vi "01 Dryer_Performance_SM.vi"() -> ()   [LabVIEW 2016]
uses:
  Utility/Save File/File Setup (Public)/DPT Global Test Variables.vi
  Utility/Save File/File Setup.lvlib
  Type Definitions/RMC Calc Inputs.ctl
  Nufi/Nufi Global_ReceivedDataCluster.vi
  Type Definitions/Q Dryer Data.ctl
  Drivers/Yokogawa WT500/Type Definitions/WT500 Sequences.ctl
  Drivers/Chroma 617xx/Type Definition/Chroma Driver Select.ctl
  Type Definitions/Equipment DPT.ctl
  <vilib>/Analysis/NI_AALBase.lvlib
  <vilib>/Analysis/baseanly.llb/Mean (DBL).vi
  Utility/Type Definitions/UTILITY Power Inputs Control.ctl
  Utility/Custom Pallet Controls/Custom Pallet DBL.ctl
  <vilib>/Platform/fileVersionInfo.llb/FileVersionInformation.ctl
  Utility/Save File/File Setup (Public)/Type Definition/DPT Global Type.ctl
  Utility/Type Definitions/UTILITY Power Analyzer.ctl
  Utility/Custom Pallet Controls/Custom Pallet Quit.ctl
  Utility/Custom Pallet Controls/Custom Pallet Timer.ctl
  Utility/Save File/File Setup (Public)/Type Definition/DPT Output Dryer Information.ctl
  Utility/Custom Pallet Controls/Custom Pallet Configuration.ctl
  Utility/Custom Pallet Controls/Custom Pallet Reverse.ctl
  Utility/Custom Pallet Controls/Custom Pallet String.ctl
  Utility/Custom Pallet Controls/Custom Pallet Chart.ctl
  Drivers/cDAQ/Type Definitions/cDAQ Setup.ctl
panel:
  out "cDAQ Data Out":string[](array[string])
  out "Indexes used":i32[](array[numeric])
  in  "Setup":T1={"Test Setup"={"RH Resistor"=100.0, "Temp Resistor"=100.0, "Gas P. Resistor"=250.0, "Temp4mA Val"=32.0, "Temp20mA Val"=212.0, "RH4mA Val"=0.0, "RH20mA Val"=100.0, "GPres4mA Val"=0.0, "Gpres20mA Val"=50.0}, "cDAQ Array Locations"={"Scale Channel"=90, "TC Channels"=0, "VDC Discrete Channel"=72, "RH Chan"=91, "Temp Chan"=93, "Tscale Channel"=2, "RDB Channel"=0, "Gas Temperature"=88, "Gas Pressure"=89, "Barometric Pressure"=94, "Gas Feedback Chan"=92}}
  in  "Weight Offset 2":dbl
  in  "W.Samps 2":i32=10
  out "Status Message":T2
  in  "Back Button":T3
  in  "Settings":T4
  in  "End Test":T5
  out "2015 array":string[][](array[string])
  out "FileInit Cluster":T6={"Dryer Type"="NR", "TR Number"="", "Lab ID"="", "Output Stream Header"=[], "Stream Data Output"=[], "2015 Array"=[], "Dryer Test Data"=[], "Off Mode Array"=[], "Calibration Array"=[], "File Initialization Array"=[], "Load Run Number"="", "Model:"="DGnn", "Serial Number:"="DGnn", "Build:"="", "Test_Title Per TR:"="HeatUP", "Ambient Temp SetPoint:"="70", "Washer Water \nTemperature ( 60 ± 5°F ):"="60", "Frequency:"="60 HZ", "Dryness Setting:"="", "Heat Setting:"="", "Ambient RH:"="50", "Drying Cycle:"="", "Exhaust:"="NR", "Comments:"="", "Technician:"="", "Engineer:"="CraigT.", "Water Hardness (PPM)"="60", "Empty Dryer Cold Weight"="HeatUP", "Date:"="DGnn", "Version:"="DGnn", "Computer:"="1A", "Load Type"="", "Nominal Load  Weight"="", "Weights Out"={"Measured IMC"=7.0, "Actual RMC"=7.0, "RMC (Desired)"=100.0, "Bone Dry Wt(lbs)"=7.0, "Tolerance(%)"=5.0}, "Test Station:"="1A", "Heat Setting:"="", "Dryness Setting:"="", "Frequency:"="60 HZ", "Water Hardness (PPM)"="60", "Washer Water \nTemperature ( 60 ± 5°F )"="60", "Flow Computer Info Baro,BTUF,u,Z"=[], "Filename"="", "Analog Voltage Data"=[]} {"Weights Out"."Tolerance(%)" format="%0#_6g"; "Weights Out"."Bone Dry Wt(lbs)" format="%03_6g"; "Weights Out"."RMC (Desired)" format="%0#_6g"; "Weights Out"."Actual RMC" format="%03_6g"; "Weights Out"."Measured IMC" format="%0#_6g"}
  out "Plot Power":cluster{dbl[], dbl[]}[](graph)
  in  "Quit":T5
  out "Power Out":T7={"Yokogawa"={"WT210"={"Sample Rate (1: 0.25s)"=1, "A Range (12: 20A)"=11, "V Range (6: 600V)"=4, "Power VISA Yokogawa WT210"=""}, "WT500"={"Power VISA Yokogawa WT500"="", "V Range (8: 1000V)"=6, "I Range (7: 40A)"=7, "Update Rate (3: 500ms)"=2}}, "Aplus"={"Aplus IP Address"="192.168.1.101", "Remote Port"=502, "Instrument"="APLUS", "Instr Driver Revision"="1.03.0053"}, "Power Limits"={"Crest Factor"={"Upper Limit"=1.49, "Lower Limit"=1.34}, "Harmonic Content"={"Uthd"=2.0}, "Voltage"={"% Error"=2.0}, "Stability"={"<1 Watt "={"Wattage"=1.0, "Slope (mW/H)"=10.0}, ">1 Watt"={"1%Power/Hour"=1.0}}}, "Nominal Voltage"=120, "Time Limit (s)"=10800.0, "Power Variation Limit (%)"=50.0, "Power Supply"={"Chroma 61605"="CHROMA", "Use Chroma?"=FALSE}} {"Yokogawa"."WT500"."Update Rate (3: 500ms)" items=["-", "100ms", "200ms", "500ms", "1s", "2s", "5s"]; "Yokogawa"."WT500"."I Range (7: 40A)" items=["AUTO", "500 mA", "1 A", "2 A", "5 A", "10 A", "20 A", "40 A", "S-AUTO", "50 mV", "100 mV", "200 mV", "500 mV", "1 V", "2 V", "5 V", "10 V", "250 mA", "500 mA", "1 A", "2.5 A", "5 A", "10 A", "20 A", "25 mV", "50 mV", "100 mV", "250 mV", "500 mV", "1 V", "2.5 V", "5 V"]; "Yokogawa"."WT500"."V Range (8: 1000V)" items=["AUTO", "15", "30", "60", "100", "150", "300", "600", "1000", "7.5", "15", "30", "50", "75", "150", "300", "500"]; "Yokogawa"."WT210"."V Range (6: 600V)" items=["Auto", "15V", "30V", "60V", "150V", "300V", "600V"]; "Yokogawa"."WT210"."A Range (12: 20A)" items=["Auto", "5mA", "10mA", "20mA", "50mA", "100mA", "200mA", "0.5A", "1A", "2A", "5A", "10A", "20A", "50mV", "100mV", "200mV", "2.5V", "5V", "10V"]; "Yokogawa"."WT210"."Sample Rate (1: 0.25s)" items=["0.1s", "0.25s", "0.5s", "1s", "2s", "5s"]}
  in  "Voltage Stream Header Output":string[][](array[string])
  in  "Stream Data":string[][](array[string])
  in  "Tab Control 3":enum32{"Page 1", "Page 2", "Page 3", "Page 4"}(tab)
  out "Equipment":T8={"Scale Com Port"="", "Com Flow Computer"="", "Com Power Meter"="", "Com Power Supply"="", "Power "={"Yokogawa"={"WT210"={"Sample Rate (1: 0.25s)"=1, "A Range (12: 20A)"=11, "V Range (6: 600V)"=4, "Power VISA Yokogawa WT210"=""}, "WT500"={"Power VISA Yokogawa WT500"="", "V Range (8: 1000V)"=6, "I Range (7: 40A)"=7, "Update Rate (3: 500ms)"=2}}, "Aplus"={"Aplus IP Address"="192.168.1.101", "Remote Port"=502, "Instrument"="APLUS", "Instr Driver Revision"="1.03.0053"}, "Power Limits"={"Crest Factor"={"Upper Limit"=1.49, "Lower Limit"=1.34}, "Harmonic Content"={"Uthd"=2.0}, "Voltage"={"% Error"=2.0}, "Stability"={"<1 Watt "={"Wattage"=1.0, "Slope (mW/H)"=10.0}, ">1 Watt"={"1%Power/Hour"=1.0}}}, "Nominal Voltage"=120, "Time Limit (s)"=10800.0, "Power Variation Limit (%)"=50.0, "Power Supply"={"Chroma 61605"="CHROMA", "Use Chroma?"=FALSE}}} {"Power"."Yokogawa"."WT500"."Update Rate (3: 500ms)" items=["-", "100ms", "200ms", "500ms", "1s", "2s", "5s"]; "Power"."Yokogawa"."WT500"."I Range (7: 40A)" items=["AUTO", "500 mA", "1 A", "2 A", "5 A", "10 A", "20 A", "40 A", "S-AUTO", "50 mV", "100 mV", "200 mV", "500 mV", "1 V", "2 V", "5 V", "10 V", "250 mA", "500 mA", "1 A", "2.5 A", "5 A", "10 A", "20 A", "25 mV", "50 mV", "100 mV", "250 mV", "500 mV", "1 V", "2.5 V", "5 V"]; "Power"."Yokogawa"."WT500"."V Range (8: 1000V)" items=["AUTO", "15", "30", "60", "100", "150", "300", "600", "1000", "7.5", "15", "30", "50", "75", "150", "300", "500"]; "Power"."Yokogawa"."WT210"."V Range (6: 600V)" items=["Auto", "15V", "30V", "60V", "150V", "300V", "600V"]; "Power"."Yokogawa"."WT210"."A Range (12: 20A)" items=["Auto", "5mA", "10mA", "20mA", "50mA", "100mA", "200mA", "0.5A", "1A", "2A", "5A", "10A", "20A", "50mV", "100mV", "200mV", "2.5V", "5V", "10V"]; "Power"."Yokogawa"."WT210"."Sample Rate (1: 0.25s)" items=["0.1s", "0.25s", "0.5s", "1s", "2s", "5s"]}
  in  "Power Analyzer":T9=enum."WT500"
  in  "Data Save Array":string[][](array[string])
  out "Off Mode Power Output":string[][](array[string])
  out "Error after create directory":errorcluster
  out "Error after save to excel":errorcluster
  out "Error before create directory":errorcluster
  out "Error":errorcluster[](array[cluster])
  out "Tsamp(s)":dbl
  in  "Tab Control":T10(tab)
  out "Wbouy":dbl
  out "Plot RMC":cluster{dbl[], dbl[]}[](graph)
  out "Experimental Completion Time Estimate":dbl format="%<%H:%M:%S>t"
  out "RMC Chart":T11
  out "Watt Chart":dbl(graph)
  out "Relative Moisture Content (%)":T12 format="%.2f"
  out "Scale Weight (lbs)":T12 format="%.2f"
  out "RDB Temperature (Degrees F)":T12 format="%.2f"
  out "Room Ambient (Degrees F)":T12 format="%.2f"
  out "Cloth Weight Estimate (lbs)":T12 format="%.2f"
  out "Wet Clothing Weight (lbs)":T12 format="%.2f"
  out "Empty Dryer Cold Weight (lbs)":T12 format="%.2f"
  out "Bone Dry Weight (lbs)":T12 format="%.2f"
  out "Watt Hours (Wh)":T12 format="%.2f"
  out "Power (Watts)":T12 format="%.2f"
  out "Current L2 (A)":T12 format="%.2f"
  out "Current L1 (A)":T12 format="%.2f"
  out "Power ON":bool
  out "Description":string="Dryer Performance Test"
  out "Test Time":T13 format="%<%H:%M:%S>t"
  in  "Tab Control 2":enum32{"Debug Only", "Running"}(tab)
  in  "Debug Info":T14(tab)=enum."Settings"
  out "FileName DataLog":path caption="FileName"
  out "FileVersionInfo Out":T15
  out "Ver.":string="Development"
  out "Work File Directory":path=path "c:/Work"
  in  "Close when complete":bool
  in  "Standby Power Settings":path=path "C:/work/Standby Power Settings.csv"
  in  "Excel Template Path":path=path "C:/work/DOE Calculation Template for 2015 DOE ETP Rev4.xlsx"
  out "Created File Path":path
  in  "Error Log 2":errorcluster[](array[cluster])
  out "Power Off Check":bool[](array[boolean])
  out "error out":errorcluster
  out "Error Count":dbl
  out "# elements in queue":i32
  out "Error Log":errorcluster[](array[cluster])
  out "Data Filename":string
  out "Power Off Time(samples)":i32=15
  in  "UI Timer":i32=1000
  in  "DAQ Timer":i32=1000
  in  "Clear Graph":bool
  out "Use SL9200 Gas Readings?":bool
  in  "Simulate":bool
  in  "Supply Voltage:":string(combo)
  out "Time Limit(s)":dbl=5400.0 format="%<%H:%M:%S>t"
  out "RMC Limit":dbl=2.0
  out "Enable Time Limit":bool
  out "Enable RMC Limit":bool
  in  "MA Filter Size":i32=10
  in  "Power On Threshold":dbl=50.0
  in  "Scale Temp Coeff":dbl
  out "Init Scale Temp":dbl=72.0
  out "Use Dry Gas Meter?":bool=TRUE
  out "Load Offset":dbl
  in  "Drum Volume":dbl=6.0
  out "Enable Stop On Power Off":bool=TRUE
  out "exe?":bool
  out "RMC Calc Inputs":T16
  out "Tend?":dbl format="%<%H:%M:%S>t"
  out "Scale Com Port":refnum<visa-resource-name>="COM1"
  out "ITHX RH Sensor":bool
  out "Offset":dbl
  out "Init Offset Coeff":dbl
  in  "Power off Check RMC sec":dbl=5.0
  out "DAQ Delay Time":i32
  out "Data Process RMC Counter":dbl
  out "L1 Adjusted":string
  out "L2 Adjusted":string
  out "Debug Mode":bool=TRUE
  out "Debug List Test States":string[](array[string])
  out "daq debug array":string[](array[string])
  out "UI States":string[](array[string])
  out "End1_Main":bool=TRUE
  out "Write to File":bool=TRUE
  out "Test Complete?":bool
  out "Loggin Data":bool
  out "End2_DAQ":bool=TRUE
  out "Eng3_Log":bool=TRUE
  out "BTUF3":string[][](array[string])
  out "Power On One Shot":bool
  out "End Msg":string
  out "Final User Message":string="Premature Completion."
  out "cDAQ":bool=TRUE
  in  "cDAQ Setting":bool=TRUE
  out "End_End":bool=TRUE
  in  "CDAQ Tasks":refnum<k21>[](array[refnum])
  out "[Temp (F), RH]":dbl[](array[numeric])
  out "Power Off One Shot":bool
  out "Elapsed Time":T13 format="%<%H:%M:%S>t"
  out "Start Time (sec)":T13 format="%<%H:%M:%S>t"
  out "Power >Threshold":bool
  out "TC Channel List":string
  out "DAQ Channel List":string
  out "DAQ Label List":string[](array[string])
  in  "Get Data Interrupt":bool
  out "Use Chroma":bool
  out "Number of TCs":i32
  out "Stream DC to File?":bool
  out "Globals for Dryer Performance Test":T17={"Test Setup"={"RH Resistor"=267.4, "Temp Cal"=72.0, "Temp Coeff"=-0.0234, "Power On Threshold"=50.0, "MA Filter Size"=60, "Weight Offset"=0.0, "Temp Resistor"=267.4, "Gas Enabled"=FALSE, "Gas P. Resistor"=250.0, "Scale Com"=1.0, "W. Samps"=5, "Temp4mA Val"=267.4, "Temp20mA Val"=267.4, "RH4mA Val"=0.0, "RH20mA Val"=100.0, "GPres4mA Val"=0.0, "Gpres20mA Val"=50.0, "Smoothing"=FALSE, "CDAQ"=FALSE, "34970"=FALSE, "34980"=FALSE, "RH-IP"="192.168.1.161", "RH-IP2"="192.168.1.161", "RH-IP3"="192.168.1.161", "CompVolume"=0.0, "T45_Coeff."=0.0}, "Agilent Setup"={"Scale Channel"="3009", "TC Channels"="1001:1040,2001:2040", "VDC Discrete Channels"="3001:3008", "RH Chan"="3010,3011", "Temp Chan"="3010,3011", "Tscale Channel"="", "RDB Channel"="1001", "Gas Temperature"="1019", "Gas Pressure"="1020", "Barometric Pressure"="1040", "Gas Feedback Chan"="3012"}, "Directories"={"Work File Directory"=path "c:/Work", "Save File Directory"=path "c:/Data", "Library Directory"=path "c:/Data", "Data Backup Directory"=path "c:/Data", "Data Backup Dir Fail"=path "c:/Data", "Lab Directory"=path "c:/Data"}, "Test Information"={"Model:"="DGnn", "Temperature:"="Mode: EHEAT", "Engineer:"="CraigT.", "Technician:"="RonR.", "Comments:"="R134A Charge Level: 50g", "Lab ID:"="DGnn", "TR Number:"="T000000", "Test Number:"="T000000", "Test Station:"="Unitialized", "Empty Dryer Cold Weight:"=0.0, "Serial Number:"="DGnn", "Build:"="DGnn", "Dryer Type"="RonR.", "Humidity"="70,50", "Test Title per TR:"="70,50"}, "cDAQ Array Locations"={"Scale Channel"="90", "TC Channels"="1-15, 65,66,67\n16-31, 68,69\n32-47, 70,71\n48-64, 72, 73", "VDC Discrete Channel"="1020,1040,3001:3008", "RH Chan"="91", "Temp Chan"="93", "Tscale Channel"="3", "RDB Channel"="1", "Gas Temperature"="0", "Gas Pressure"="89", "Barometric Pressure"="94", "Gas Feedback Chan"="92"}}
  out "Plot All":cluster{dbl[], dbl[]}[](graph)
  in  "Apply Load Offset":bool
  out "Use Smoothing":bool=TRUE
  out "2015?":bool
  out "Data":string[][](array[string])
  in  "Plot Legend":T18(array[cluster])
  in  "None":bool
  in  "All":bool
  out "Power Label":string[](array[string])=["VL1", "VL2", "IL1", "IL2", "P", "WH", "Ipeak", "Phi(1,2)"]
  out "Q Element":T19
  in  "Start Test":bool
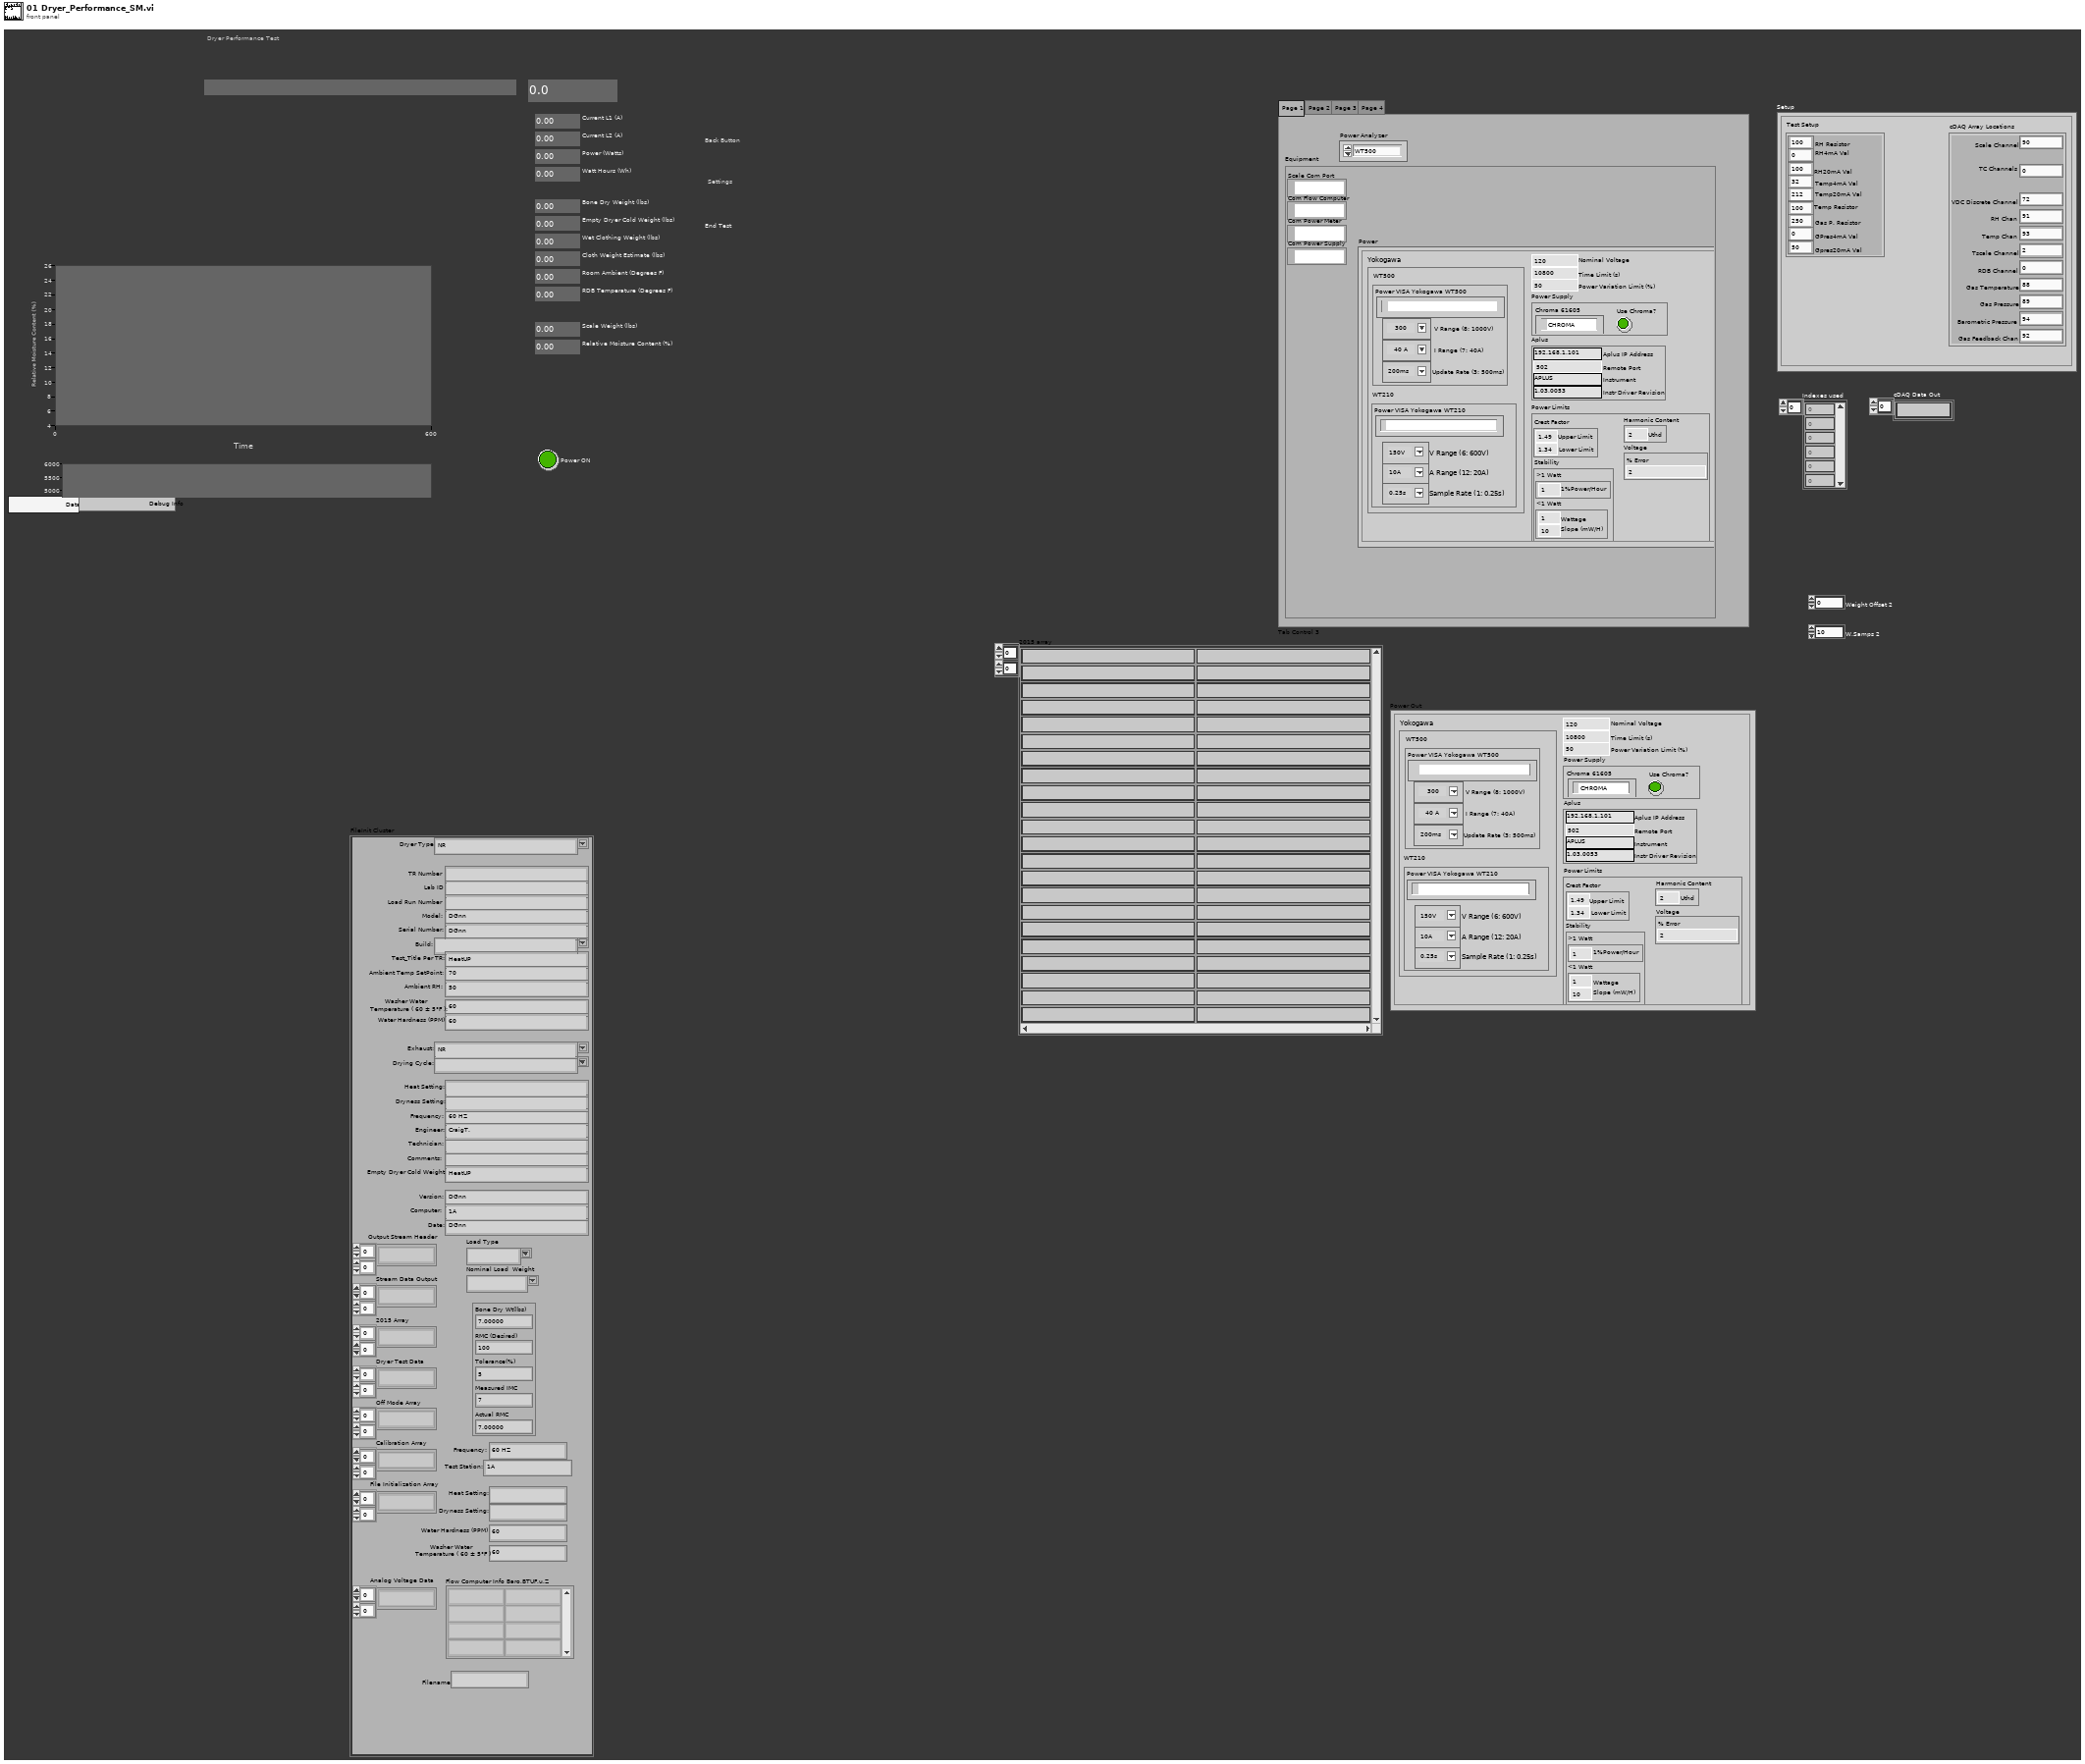
[diagram p1: front panel]
types:
  T1 = typedef "cDAQ Setup.ctl" = cluster{"Test Setup":cluster{"RH Resistor":dbl, "Temp Resistor":dbl, "Gas P. Resistor":dbl, "Temp4mA Val":dbl, "Temp20mA Val":dbl, "RH4mA Val":dbl, "RH20mA Val":dbl, "GPres4mA Val":dbl, "Gpres20mA Val":dbl}, "cDAQ Array Locations":cluster{"Scale Channel":i32, "TC Channels":i32, "VDC Discrete Channel":i32, "RH Chan":i32, "Temp Chan":i32, "Tscale Channel":i32, "RDB Channel":i32, "Gas Temperature":i32, "Gas Pressure":i32, "Barometric Pressure":i32, "Gas Feedback Chan":i32}}
  T2 = typedef "Custom Pallet String.ctl" = string
  T3 = typedef "Custom Pallet Reverse.ctl" = bool
  T4 = typedef "Custom Pallet Configuration.ctl" = bool
  T5 = typedef "Custom Pallet Quit.ctl" = bool
  T6 = typedef "File Setup.lvlib/DPT Output Dryer Information.ctl" = cluster{"Dryer Type":string, "TR Number":string, "Lab ID":string, "Output Stream Header":string[][], "Stream Data Output":string[][], "2015 Array":string[][], "Dryer Test Data":string[][], "Off Mode Array":string[][], "Calibration Array":string[][], "File Initialization Array":string[][], "Load Run Number":string, "Model:":string, "Serial Number:":string, "Build:":string, "Test_Title Per TR:":string, "Ambient Temp SetPoint:":string, "Washer Water \nTemperature ( 60 ± 5°F ):":string, "Frequency:":string, "Dryness Setting:":string, "Heat Setting:":string, "Ambient RH:":string, "Drying Cycle:":string, "Exhaust:":string, "Comments:":string, "Technician:":string, "Engineer:":string, "Water Hardness (PPM)":string, "Empty Dryer Cold Weight":string, "Date:":string, "Version:":string, "Computer:":string, "Load Type":string, "Nominal Load  Weight":string, "Weights Out":cluster{"Measured IMC":dbl, "Actual RMC":dbl, "RMC (Desired)":dbl, "Bone Dry Wt(lbs)":dbl, "Tolerance(%)":dbl}, "Test Station:":string, "Heat Setting:":string, "Dryness Setting:":string, "Frequency:":string, "Water Hardness (PPM)":string, "Washer Water \nTemperature ( 60 ± 5°F )":string, "Flow Computer Info Baro,BTUF,u,Z":string[][], "Filename":string, "Analog Voltage Data":string[][]}
  T7 = typedef "UTILITY Power Inputs Control.ctl" = cluster{"Yokogawa":cluster{"WT210":cluster{"Sample Rate (1: 0.25s)":i32, "A Range (12: 20A)":i32, "V Range (6: 600V)":i32, "Power VISA Yokogawa WT210":refnum<visa-resource-name>}, "WT500":cluster{"Power VISA Yokogawa WT500":refnum<visa-resource-name>, "V Range (8: 1000V)":i32, "I Range (7: 40A)":i32, "Update Rate (3: 500ms)":i32}}, "Aplus":cluster{"Aplus IP Address":string, "Remote Port":i32, "Instrument":string, "Instr Driver Revision":string}, "Power Limits":cluster{"Crest Factor":cluster{"Upper Limit":dbl, "Lower Limit":dbl}, "Harmonic Content":cluster{"Uthd":dbl}, "Voltage":cluster{"% Error":dbl}, "Stability":cluster{"<1 Watt ":cluster{"Wattage":dbl, "Slope (mW/H)":dbl}, ">1 Watt":cluster{"1%Power/Hour":dbl}}}, "Nominal Voltage":i32, "Time Limit (s)":dbl, "Power Variation Limit (%)":dbl, "Power Supply":cluster{"Chroma 61605":refnum<visa-resource-name>, "Use Chroma?":bool}}
  T8 = typedef "Equipment DPT.ctl" = cluster{"Scale Com Port":refnum<visa-resource-name>, "Com Flow Computer":refnum<visa-resource-name>, "Com Power Meter":refnum<visa-resource-name>, "Com Power Supply":refnum<visa-resource-name>, "Power ":T7}
  T9 = typedef "UTILITY Power Analyzer.ctl" = enum16{"", "APLUS", "WT210", "WT500", "WT300", "OSI", "Debug", "WT230"}
  T10 = enum32{"                           Data  ", "                                  Debug Info"}
  T11 = typedef "Custom Pallet Chart.ctl" = dbl
  T12 = typedef "Custom Pallet DBL.ctl" = dbl
  T13 = typedef "Custom Pallet Timer.ctl" = dbl
  T14 = enum32{"File Info", "Error Data", "Settings", "Test States", "NI CDAQ Data", "Globals"}
  T15 = typedef "FileVersionInformation.ctl" = cluster{"FileVersion":string, "ProductName":string, "InternalName":string, "CompanyName":string, "LegalCopyright":string, "FileDescription":string}
  T16 = typedef "RMC Calc Inputs.ctl" = cluster{"Measeured Weight":dbl, "BDW - Bone Dry Wt(lbs)":dbl, "Empty Dryer Cold Weight":dbl, "Measured IMC":dbl, "Tamb":dbl, "T-RDB":dbl, "Drum Volume":dbl, "Load Offset":dbl, "Temp Coeff":dbl, "Temp Cal":dbl, "Tscale":dbl}
  T17 = typedef "File Setup.lvlib/DPT Global Type.ctl" = cluster{"Test Setup":cluster{"RH Resistor":dbl, "Temp Cal":dbl, "Temp Coeff":dbl, "Power On Threshold":dbl, "MA Filter Size":i32, "Weight Offset":dbl, "Temp Resistor":dbl, "Gas Enabled":bool, "Gas P. Resistor":dbl, "Scale Com":dbl, "W. Samps":i32, "Temp4mA Val":dbl, "Temp20mA Val":dbl, "RH4mA Val":dbl, "RH20mA Val":dbl, "GPres4mA Val":dbl, "Gpres20mA Val":dbl, "Smoothing":bool, "CDAQ":bool, "34970":bool, "34980":bool, "RH-IP":string, "RH-IP2":string, "RH-IP3":string, "CompVolume":dbl, "T45_Coeff.":dbl}, "Agilent Setup":cluster{"Scale Channel":string, "TC Channels":string, "VDC Discrete Channels":string, "RH Chan":string, "Temp Chan":string, "Tscale Channel":string, "RDB Channel":string, "Gas Temperature":string, "Gas Pressure":string, "Barometric Pressure":string, "Gas Feedback Chan":string}, "Directories":cluster{"Work File Directory":path, "Save File Directory":path, "Library Directory":path, "Data Backup Directory":path, "Data Backup Dir Fail":path, "Lab Directory":path}, "Test Information":cluster{"Model:":string, "Temperature:":string, "Engineer:":string, "Technician:":string, "Comments:":string, "Lab ID:":string, "TR Number:":string, "Test Number:":string, "Test Station:":string, "Empty Dryer Cold Weight:":dbl, "Serial Number:":string, "Build:":string, "Dryer Type":string, "Humidity":string, "Test Title per TR:":string}, "cDAQ Array Locations":cluster{"Scale Channel":string, "TC Channels":string, "VDC Discrete Channel":string, "RH Chan":string, "Temp Chan":string, "Tscale Channel":string, "RDB Channel":string, "Gas Temperature":string, "Gas Pressure":string, "Barometric Pressure":string, "Gas Feedback Chan":string}}
  T18 = cluster{"Title":string, "OnOff":bool, "Color Box":u32, "Value":dbl}[]
  T19 = typedef "Q Dryer Data.ctl" = cluster{"Data Array":dbl[], "Data":string[][], "Date":string}
  T20 = enum32{"invalid app kind", "Development System", "Run Time System", "Student Edition", "Embedded LabVIEW", "Evaluation", "Custom"}
  T21 = enum16{"Exe", "Init CDAQ", "Gather DATA", "Close"}
  T22 = typedef "Chroma Driver Select.ctl" = enum16{"Initialize", "Output On 120", "Output On 240", "Output On 208", "Output Off", "Status", "Send Command", "Track Current"}
  T23 = enum32{"Invalid", "Standard", "Closed", "Hidden", "Minimized", "Maximized"}
  T24 = cluster{"Core":cluster{"Current VI Reference":refnum<vi>, "Close Panel on Exit?":bool}, "Error Log":errorcluster[], "FileName":path, "Config File Path":path, "Standby Power Settings":path, "Equipment":T8, "DAQ Chan List":string, "DAQ Label List":string[], "Supply Voltage:":string, "Empty Dryer Cold Weight":dbl, "Start Header Data":string[][], "Dryer Type":string, "Dryer Load Nominal Weight":string, "Power Analyzer":T9, "CDAQ Tasks":refnum<k21>[]}
  T25 = typedef "File Setup.lvlib/DPT Audit Data.ctl" = cluster{"Technician":string, "Date":string, "Model":string, "Serial":string, "Total Dry Time(m)":dbl, "Bone Dry Wt":dbl, "Initial Wt":dbl, "Final Wt":dbl, "Initial Ret":dbl, "Final Ret":dbl, "Elect Energy Used":dbl, "Gas Meter Temp":dbl, "Gas Meter Pres":dbl, "Gas Volume":dbl, "Barometer Temp":dbl, "Barometer Pres":dbl, "Gas Corr Fact":dbl, "Cor Gas Vol":dbl, "Gas Heat Val":dbl, "Gas Energy BTU":dbl, "Gas Energy kwh 4%":dbl, "Elect Energy kwh 4%":dbl, "Total  Energy 4%":dbl, "Gas Vol Init":dbl, "Gas Vol Fin":dbl, "Start Time(s)":dbl, "End Time(s)":dbl, "Elect Energy Start":dbl, "Elect Energy End":dbl, "Per Cycle Efficency":dbl, "Annual Consumption":dbl, "Load Cycles":string, "Ambinet Temp":string, "Ambinet RH":string, "Per Cycle Off Mode/Standby Power":dbl, "Total Energy (Gas + Elect)":dbl, "Combined Energy Factor":dbl, "Off Mode Power":dbl, "Exhaust":string, "Washer Water Temperature ( 60 ± 5°F )":string, "Supply Voltage":string, "Reference Temperature (F)":string, "Reference Pressure (psi)":string, "Standby Power":dbl}
  T26 = typedef "UTILITY Power Data.ctl" = cluster{"Irms:Element 1":dbl, "Irms:Element 2":dbl, "P:Sigma":dbl, "Wp:Sigma":dbl, "Urms:Element 2":dbl, "Urms:Element 1":dbl, "Cf I:Element 1":dbl, "Cf I:Element 2":dbl, "Uthd:Element 1":dbl, "Uthd:Element 2":dbl, "Cf U:Element 1":dbl, "Cf U:Element 2":dbl, "Time:Element 1":dbl, "Freq U:Element 1":dbl, "S:Element 1":dbl, "S:Element 2":dbl, "Lambda:Element 1":dbl, "Lambda:Element 2":dbl, "Max Watt Hours":dbl, "Urms:Element 2 Avg":dbl, "Urms:Element 1 Avg":dbl}
  T27 = cluster{"Temp/Humidity[0]":dbl, "Temp/Humidity[1]":dbl}
  T28 = cluster{"Measured IMC":dbl, "Actual RMC":dbl, "RMC (Desired)":dbl, "Bone Dry Wt(lbs)":dbl, "Tolerance(%)":dbl}
  T29 = cluster{"Current VI Reference":refnum<vi>, "Close Panel on Exit?":bool}
  T30 = typedef "WT500 Sequences.ctl" = enum16{"Initialize", "GetReadings", "GetErrors", "Close", "NoOp", "MiscCmd"}
  T31 = cluster{"queue out":refnum<queue>, "Q Element":T19, "Equipment":T8, "DAQ Channel List":string, "Error Log 2":errorcluster[], "Stream Data":string[][], "Voltage Stream Header Output":string[][]}
  T32 = typedef "WT500 Dryer Power Data.ctl" = cluster{"Current L1":dbl, "Current L2":dbl, "Power":dbl, "WattHours":dbl}
  T33 = cluster{"queue out":refnum<queue>, "Q Element":T19, "Graph Reset":bool, "Init Save File":bool, "Time Array":dbl[], "Data Array":dbl[][], "Enable RMC":bool, "Power Previous":bool, "Data Save Array":string[][], "Excel Template Path":path}
  T34 = cluster{"Title":string, "OnOff":bool, "Color Box":u32, "Value":dbl}
  T35 = cluster{"[0]":dbl, "[1]":dbl, "[2]":dbl, "[3]":dbl, "[4]":dbl, "[5]":dbl}
  T36 = cluster{"[0]":dbl, "[1]":dbl, "[2]":dbl, "[3]":dbl}
  T37 = enum16{"Left Button", "Center Button", "Right Button", "Window Close"}
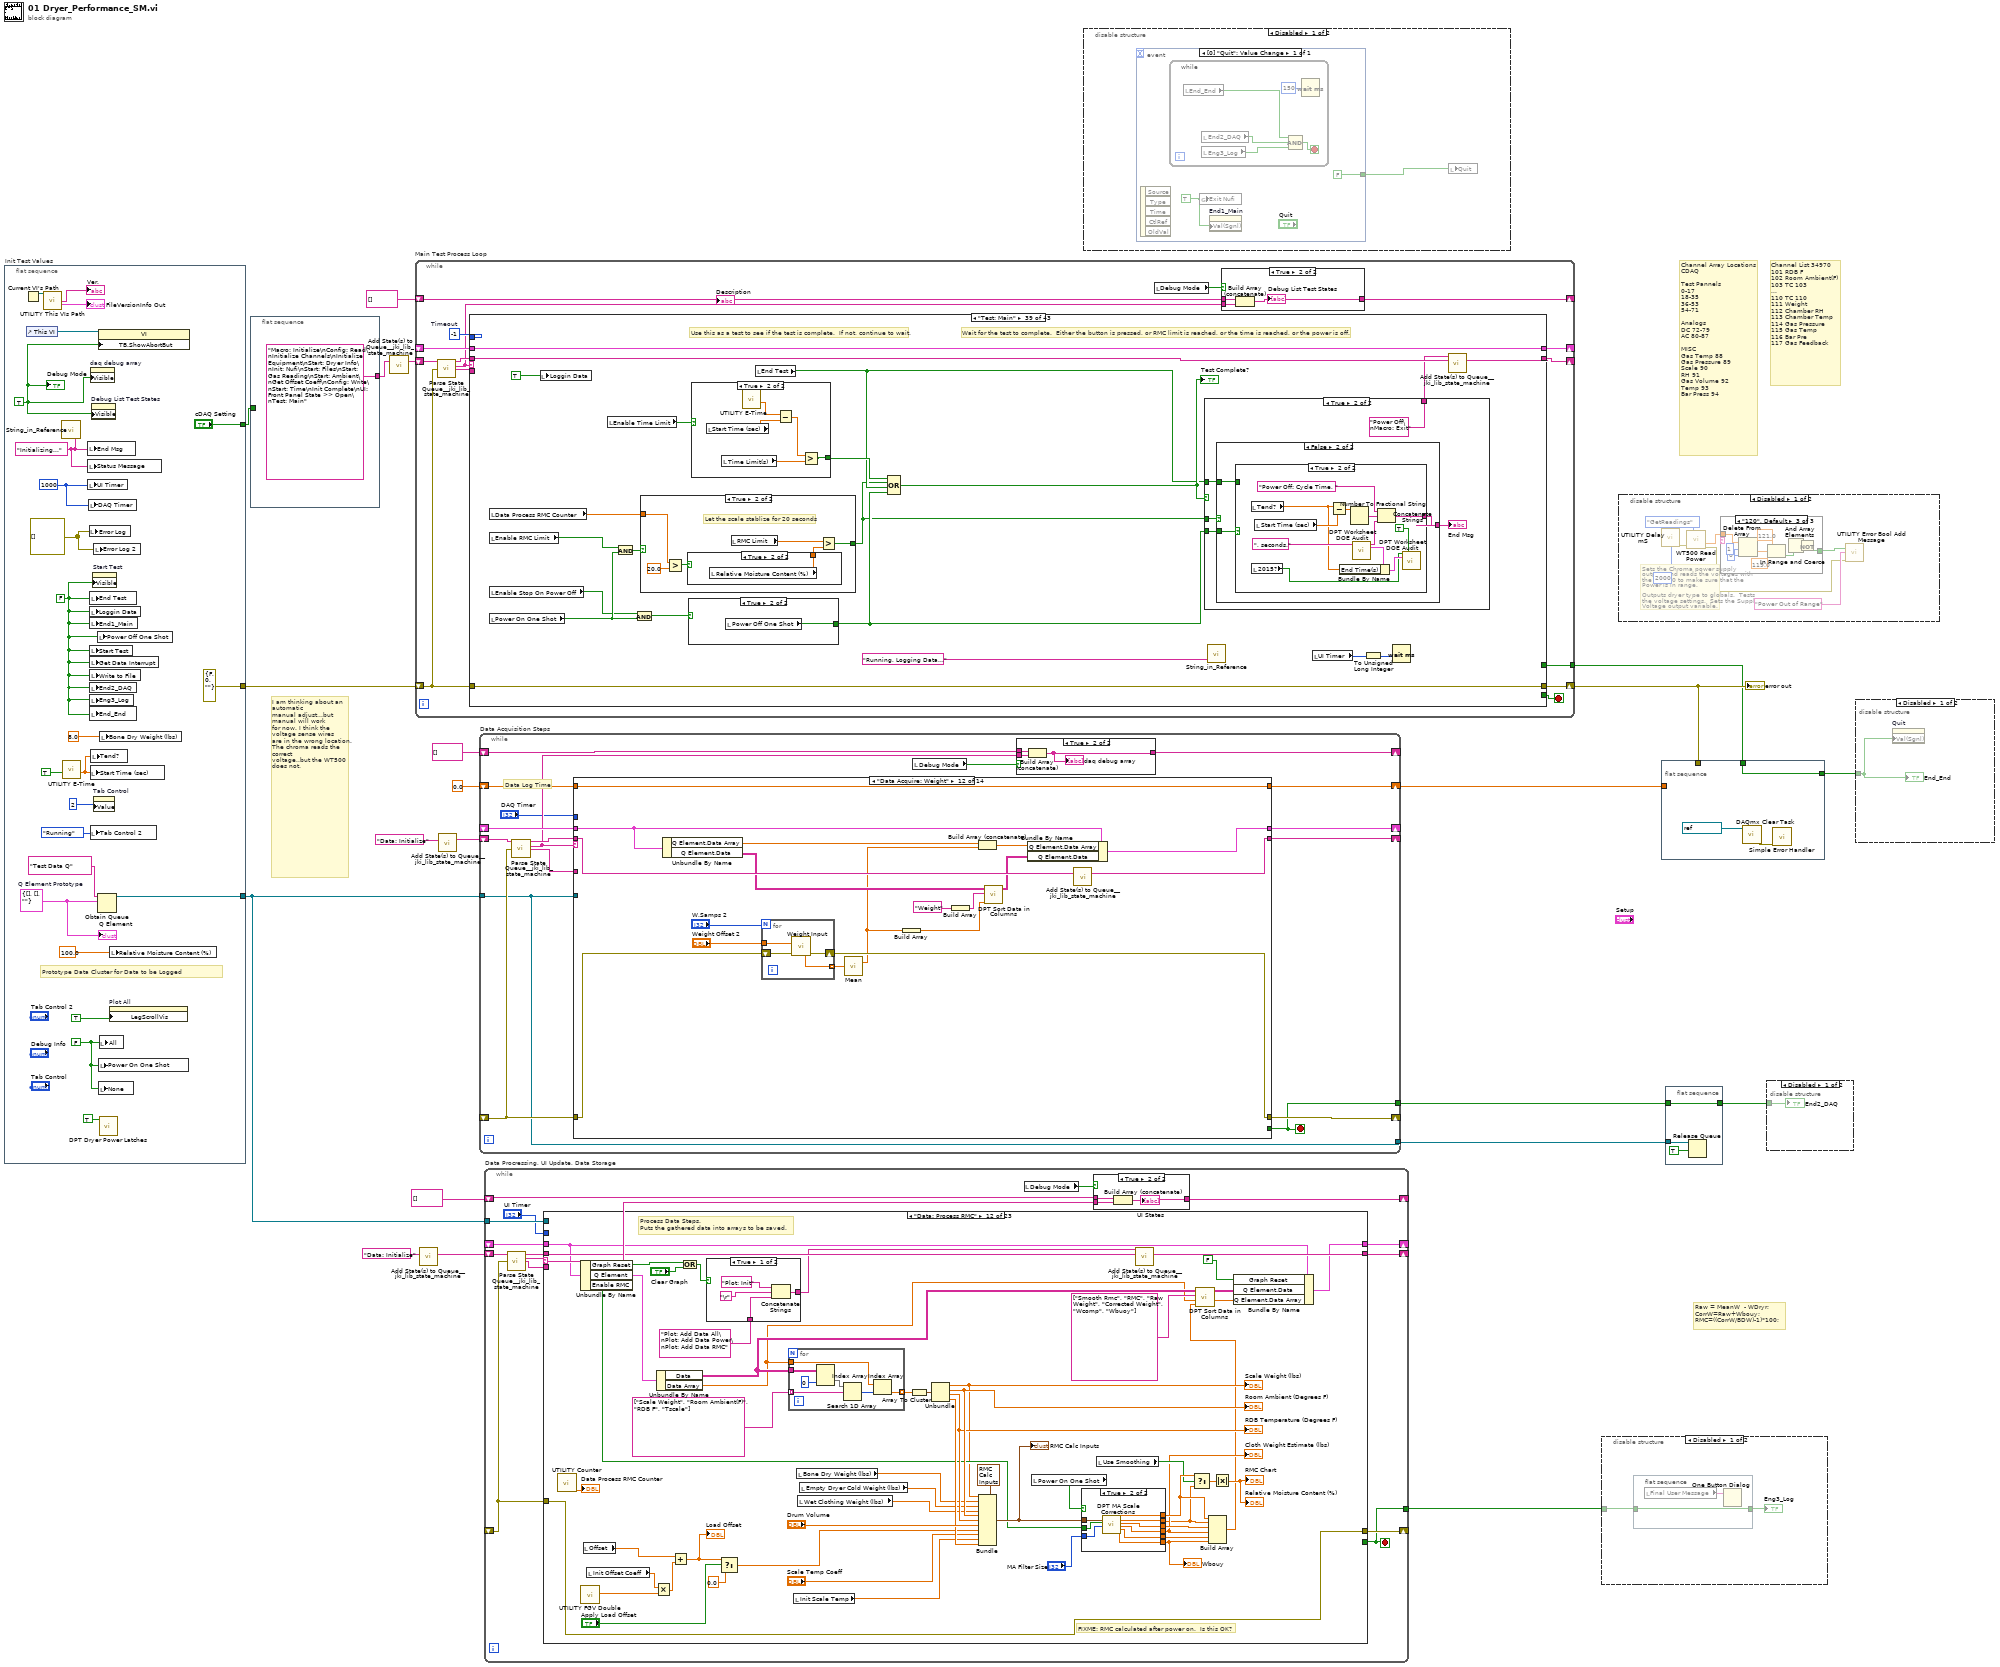
[diagram p0: block diagram]
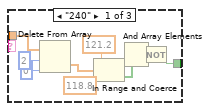
[diagram p6: hidden frame]
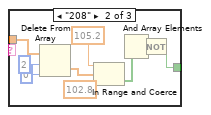
[diagram p7: hidden frame]
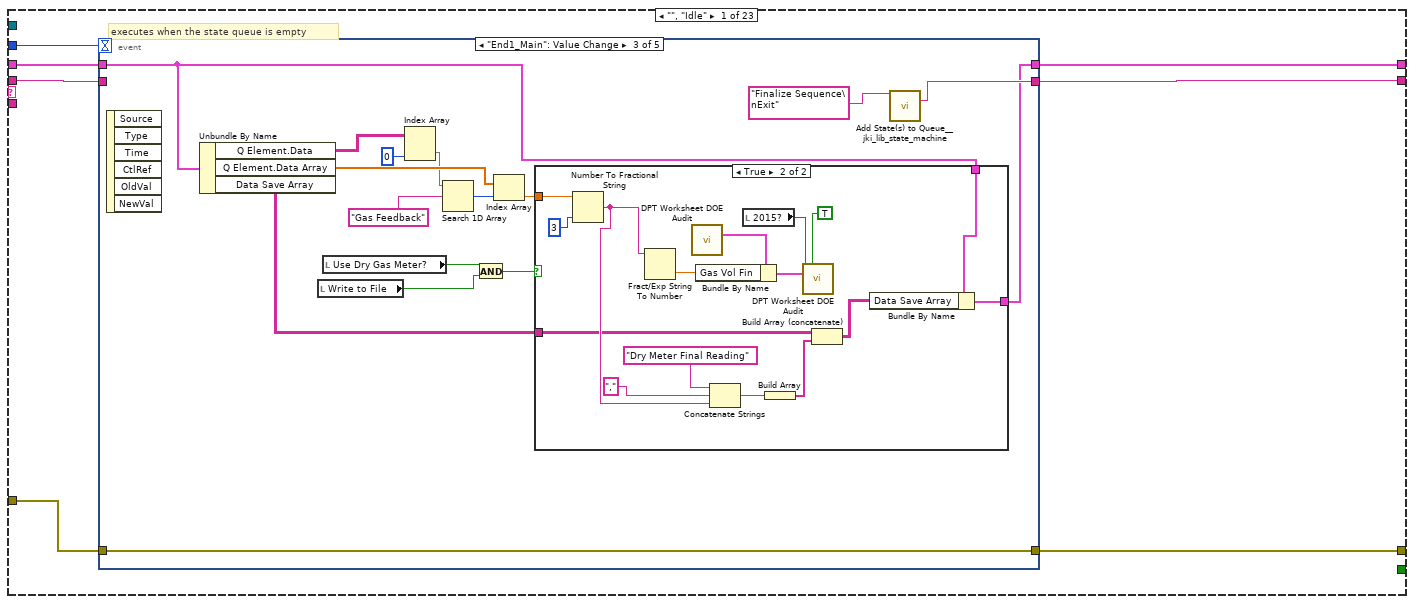
[diagram p10: hidden frame]
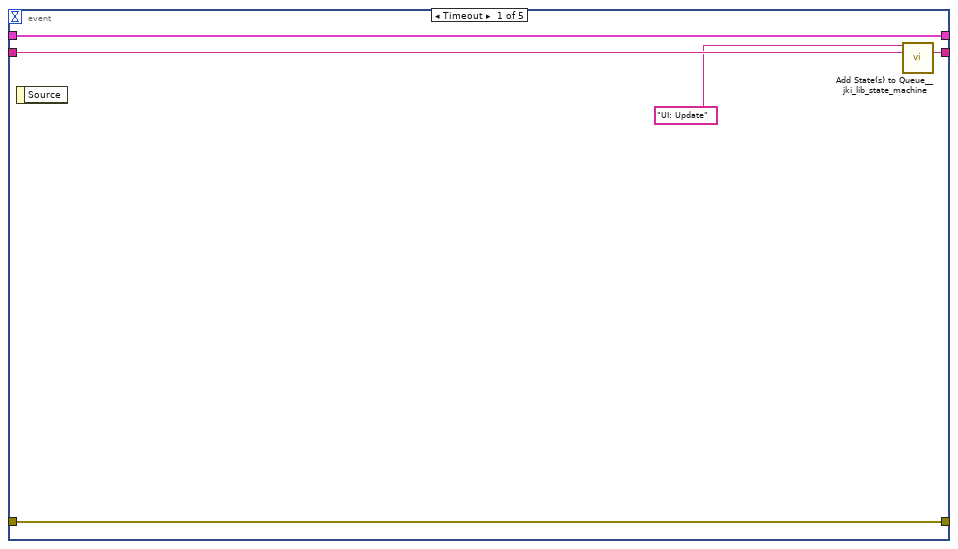
[diagram p11: hidden frame]
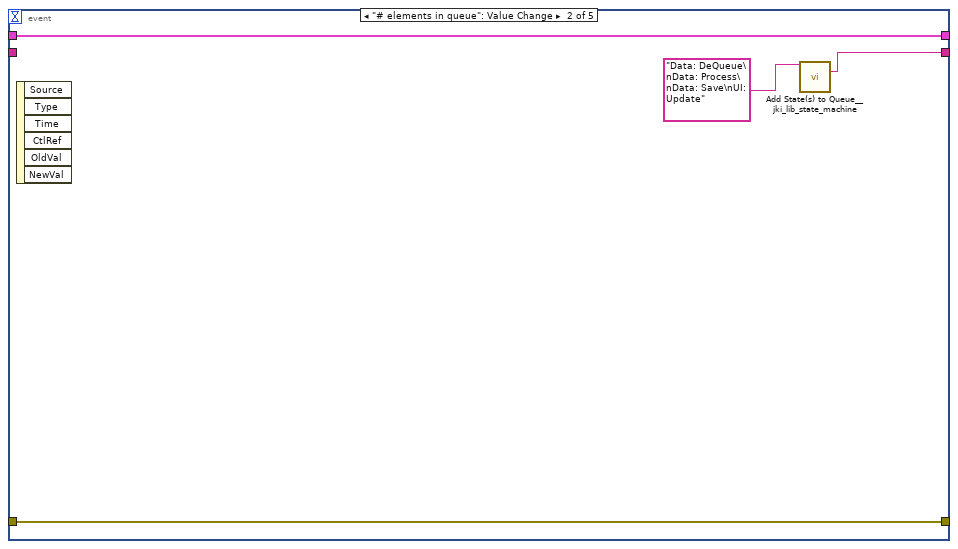
[diagram p12: hidden frame]
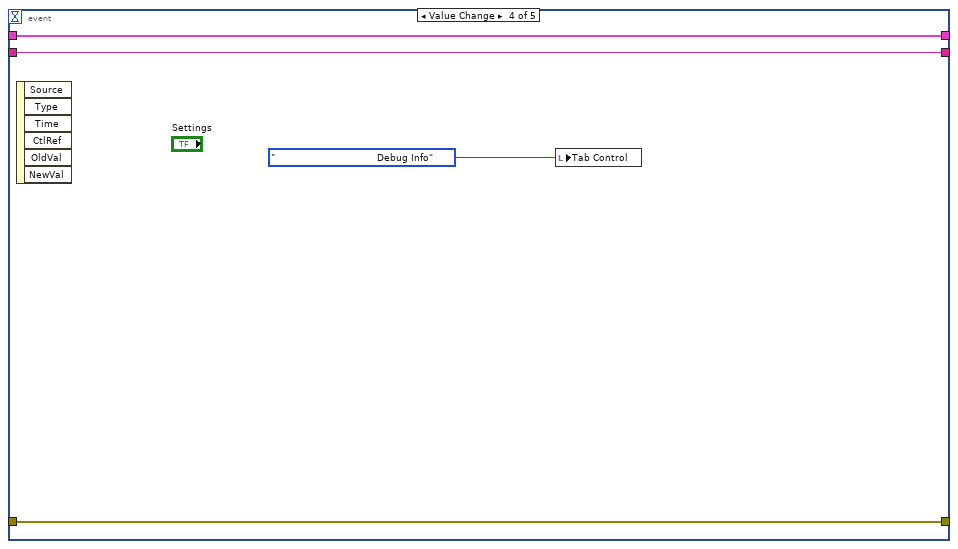
[diagram p14: hidden frame]
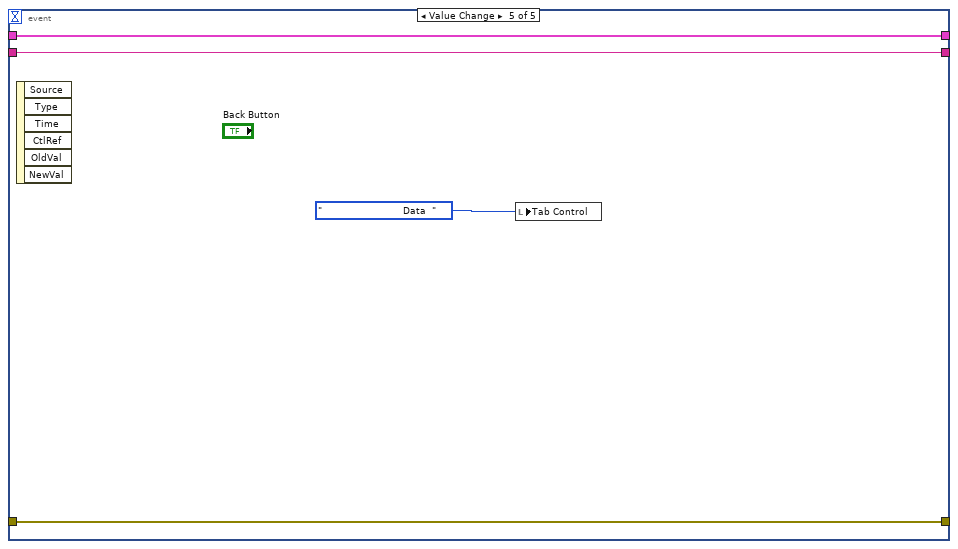
[diagram p15: hidden frame]
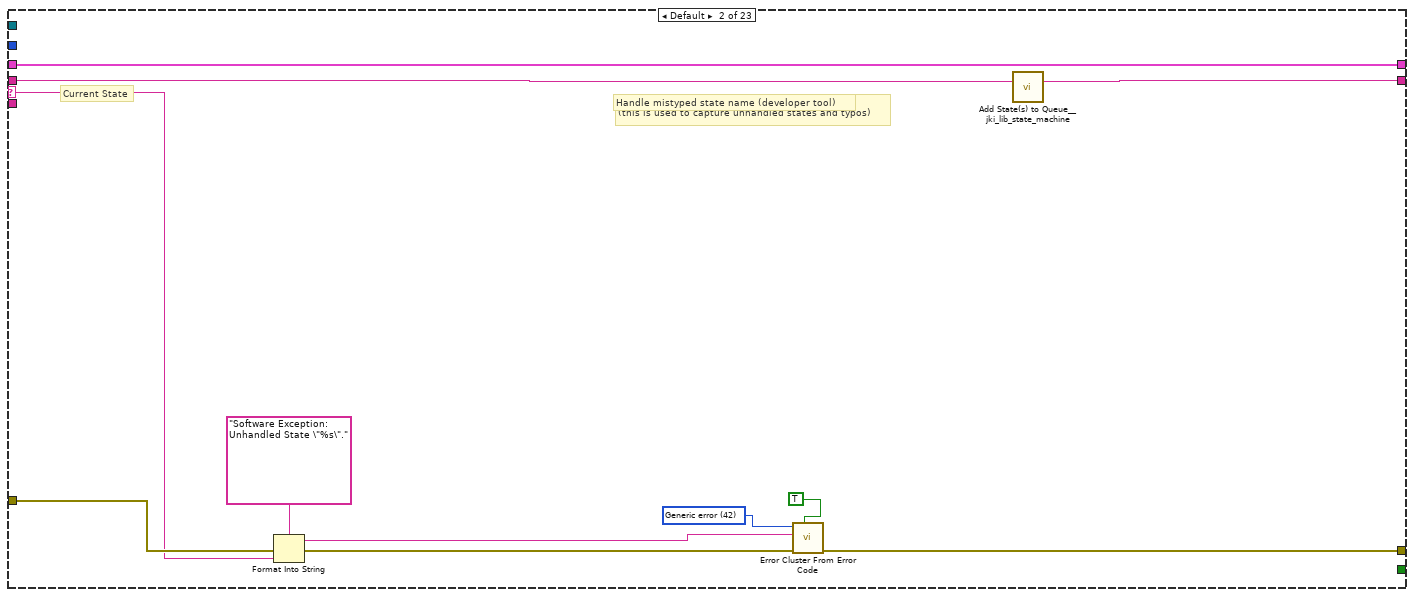
[diagram p16: hidden frame]
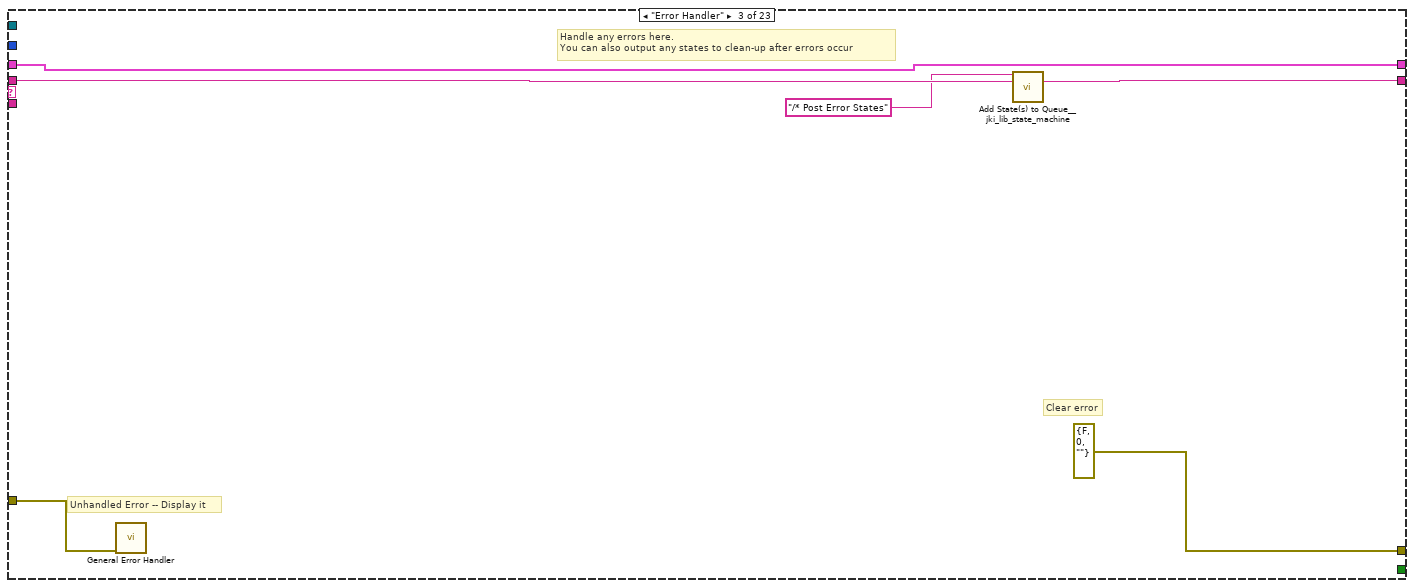
[diagram p17: hidden frame]
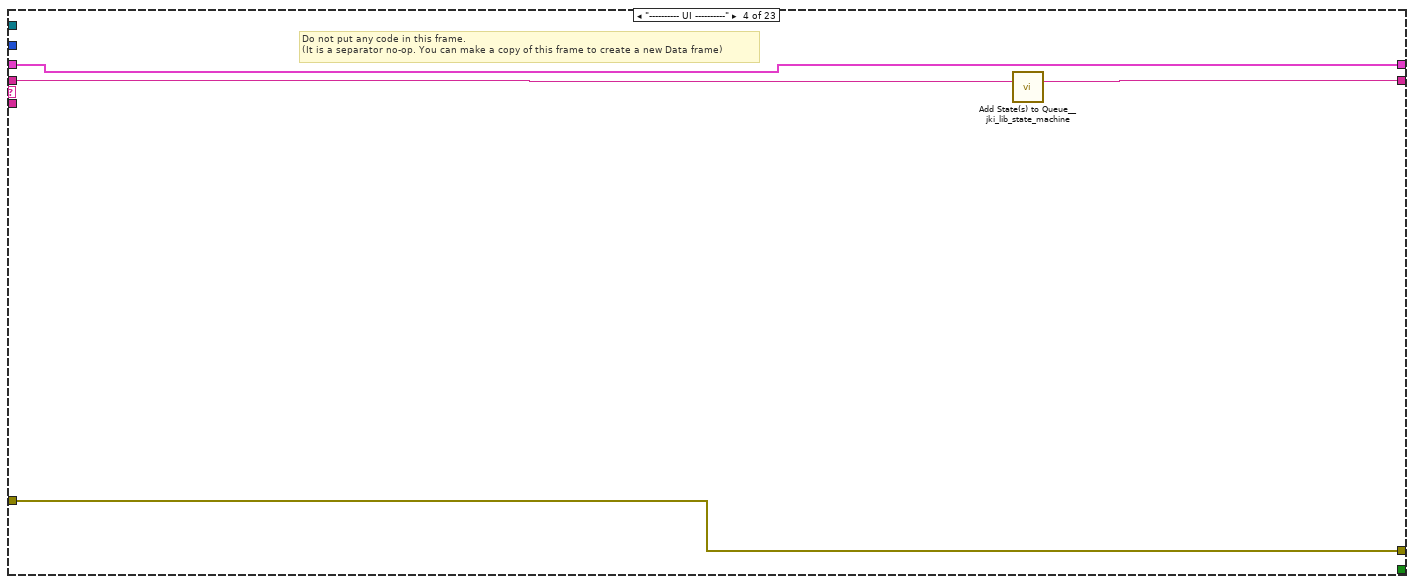
[diagram p18: hidden frame]
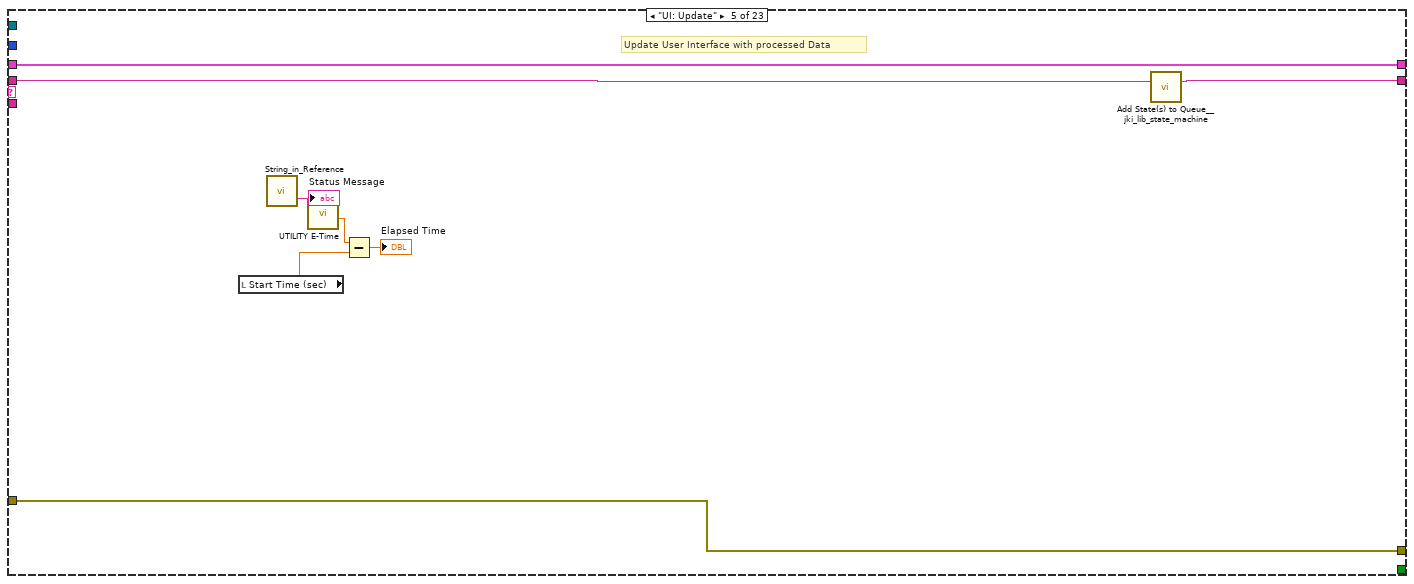
[diagram p19: hidden frame]
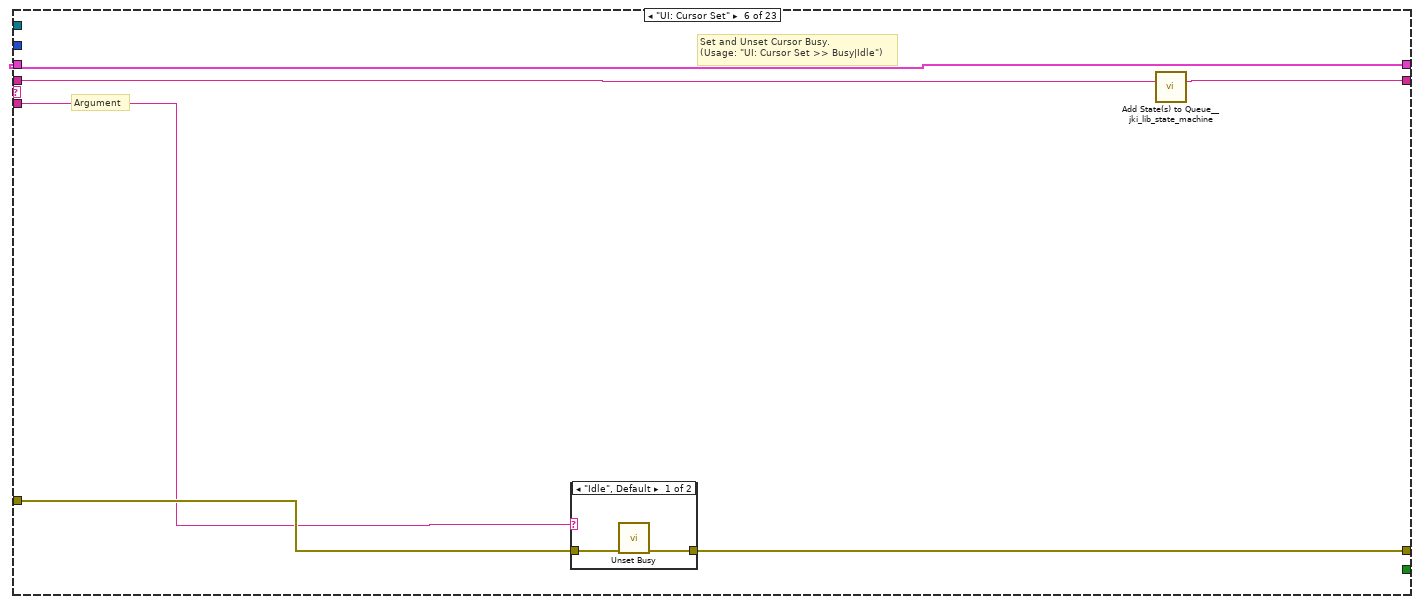
[diagram p20: hidden frame]
diagram:
  # "I am thinking about an automatic\nmanual adjust...but manual will work\nfor now. I think the voltage sense wires \nare in the wrong location. The chroma reads the correct \nvoltage..but the WT500 does not."
  # "Channel List 34970\n101 RDB F\n102 Room Ambient(F)\n103 TC 103\n...\n110 TC 110\n111 Weight\n112 Chamber RH\n113 Chamber Temp\n114 Gas Pressure\n115 Gas Temp\n116 Bar Pre\n117 Gas Feedback"
  # "Channel Array Locations\nCDAQ\n\nTest Pannels\n0-17\n18-35\n36-53\n54-71\n\nAnalogs\nDC 72-79\nAC 80-87\n\nMISC\nGas Temp 88\nGas Pressure 89\nScale 90\nRH 91\nGas Volume 92\nTemp 93\nBar Press 94"
  # "Raw = MeanW  - WDryr;\nCorrW=Raw+Wbouy;\nRMC=((CorrW/BDW)-1)*100;"
  n1 = flat-sequence "Init Test Values" {
    tunnel: [errorcluster {"status"=FALSE, "code"=0, "source"=""} ("Error Out")] -> w13
    tunnel: [w43] -> w19
    tunnel: ["cDAQ Setting"] -> w2
    frame #0 {
      w37 = FALSE ("Reset RMC")
      w28 = TRUE
      w41 = T19 {"Data Array"=[], "Data"=[], "Date"=""}  # Q Element Prototype
      w27 = errorcluster[] [] ("Error Log")
      w35 = "Initializing..." ("String")
      w40 = 1000 ("T1 ComTimer")
      w25 = FALSE ("Init Complete")
      # "Prototype Data Cluster for Data to be Logged"
      n2 = Current VI's Path() -> (path=w30:path)
      n3 = control-ref of="This VI"() -> (w38:refnum<vi>)
      n4 = call "UTILITY This VIs Path.vi"("path"=w30) -> ("File Version Info"=→"Ver.":string, "FileVersionInfo Out"=→"FileVersionInfo Out":T15)  [unwired: 8 in, 5 out]
      n5 = call "String_in_Reference.vi"("String"=w35) -> ()  [unwired: 18 in, 1 out]
      n6 = call "UTILITY E-Time.vi"("Reset"=TRUE) -> ("Elapsed Time (sec)"=w36:dbl)  [unwired: 8 in, 2 out]
      n7 = local write "End Msg"(w35) -> ()
      n8 = local write "Status Message"(w35) -> ()
      n9 = local write "UI Timer"(w40) -> ()
      n10 = local write "DAQ Timer"(w40) -> ()
      n11 = local write "Error Log"(w27) -> ()
      n12 = local write "End Test"(w25) -> ()
      n13 = local write "Loggin Data"(w25) -> ()
      n14 = local write "End1_Main"(w25) -> ()
      n15 = local write "Start Test"(w25) -> ()
      n16 = local write "Get Data Interrupt"(w25) -> ()
      n17 = local write "Write to File"(w25) -> ()
      n18 = local write "End2_DAQ"(w25) -> ()
      n19 = local write "Eng3_Log"(w25) -> ()
      n20 = local write "End_End"(w25) -> ()
      n21 = property on="daq debug array" class="Array (strict)"("Visible"=w28) -> ()  [unwired: 2 in, 2 out]
      n22 = local write "Start Time (sec)"(w36) -> ()
      n23 = local write "Tab Control 2"(enum32{"Debug Only", "Running"}."Running" ("Tab Control 2")) -> ()
      n24 = local write "Tend?"(w36) -> ()
      n25 = property on="Debug List Test States" class="Array (strict)"("Visible"=w28) -> ()  [unwired: 2 in, 2 out]
      n26 = property on="Start Test" class="Boolean (strict)"("Visible"=w25) -> ()  [unwired: 2 in, 2 out]
      n27 = property on="Tab Control" class="TabControl (strict)"("Value"=2) -> ()  [unwired: 2 in, 2 out]
      n28 = local write "Error Log 2"(w27) -> ()
      n29 = local write "Power Off One Shot"(w25) -> ()
      n30 = Obtain Queue(name (unnamed)="Test Data Q", element data type=w41) -> (queue out=w43:refnum<queue>)  [unwired: 3 in, 2 out]
      n31 = property class="VI"(reference=w38, "TB.ShowAbortBut"=w28) -> ()  [unwired: 1 in, 2 out]
      n32 = local write "Power On One Shot"(w37) -> ()
      n33 = local write "None"(w37) -> ()
      n34 = local write "All"(w37) -> ()
      n35 = call "DPT Dryer Power Latches.vi"("Init?"=TRUE) -> ()  [unwired: 8 in, 3 out]
      n36 = local write "Bone Dry Weight (lbs)"(8.0 ("BDW - Bone Dry Wt(lbs)")) -> ()
      n37 = property on="Plot All" class="XYGraph (strict)"("LegScrollVis"=TRUE ("Legend:Scrollbar Visible")) -> ()  [unwired: 2 in, 2 out]
      n38 = local write "Relative Moisture Content (%)"(100.0 ("RMC")) -> ()
      "Q Element" <- w41
      "Debug Mode" <- w28
    }
  }
  n39 = flat-sequence {
    tunnel: ["Macro: Initialize\nConfig: Read\nInitialize Channels\nInitialize Equipment\nStart: Dryer Info\nInit: Nufi\nStart: Files\nStart: Gas Reading\nStart: Ambient\nGet Offset Coeff\nConfig: Write\nStart: Time\nInit Complete\nUI: Front Panel State >> Open\nTest: Main"] -> w11
    tunnel: w2 -> [_]
    frame #0 {
    }
  }
  n40 = call <vilib>:"Add State(s) to Queue__jki_lib_state_machine.vi"("State(s) in (\"\")"=w11) -> ("States Out"=w17:string)  [unwired: 14 in]
  n41 = while "Main Test Process Loop" {
    shift-right: [w56] -> _
    shift-left: _ -> [w55]
    shift-right: [w58] -> w8
    shift-left: w13 -> [w53]
    shift-right: [w57] -> _
    shift-left: w17 -> [w59]
    shift-right: [w51] -> _
    shift-left: string[] [] -> [w50]
    tunnel: [w46] -> w5
    stop <- w52 stop-if-true
    w54 = -1  # Timeout
    n42 = call <vilib>:"Parse State Queue__jki_lib_state_machine.vi"("State Queue"=w59, "Error In (no error)"=w53) -> ("Remaining States"=w60:string, "Current State"=w48:string, "Arguments"=w49:string)  [unwired: 11 in]
    n43 = case shown="\"Test: Main\"" w48 {
      selector: w48 -> [_ _ _ w99 _ _ _ _ _ _ _ _ w269 w316 w345 _ _ _ _ w430 w452 w513 w552 w627 _ _ _ _ _ _ _ _ _ _ _ _ _ _ _ _ _ _ w896]
      tunnel: w60 -> [w66 w74 w98 w103 w119 w141 w145 w157 w162 w175 w226 w254 w275 w321 w352 w373 w385 w390 w408 w433 w455 w516 w555 w633 w652 w663 w667 w687 w698 w722 w730 w759 w773 w781 w785 w790 w807 w811 w832 w885 w890 w894 w904]
      tunnel: w49 -> [_ _ _ _ _ _ _ _ _ _ _ _ _ _ _ _ _ _ _ _ _ _ _ _ _ _ _ _ _ _ w724 _ _ _ _ _ _ _ _ _ _ _ _]
      tunnel: w55 -> [w67 w72 w95 w101 w115 w139 w142 w148 w159 w172 w223 w234 w267 w315 w350 w371 w383 w387 w405 w419 w448 w510 w549 w625 w650 w653 w664 _ w696 w719 w726 w756 w762 w779 w782 w787 w804 w808 w828 w883 w888 w891 w902]
      tunnel: [w65 w71 w96 w105 errorcluster {"status"=FALSE, "code"=0, "source"=""} ("error out") w137 w143 w154 w160 w173 w224 w235 w271 w318 w343 w368 w382 w388 w406 w423 w449 w508 w547 w619 w649 w661 w665 w682 w693 w720 w727 w757 w770 w776 w783 w788 w805 w809 w830 w882 w887 w892 w898] -> w58
      tunnel: w53 -> [w65 w70 w96 w104 w112 w137 w143 w154 w160 w173 w224 w249 w272 w319 w347 w368 w382 w388 w406 w414 w451 w512 w551 w622 w649 w661 w665 w682 w694 w720 w728 w757 w771 w777 w783 w788 w805 w809 w830 w882 w887 w892 w899]
      tunnel: [w66 w73 w97 w102 w118 w140 w144 w156 w161 w174 w225 w253 w274 w320 w351 w372 w384 w389 w407 w432 w454 w515 w554 w632 w651 w662 w666 w686 w697 w721 w729 w758 w772 w780 w784 w789 w806 w810 w831 w884 w889 w893 w903] -> w57
      tunnel: [_ _ _ _ _ w136 _ _ _ _ _ _ _ _ _ _ _ _ _ _ _ _ _ _ _ _ _ _ _ _ _ _ _ _ _ _ _ _ _ _ _ _ _] -> w52
      tunnel: [w67 w69 w95 w101 w114 w139 w142 w155 w159 w171 w223 w228 w266 w314 w350 w370 w383 w387 w405 w419 w447 w509 w548 w611 w650 w653 w664 w685 w696 w719 w726 w756 w761 w779 w782 w787 w804 w808 w828 w883 w888 w891 w902] -> w56
      tunnel: w54 -> [_ w68 _ _ _ _ _ _ _ _ _ _ _ _ _ _ _ _ _ _ _ _ _ _ _ _ _ _ _ _ _ _ _ _ _ _ _ _ _ _ _ _ _]
      tunnel: [_ _ _ _ _ w136 _ _ _ _ _ _ _ _ _ _ _ _ _ _ _ _ _ _ _ _ _ _ _ _ _ _ _ _ _ _ _ _ _ _ _ _ _] -> w46
      frame "ABOUT" {
        (unwired) "This Program has 3 state machines.  The top is the main test loop, where the test sequence is executed. The Second is the Data Acquisition state machine.  It puts the data into a Q that has the datat titles, and raw data in it.  The third \nState Machine deques the Q, saving, processing and displaying the Data.\n\nLegacy code for Agilent still remains.  CDAQ is the main daq."
      }
      frame "", "Idle" {
        # "executes when the state queue is empty"
        n44 = event shown="[1] \"End Test\": Value Change" {
          selector: _ -> [_ _ _ _]
          dyn-events: _ -> [_ _ _ _]
          timeout: w68 -> [_ _ _ _]
          tunnel: w74 -> [w78 w83 w88 w94]
          tunnel: [w77 w82 w87 w93] -> w73
          tunnel: w72 -> [w75 w80 w85 w91]
          tunnel: [w76 w81 w86 w92] -> w71
          tunnel: w70 -> [w76 w81 w86 w92]
          tunnel: [w75 w80 w85 w91] -> w69
          event Timeout {
            n45 = event-data() -> ()  [unwired: 1 in, 1 out]
            n46 = call <vilib>:"Add State(s) to Queue__jki_lib_state_machine.vi"("State(s) in (\"\")"=w78) -> ("States Out"=w77:string)  [unwired: 14 in]
          }
          event Value Change {
            # "Exit Button Value Change (pressed) Event\n(this executes Macro: Exit to terminate the VI)"
            n47 = event-data() -> ()  [unwired: 1 in, 8 out]
            n48 = call <vilib>:"Add State(s) to Queue__jki_lib_state_machine.vi"("State(s) in Front (\"\")"="Power Off\nMacro: Exit", "State(s) in (\"\")"=w83) -> ("States Out"=w82:string)  [unwired: 13 in]
          }
          event "Start Test": Value Change {
            # "This will stop logging until the test is running."
            n49 = event-data() -> ()  [unwired: 1 in, 6 out]
            n50 = call <vilib>:"Add State(s) to Queue__jki_lib_state_machine.vi"("State(s) in Front (\"\")"="Start: Dryer Info\nStart: Gas Reading\nStart: Files\nConfig: Write\nStart: Time\nTest: Main", "State(s) in (\"\")"=w88) -> ("States Out"=w87:string)  [unwired: 13 in]
          }
          event Panel Close? {
            # "Discard the event because we'll close the front panel ourselves in Macro: Exit"
            # "Close Panel button (pressed) Event\n(this executes Macro: Exit to terminate the VI)"
            n51 = event-data() -> ()  [unwired: 1 in, 1 out]
            n52 = call <vilib>:"Add State(s) to Queue__jki_lib_state_machine.vi"("State(s) in Front (\"\")"="Macro: Exit", "State(s) in (\"\")"=w94) -> ("States Out"=w93:string)  [unwired: 13 in]
            n53 = event-data("Discard?"=TRUE) -> ()  [unwired: 1 in, 1 out]
          }
        }
      }
      frame "---------- Core ----------" {
        # "Do not put any code in this frame.\n(it is a separator no-op)"
        n54 = call <vilib>:"Add State(s) to Queue__jki_lib_state_machine.vi"("State(s) in (\"\")"=w98) -> ("States Out"=w97:string)  [unwired: 14 in]
      }
      frame Default {
        w108 = 42 items=["No error", "Argument error", "Memory is full", "Out of zone", "End of file", "File already open", "Generic file I/O error", "File not found", "File permission error", "Disk is full", "Duplicate path", "Too many files open", "System feature not enabled", "Resource file not found", "Cannot add resource", "Resource not found", "Image not found", "Image memory error", "Pen does not exist", "Config type invalid", "Config token not found", "Config parse error", "Config memory error", "Bad external code format", "Bad external code offset", "External code not present", "Null window", "Destroy window error", "Null menu", "Print aborted", "Bad print record", "Print driver error", "Windows error during printing", "Memory error during printing", "Print dialog error", "Generic print error", "Invalid device refnum", "Device not found", "Device parameter error", "Device unit error", "Cannot open device", "Device call aborted", "Generic error", "Cancelled by user", "Object ID too low", "Object ID too high", "Object not in heap", "Unknown heap", "Unknown object (invalid DefProc)", "Unknown object (DefProc not in table)", "Message out of range", "Invalid (null) method", "Unknown message", "Manager call not supported", "Bad address", "Network operation in progress", "Network operation timed out", "Connection is busy", "Network attribute not supported", "Network error", "Address in use", "System out of memory", "Connection aborted", "Connection refused", "Not connected", "Already connected", "Connection closed", "Initialization error (interapplication manager)", "Bad occurrence", "Wait on unbound occurrence handler", "Occurrence queue overflow", "Datalog type conflict", "Unused", "Unrecognized type (interapplication manager)", "Memory corrupt", "Failed to make temporary DLL", "Old CIN version", "Drag socket not found", "Failed to load drop-object", "Failed to register OLE object", "Failed to release OLE object", "Format specifier type mismatch", "Unknown format specifier", "Too few format specifiers", "Too many format specifiers", "Scan failed", "Newer CIN version", "Error converting to variant", "Runtime menu error", "Password tampered", "Variant attribute not found", "Incompatible variant data type", "Event data is not available", "Event Store is not present", "Occurrence is not found", "Event Queue is not created", "Event info is not available", "Refnum passed is NULL", "Error retrieving Class GUID", "Error retrieving CoClass GUID", "Error retrieving TypeLib GUID.", "Bad built application magic bytes.", "Specific driver is different from the specific driver associated with the Logical Name.", "There is no session opened to the class driver.", "Max Error", "MAX - Error with config objects", "MAX - Error loading configuration", "MAX - Group not supported"]
        # "Current State"
        # "Do not delete, rename, or modify this frame.\n(this is used to capture unhandled states and typos)"
        # "Handle mistyped state name (developer tool)"
        n55 = Format Into String(format string="Software Exception: Unhandled State \"%s\"." ("message"), error in=w104, w99) -> (resulting string=w107:string, error out=w106:errorcluster)  [unwired: 1 in]
        n56 = call <vilib>:"Error Cluster From Error Code.vi"("show call chain? (False)"=TRUE, "error in (no error)"=w106, "error message (\"\")"=w107, "error code (0)"=w108) -> ("error out"=w105:errorcluster)  [unwired: 5 in]
        n57 = call <vilib>:"Add State(s) to Queue__jki_lib_state_machine.vi"("State(s) in (\"\")"=w103) -> ("States Out"=w102:string)  [unwired: 14 in]
      }
      frame "Error Handler" {
        # "Unhandled Error -- Display it"
        # "Handle any errors here.\nYou can also output any states to clean-up after errors occur"
        # "Clear error"
        n58 = Unbundle By Name(w115) -> ("Error Log"=w116:errorcluster[])
        n59 = local read "Loggin Data"() -> (w111:bool)
        n60 = Build Array (concatenate)(w116, w112) -> (w113:errorcluster[])
        n61 = case shown="True" w111 {
          tunnel: w113 -> [w120 w133]
          tunnel: w112 -> [_ w132]
          tunnel: ["Macro: Exit" "Macro: Exit"] -> w110
          frame False {
            n62 = local write "Error Log"(w120) -> ()
          }
          frame True {
            n63 = call "UTILITY Counter.vi"() -> ("Count"=w130:dbl)  [unwired: 11 in]
            "Error Count" <- w130
            n64 = Unbundle By Name(w132) -> ("code"=w125:i32, "source"=w126:string)  [unwired: 1 out]
            n65 = local read "Write to File"() -> (w122:bool)
            n66 = Format Into String(format string="%s %d %s %d %s %s", "Error Count: " ("input 1"), w130, " Code: " ("input 1"), w125, " Source: " ("input 1"), w126) -> (resulting string=w124:string)  [unwired: 2 in, 1 out]
            n67 = case shown="True" w122 {
              tunnel: w124 -> [_ w135]
              frame False {
              }
              frame True {
                n68 = local read "FileName DataLog"() -> (w134:path)
                n69 = call "UTILITY Log String to Spreadsheet.vi"("String"=w135, "FileName"=w134) -> ()  [unwired: 9 in, 1 out]
              }
            }
            "Error Log" <- w133
          }
        }
        n70 = Bundle By Name(cluster=w115, "Error Log"=w113) -> (w114:T24)
        n71 = call <vilib>:"Add State(s) to Queue__jki_lib_state_machine.vi"("State(s) in Front (\"\")"=w110, "State(s) in (\"\")"=w119) -> ("States Out"=w118:string)  [unwired: 13 in]
      }
      frame "Exit" {
        w136 = TRUE
        # "Do not put any code in this frame.\n(No errors that occur here will be handled.)"
        n72 = call "String_in_Reference.vi"("String"="Stopping Test..." ("string")) -> ()  [unwired: 18 in, 1 out]
        n73 = call <vilib>:"Add State(s) to Queue__jki_lib_state_machine.vi"("State(s) in (\"\")"=w141) -> ("States Out"=w140:string)  [unwired: 14 in]
      }
      frame "-------Initialize-------" {
        # "Do not put any code in this frame.\n(It is a separator no-op. You can make a copy of this frame to create a new Data frame)"
        n74 = call <vilib>:"Add State(s) to Queue__jki_lib_state_machine.vi"("State(s) in (\"\")"=w145) -> ("States Out"=w144:string)  [unwired: 14 in]
      }
      frame "Initialize Core Data" {
        # "Do not delete, rename, or modify this frame.\n(this is used to determine panel behavior on exit)"
        # "originally closed?"
        # "exe?"
        # "If panel starts closed or is an EXE, then close it when we exit"
        n75 = property class="VI"() -> ("Front Panel.Open"=w153:bool)  [unwired: 2 in, 2 out]
        n76 = control-ref of="Current VI Reference"() -> (w146:refnum<vi>)
        n77 = property class="App"() -> ("App.Kind"=w152:T20)  [unwired: 2 in, 2 out]
        n78 = Not(x=w153) -> (.not. x?=w150:bool)
        n79 = Equal?(x=w152, y=T20."Run Time System" ("Application:Kind")) -> (x = y?=w149:bool)
        "exe?" <- w149
        n80 = Or(x=w150, y=w149) -> (x .or. y?=w147:bool)
        n81 = Bundle By Name(cluster=w148, "Core.Current VI Reference"=w146, "Core.Close Panel on Exit?"=w147) -> (w155:T24)
        n82 = call <vilib>:"Add State(s) to Queue__jki_lib_state_machine.vi"("State(s) in (\"\")"=w157) -> ("States Out"=w156:string)  [unwired: 14 in]
      }
      frame "Initialize Channels" {
        n83 = call <vilib>:"Add State(s) to Queue__jki_lib_state_machine.vi"("State(s) in Front (\"\")"="Initialize CDAQ Channels" ("State(s) in Front (\"\")"), "State(s) in (\"\")"=w162) -> ("States Out"=w161:string)  [unwired: 13 in]
      }
      frame "Initialize CDAQ Channels" {
        # "This shouldn't be needed"
        # "Label names for data"
        n84 = call "DPT TC Panel Setup.vi"() -> ("Channel List"=w167:string, "Label Array"=w163:string[], "Indexes used"=→"Indexes used":i32[])  [unwired: 13 in]
        "TC Channel List" <- w167
        "DAQ Label List" <- w163
        n85 = disable-structure shown="Disabled" {
          disable-tunnel: w167 -> [w202 _]
          disable-tunnel: [w201 _] -> w166
          disable-tunnel: w163 -> [w200 _]
          frame Disabled {
            w176 = "," ("string")
            # "if ends in , remove it"
            n86 = global read "DPT Global Test Variables.vi" "Globals for Dryer Performance Test"() -> (w185:T17)
            n87 = Unbundle By Name(w185) -> ("cDAQ Array Locations.Scale Channel"=w184:string, "cDAQ Array Locations.RH Chan"=w183:string, "cDAQ Array Locations.Temp Chan"=w182:string, "Test Setup.Gas Enabled"=w177:bool, "cDAQ Array Locations.Gas Pressure"=w181:string, "cDAQ Array Locations.Gas Temperature"=w180:string, "cDAQ Array Locations.Barometric Pressure"=w179:string, "cDAQ Array Locations.Gas Feedback Chan"=w178:string)
            n88 = call "DPT Panel Voltage Panel Setup.vi"("Channel List In"=w202, "Label List In"=w200) -> ("Channel List Out"=w208:string, "Label List Out"=w207:string[], "Stream DC to File(out)?"=→"Stream DC to File?":bool)  [unwired: 11 in]
            n89 = Concatenate Strings(w184, w176, w183, w176, w182) -> (w206:string)
            n90 = String Length(string=w208) -> (length=w199:i32)
            n91 = Greater Than 0?(x=w199) -> (x > 0?=w196:bool)
            n92 = Select(t=",", s=w196, f="") -> (s? t:f=w195:string)
            n93 = case shown="True" w177 {
              tunnel: ["" w217] -> w205
              tunnel: [string[] [] ("Label List 2") string[] ["Gas Pressure", "Gas Temperature", "Barometric Pressure", "Gas Feedback"] ("Label List 2")] -> w186
              tunnel: w181 -> [_ w214]
              tunnel: w180 -> [_ w213]
              tunnel: w179 -> [_ w212]
              tunnel: w178 -> [_ w211]
              frame False {
              }
              frame True {
                w215 = "," ("string")
                n94 = Concatenate Strings(w215, w214, w215, w213, w215, w212, w215, w211) -> (w217:string)
              }
            }
            n95 = Concatenate Strings(w208, w195, w206, w205) -> (w189:string)
            n96 = String Length(string=w189) -> (length=w194:i32)
            n97 = Decrement(x=w194) -> (x-1=w188:i32)
            n98 = String Subset(string=w189, offset (0)=w188, length (rest)=1 ("length (rest)")) -> (substring=w192:string)
            n99 = Build Array (concatenate)(w207, w186) -> (w204:string[])  [unwired: 1 in]
            n100 = Equal?(x=w192, y=",") -> (x = y?=w190:bool)
            n101 = case shown="True" w190 {
              tunnel: w189 -> [w218 w222]
              tunnel: w188 -> [_ w220]
              tunnel: [w218 w219] -> w187
              frame False {
              }
              frame True {
                n102 = String Subset(string=w222, offset (0)=0, length (rest)=w220) -> (substring=w219:string)
              }
            }
            n103 = call "Agilent Sort Channels.vi"("Agilent Chanel List"=w187, "Agilent Label List"=w204) -> ("Sorted Channels"=w201:string)  [unwired: 12 in, 1 out]
          }
          frame Enabled {
          }
        }
        "DAQ Channel List" <- w166
        n104 = Search and Replace String(replace all?=TRUE ("replace all? (F)"), input string=w167, search string=",") -> (number of replacements=w168:i32)  [unwired: 5 in, 3 out]
        n105 = Increment(x=w168) -> (x+1=→"Number of TCs":i32)
        n106 = Bundle By Name(cluster=w172, "DAQ Chan List"=w166, "DAQ Label List"=w163) -> (w171:T24)
        n107 = call <vilib>:"Add State(s) to Queue__jki_lib_state_machine.vi"("State(s) in (\"\")"=w175) -> ("States Out"=w174:string)  [unwired: 14 in]
      }
      frame "----Initialize Equip-----" {
        # "Do not put any code in this frame.\n(It is a separator no-op. You can make a copy of this frame to create a new Data frame)"
        n108 = call <vilib>:"Add State(s) to Queue__jki_lib_state_machine.vi"("State(s) in (\"\")"=w226) -> ("States Out"=w225:string)  [unwired: 14 in]
      }
      frame "Initialize Equipment" {
        w240 = 4  # Invalid IP Address Length Size
        # "Panel to enter drum volume, MA filter, and scale temp coeff.  \nDrum volume needs to be experimentally determined, depending on a heated run with no clothes.\nThis data is processed with anther program.\n(FIXME, maybe automatically generate this?)"
        n109 = global read "DPT Global Test Variables.vi" "Globals for Dryer Performance Test"() -> (w244:T17)
        n110 = Unbundle By Name(w234) -> ("Equipment"=w251:T8)
        n111 = Unbundle By Name(w244) -> ("Test Setup.CompVolume"=w238:dbl, "Test Setup.MA Filter Size"=w243:i32, "Test Setup.RH-IP"=w242:string)
        n112 = Bundle By Name(cluster=w251, "Com Flow Computer"=refnum<visa-resource-name> "COM1") -> (w229:T8)
        n113 = local read "Use Smoothing"() -> (w245:bool)
        n114 = String Length(string=w242) -> (length=w241:i32)
        n115 = local write "MA Filter Size"(w243) -> ()
        n116 = Greater?(x=w241, y=w240) -> (0:→"ITHX RH Sensor":bool)
        n117 = call "DPT Panel Volume Size.vi"("Default Volume Value"=w238, "Error In"=w249) -> ("Scale Temp Coeff Out"=w248:dbl, "Drum Volume"=w237:dbl, "Out Strings"=w246:string[][], "Error Out"=w236:errorcluster)  [unwired: 9 in, 1 out]
        n118 = case shown="True" w245 {
          tunnel: [w255 w259] -> w247
          tunnel: w246 -> [w255 w258]
          frame False {
          }
          frame True {
            n119 = Insert Into Array(array=w258, index (row)=0, new element=string[] ["Smoothing Used"] ("new element/subarray")) -> (w259:string[][])  [unwired: 1 in]
          }
        }
        n120 = local write "Scale Temp Coeff"(w248) -> ()
        n121 = local write "Drum Volume"(w237) -> ()
        n122 = Unbundle By Name(w234) -> ("Power Analyzer"=w232:T9, "Standby Power Settings"=w233:path)
        n123 = call "Power Settings.vi"("error in (no error)"=w236, "File Path Control"=w233, "Power Analyzer"=w232) -> ("error out"=w235:errorcluster, "Power Analyzer Out"=w230:T9, "Power Out"=w231:T7)  [unwired: 6 in]
        "Power Out" <- w231
        n124 = Bundle By Name(cluster=w234, "Equipment"=w229, "Start Header Data"=w247, "Equipment.Power"=w231, "Power Analyzer"=w230) -> (w228:T24)
        n125 = Unbundle By Name(w228) -> ("Equipment"=→"Equipment":T8)
        n126 = case shown="No Error" w235 {
          selector: w235 -> [_ w261]
          tunnel: ["Init: Power\nInit: Gas\nOff Mode Power" ("State(s) in Front (\"\")") "Macro: Exit" ("State(s) in Front (\"\")")] -> w252
          frame No Error {
          }
          frame Error {
            n127 = call <vilib>:"Simple Error Handler.vi"("error in (no error)"=w261) -> ()  [unwired: 4 in, 5 out]
          }
        }
        n128 = call <vilib>:"Add State(s) to Queue__jki_lib_state_machine.vi"("State(s) in Front (\"\")"=w252, "State(s) in (\"\")"=w254) -> ("States Out"=w253:string)  [unwired: 13 in]
      }
      frame "Init: Power" {
        # "Power up the Chroma"
        n129 = Unbundle By Name(w267) -> ("Equipment.Power.Power Supply.Chroma 61605"=w273:refnum<visa-resource-name>, "Equipment.Power.Power Supply.Use Chroma?"=w264:bool)
        n130 = global read "DPT Global Test Variables.vi" "Globals for Dryer Performance Test"() -> (w268:T17)
        n131 = case shown="False" "Simulate" {
          tunnel: w273 -> [w290 _]
          tunnel: [w281 w303] -> w271
          tunnel: w272 -> [w289 w303]
          tunnel: w268 -> [w288 _]
          tunnel: [w282 "Electric" ("Chroma Power Setting Out")] -> w263
          tunnel: w264 -> [w283 _]
          frame False {
            n132 = call "DPT Panel Power Setting.vi"() -> ("Dryer Type Out"=w286:string, "Chroma Power Setting Out"=w282:string)  [unwired: 14 in]
            n133 = Bundle By Name(cluster=w288, "Test Information.Dryer Type"=w286) -> (w287:T17)
            n134 = case shown="\"120\", Default" w282 {
              tunnel: [w297 w299 w301] -> w285
              tunnel: [w296 w298 w300] -> w284
              tunnel: w283 -> [w296 w298 w300]
              frame "120", Default {
                w297 = T22[] [enum."Initialize", enum."Output On 120"] items=["Initialize", "Output On 120", "Output On 240", "Output On 208", "Output Off", "Status", "Send Command", "Track Current"]
              }
              frame "208" {
                w299 = T22[] [enum."Initialize", enum."Output On 208"] items=["Initialize", "Output On 120", "Output On 240", "Output On 208", "Output Off", "Status", "Send Command", "Track Current"]
              }
              frame "240" {
                w301 = T22[] [enum."Initialize", enum."Output On 240"] items=["Initialize", "Output On 120", "Output On 240", "Output On 208", "Output Off", "Status", "Send Command", "Track Current"]
              }
            }
            "Use Chroma" <- w284
            n135 = global write "DPT Global Test Variables.vi" "Globals for Dryer Performance Test"(w287) -> ()
            n136 = for {
              tunnel: w290 -> [w295]
              tunnel: w285 -> [w292] mode=indexing
              shift-right: [w293] -> w281
              shift-left: w289 -> [w294]
              n137 = call "Chroma 617xx Driver GPIB-VISA-RW.vi"("VISA resource name"=w295, "Chroma Power Select"=w292, "Use Adjusted Voltage"=FALSE, "error in (no error)"=w294) -> ("error out"=w293:errorcluster)  [unwired: 10 in, 1 out]
            }
          }
          frame True {
          }
        }
        n138 = local write "Supply Voltage:"(w263) -> ()
        n139 = Bundle By Name(cluster=w267, "Dryer Type"=w263) -> (w266:T24)
        n140 = case shown="No Error" w271 {
          tunnel: ["" ("State(s) in Front (\"\")") "Macro: Exit" ("State(s) in Front (\"\")")] -> w270
          tunnel: w269 -> [_ w278]
          frame No Error {
          }
          frame Error {
            n141 = Concatenate Strings("Error:", w278) -> (w280:string)
            n142 = One Button Dialog(message=w280) -> ()  [unwired: 1 in, 1 out]
          }
        }
        n143 = call <vilib>:"Add State(s) to Queue__jki_lib_state_machine.vi"("State(s) in Front (\"\")"=w270, "State(s) in (\"\")"=w275) -> ("States Out"=w274:string)  [unwired: 13 in]
      }
      frame "Init: Gas" {
        # "Initializes the gas data for the header.  Also, triggers the bool indicating\nwhether gas is going to be used."
        # "(OPEC) and a majority of the natural gas industry in North America have adopted 60 °F and 14.73 psia \nas their standard reference conditions (instead of 60 °F and 14.696 psia) for expressing natural gas volumes and flow rates"
        n144 = global read "DPT Global Test Variables.vi" "Globals for Dryer Performance Test"() -> (w312:T17)
        n145 = Unbundle By Name(w315) -> ("Start Header Data"=w306:string[][])
        n146 = Unbundle By Name(w312) -> ("Test Information.Dryer Type"=w311:string)
        n147 = local read "Simulate"() -> (w307:bool)
        n148 = Equal?(x="Gas", y=w311) -> (x = y?=w304:bool)
        n149 = Compound Arithmetic op=AND(invert w307, w304) -> (w305:bool)
        n150 = case shown="True" w305 {
          tunnel: [w329 w332] -> w318
          tunnel: w319 -> [w329 w333]
          tunnel: [w328 w338] -> w313
          tunnel: [w327 FALSE ("Use Dry Gas Meter Out?")] -> w309
          tunnel: [w327 TRUE ("Use Dry Gas Meter Out?")] -> w308
          tunnel: w306 -> [w328 w339]
          frame False {
            w327 = FALSE ("Use Dry Gas Meter Out?")
          }
          frame True {
            n151 = call "DPT Panel Init Dry Flow Meter.vi"("Error In"=w333) -> ("Heat Val."=w330:dbl, "BTUF3"=w331:string[][], "Error Out"=w332:errorcluster)  [unwired: 12 in]
            n152 = call "DPT Worksheet DOE Audit.vi"() -> ("DOE Data Out"=w337:T25)  [unwired: 13 in, 2 out]
            n153 = Bundle By Name(cluster=w337, "Gas Heat Val"=w330) -> (w336:T25)
            n154 = local read "2015?"() -> (w334:bool)
            n155 = call "DPT Worksheet DOE Audit.vi"("2015?"=w334, "Add?"=TRUE, "DOE Data"=w336) -> ()  [unwired: 10 in, 3 out]
            n156 = Build Array (concatenate)(w339, w331) -> (w338:string[][])
            "BTUF3" <- w338
          }
        }
        "Use Dry Gas Meter?" <- w308
        "Use SL9200 Gas Readings?" <- w309
        n157 = Bundle By Name(cluster=w315, "Start Header Data"=w313) -> (w314:T24)
        n158 = case shown="No Error" w318 {
          tunnel: ["" ("State(s) in Front (\"\")") "Macro: Exit" ("State(s) in Front (\"\")")] -> w317
          tunnel: w316 -> [_ w324]
          frame No Error {
          }
          frame Error {
            n159 = Concatenate Strings("Error:", w324) -> (w326:string)
            n160 = One Button Dialog(message=w326) -> ()  [unwired: 1 in, 1 out]
          }
        }
        n161 = call <vilib>:"Add State(s) to Queue__jki_lib_state_machine.vi"("State(s) in Front (\"\")"=w317, "State(s) in (\"\")"=w321) -> ("States Out"=w320:string)  [unwired: 13 in]
      }
      frame "Init: Power Analyzer" {
        # "This delay allows the \npower analyzer to stablize. \nWhen it first starts it can throw\nhigh watts, which throws off\nthe dryer precondition"
        # "Initialize WT500."
        n162 = Unbundle By Name(w350) -> ("Equipment.Power.Yokogawa.WT500.Power VISA Yokogawa WT500"=w349:refnum<visa-resource-name>)
        n163 = local read "Simulate"() -> (w348:bool)
        n164 = case shown="False" w348 {
          tunnel: w349 -> [w359 _]
          tunnel: [w366 w367] -> w344
          tunnel: w347 -> [w364 w367]
          frame False {
            w362 = u16 0 items=["AUTO", "500 mA", "1 A", "2 A", "5 A", "10 A", "20 A", "40 A", "S-AUTO", "50 mV", "100 mV", "200 mV", "500 mV", "1 V", "2 V", "5 V", "10 V", "250 mA", "500 mA", "1 A", "2.5 A", "5 A", "10 A", "20 A", "25 mV", "50 mV", "100 mV", "250 mV", "500 mV", "1 V", "2.5 V", "5 V"] ("I Range (7: 40A)")
            w363 = u16 0 items=["AUTO", "15", "30", "60", "100", "150", "300", "600", "1000", "7.5", "15", "30", "50", "75", "150", "300", "500"] ("V Range (8: 1000V)")
            n165 = call "WT500 Initialize.vi"("VISA resource name"=w359, "V Range (8: 1000V)"=w363, "I Range (7: 40A)"=w362, "Error In (No Error) 2"=w364) -> ("Label"=→"Power Label":string[], "VISA resource name out"=w361:refnum<visa-resource-name>, "Error Out"=w360:errorcluster)  [unwired: 4 in]
            n166 = call "YKWT500 Error Query.vi"("error in (no error)"=w360, "VISA resource name"=w361) -> ("error out"=w366:errorcluster, "Error Message"=w358:string)  [unwired: 6 in, 2 out]
            n167 = local write "Status Message"(w358) -> ()
          }
          frame True {
          }
        }
        n168 = call "UTILITY Delay mS.vi"("Error In"=w344, "milliseconds to wait"=u32 1000) -> ("Error Out"=w343:errorcluster)  [unwired: 13 in]
        n169 = case shown="No Error" w343 {
          tunnel: ["Init: CDAQ" ("State(s) in Front (\"\")") "Macro: Exit" ("State(s) in Front (\"\")")] -> w346
          tunnel: w345 -> [_ w355]
          frame No Error {
          }
          frame Error {
            n170 = Concatenate Strings("Error:", w355) -> (w357:string)
            n171 = One Button Dialog(message=w357) -> ()  [unwired: 1 in, 1 out]
          }
        }
        n172 = call <vilib>:"Add State(s) to Queue__jki_lib_state_machine.vi"("State(s) in Front (\"\")"=w346, "State(s) in (\"\")"=w352) -> ("States Out"=w351:string)  [unwired: 13 in]
      }
      frame "Init: CDAQ" {
        # "5/29 replaced ChanTester: Init cDAQ, Gather Data- M.S."
        n173 = Unbundle By Name(w371) -> ("CDAQ Tasks"=w369:refnum<k21>[])
        n174 = disable-structure shown="Disabled" {
          disable-tunnel: [w380 _] -> _
          disable-tunnel: _ -> [w377 _]
          disable-tunnel: [w376 _] -> _
          disable-tunnel: _ -> [w374 _]
          frame Disabled {
            n175 = call "cDAQ Channel Tester.vi"(7:w377, "error in (no error)"=w374, 11:T21."Init CDAQ" ("Mode")) -> ("error out"=w375:errorcluster, 5:w378)  [unwired: 7 in]
            n176 = call "cDAQ Channel Tester.vi"(7:w378, "error in (no error)"=w375, 11:T21."Gather DATA" ("Mode")) -> ("error out"=w380:errorcluster, 5:w376)  [unwired: 7 in]
          }
          frame Enabled {
          }
        }
        n177 = call <vilib>:"Add State(s) to Queue__jki_lib_state_machine.vi"("State(s) in (\"\")"=w373) -> ("States Out"=w372:string)  [unwired: 14 in]
        n178 = Bundle By Name(cluster=w371, "CDAQ Tasks"=w369) -> (w370:T24)
      }
      frame "Init: Nufi" {
        # "Need to install new newfi tool"
        n179 = call <vilib>:"Add State(s) to Queue__jki_lib_state_machine.vi"("State(s) in (\"\")"=w385) -> ("States Out"=w384:string)  [unwired: 14 in]
      }
      frame "Init Complete" {
        n180 = Unbundle By Name(w387) -> ("Equipment.Power.Yokogawa.WT500.Power VISA Yokogawa WT500"=w386:refnum<visa-resource-name>)
        n181 = flat-sequence {
          tunnel: w386 -> [w392]
          frame #0 {
            # "\"Whenever there is a wait period you have to clear the CDAQ buffer..or you will get error. Need to fix!!\"   <-- This should be fixed with these new VI's (M.S.)"
            # "This corrects the time issue due to the amount of \ntime it takes to load the dryer and turn on. Without\nthis routine, we generally report approx. 1 minute longer\ndrying time."
            n182 = while {
              tunnel: w392 -> [w394]
              stop <- w399 stop-if-true
              n183 = call "WT500 Get Power Data.vi"("VISA resource name"=w394) -> ("error out"=w397:errorcluster, "Power Data Out"=w395:T26, "VISA resource name out"=w396:refnum<visa-resource-name>)  [unwired: 4 in, 3 out]
              n184 = Unbundle By Name(w395) -> ("P:Sigma"=w401:dbl)
              n185 = call "YKWT500 Error Query.vi"("error in (no error)"=w397, "VISA resource name"=w396) -> ("Error Message"=w393:string)  [unwired: 6 in, 3 out]
              n186 = local write "Status Message"(w393) -> ()
              n187 = Greater?(x=w401, y=50.0) -> (0:w399:bool)
              n188 = Wait (ms)(milliseconds to wait=u32 500) -> ()  [unwired: 1 out]
            }
            n189 = call "String_in_Reference.vi"("String"="Waiting  for Power ON..." ("string")) -> ()  [unwired: 18 in, 1 out]
          }
          frame #1 {
            # "*"
            n190 = Wait (ms)(milliseconds to wait=u32 2000) -> ()  [unwired: 1 out]
            n191 = call "String_in_Reference.vi"("String"="Starting Test Log..." ("string")) -> ()  [unwired: 18 in, 1 out]
          }
          frame #2 {
            w404 = TRUE ("Init Complete")
            n192 = property on="Loggin Data" class="Bool (strict)"("Val(Sgnl)"=w404) -> ()  [unwired: 2 in, 2 out]
            "Loggin Data" <- w404
          }
        }
        n193 = call <vilib>:"Add State(s) to Queue__jki_lib_state_machine.vi"("State(s) in (\"\")"=w390) -> ("States Out"=w389:string)  [unwired: 14 in]
      }
      frame "-----Start Sequence----" {
        # "Do not put any code in this frame.\n(It is a separator no-op. You can make a copy of this frame to create a new Data frame)"
        n194 = call <vilib>:"Add State(s) to Queue__jki_lib_state_machine.vi"("State(s) in (\"\")"=w408) -> ("States Out"=w407:string)  [unwired: 14 in]
      }
      frame "Off Mode Power" {
        w409 = u16 2 items=["-", "100ms", "200ms", "500ms", "1s", "2s", "5s"] ("Update Rate (3: 500ms)")
        w410 = u16 7 items=["AUTO", "500 mA", "1 A", "2 A", "5 A", "10 A", "20 A", "40 A", "S-AUTO", "50 mV", "100 mV", "200 mV", "500 mV", "1 V", "2 V", "5 V", "10 V", "250 mA", "500 mA", "1 A", "2.5 A", "5 A", "10 A", "20 A", "25 mV", "50 mV", "100 mV", "250 mV", "500 mV", "1 V", "2.5 V", "5 V"] ("I Range (7: 40A)")
        w411 = u16 6 items=["AUTO", "15", "30", "60", "100", "150", "300", "600", "1000", "7.5", "15", "30", "50", "75", "150", "300", "500"] ("V Range (8: 1000V)")
        # "I am thinking about an automatic\nmanual adjust...but manual will work\nfor now. I think the voltage sense wires \nare in the wrong location. The chroma reads the correct \nvoltage..but the WT500 does not."
        n195 = Unbundle By Name(w419) -> ("Equipment.Power"=w415:T7, "Power Analyzer"=w426:T9)
        n196 = Unbundle By Name(w415) -> ()  [unwired: 1 out]
        n197 = Unbundle By Name(w419) -> ("Equipment.Power.Power Supply.Chroma 61605"=w418:refnum<visa-resource-name>, "Equipment.Power.Yokogawa.WT500.Power VISA Yokogawa WT500"=w412:refnum<visa-resource-name>)
        n198 = local read "Supply Voltage:"() -> (w420:string)
        n199 = call "WT500 IEC 2015 Setup.vi"("VISA Input"=w412, "V Range (8: 1000V)"=w411, "I Range (7: 40A)"=w410, "Update Rate (3: 500ms)"=w409, "error in (no error)"=w414) -> ("error out"=w413:errorcluster)  [unwired: 6 in, 4 out]
        n200 = call "Manual Adjust Voltage.vi"("error in (no error)"=w413, "VISA resource name"=w418, "Supply Voltage:"=w420) -> ("error out"=w421:errorcluster, "L2 Adjusted"=→"L2 Adjusted":string, "L1 Adjusted"=→"L1 Adjusted":string)  [unwired: 6 in]
        n201 = call "Off Mode Standby Mode Power Measure SM.vi"("Power"=w415, "Power Analyzer"=w426, "Error In"=w421) -> ("Output File"=→"Off Mode Power Output":string[][], "Run 2015 Calculation"=→"2015?":bool, "Average Power (Watts)"=w424:dbl, "Error Out"=w423:errorcluster)  [unwired: 8 in, 1 out]
        n202 = call "DPT Worksheet DOE Audit.vi"() -> ("DOE Data Out"=w427:T25)  [unwired: 13 in, 2 out]
        n203 = Bundle By Name(cluster=w427, "Standby Power"=w424) -> (w428:T25)
        n204 = call "DPT Worksheet DOE Audit.vi"("Add?"=TRUE, "DOE Data"=w428) -> ()  [unwired: 11 in, 3 out]
        n205 = case shown="No Error" w423 {
          tunnel: ["Init: Power Analyzer" ("State(s) in Front (\"\")") "Macro: Exit" ("State(s) in Front (\"\")")] -> w431
          tunnel: w430 -> [_ w436]
          frame No Error {
          }
          frame Error {
            n206 = Concatenate Strings("Error:", w436) -> (w438:string)
            n207 = One Button Dialog(message=w438) -> ()  [unwired: 1 in, 1 out]
          }
        }
        n208 = call <vilib>:"Add State(s) to Queue__jki_lib_state_machine.vi"("State(s) in Front (\"\")"=w431, "State(s) in (\"\")"=w433) -> ("States Out"=w432:string)  [unwired: 13 in]
      }
      frame "Start: Dryer Info" {
        # "After Conditioning make sure the dryer is shut off. This is just to get ready for\nthe actual drying test. (It's a luxury, the tech could shut off..but we have communication)"
        # "2.2 Ambient temperature and humidity. Maintain the room ambient air temperature at 75 ±3 °F and the room relative humidity at 50\n±10 percent relative humidity"
        # "Before any test cycle, operate the dryer without a test load in the non-heat mode for 15 minutes\nor until the discharge air temperature is varying less than 1 °F for 10 minutes, which ever is longer, in the test installation location\nwith the ambient conditions within the specified rest condition tolerances of 2.2."
        n209 = Unbundle By Name(w448) -> ("Equipment.Power.Power Supply.Use Chroma?"=w441:bool, "Equipment.Power.Power Supply.Chroma 61605"=w442:refnum<visa-resource-name>, "Equipment"=w445:T8, "CDAQ Tasks"=w440:refnum<k21>[])
        n210 = local read "Simulate"() -> (w450:bool)
        n211 = global read "DPT Global Test Variables.vi" "Globals for Dryer Performance Test"() -> (w443:T17)
        n212 = Unbundle By Name(w443) -> ("Agilent Setup.RDB Channel"=w444:string)
        n213 = case shown="False" w450 {
          tunnel: w451 -> [w461 w497]
          tunnel: [w471 100.0 ("Cold Dryer Weight")] -> w439
          tunnel: w445 -> [w462 _]
          tunnel: w444 -> [w470 _]
          tunnel: w442 -> [w465 _]
          tunnel: [w463 w497] -> w449
          tunnel: w441 -> [w460 _]
          tunnel: w440 -> [w459 _]
          frame False {
            n214 = local read "Supply Voltage:"() -> (w469:string)
            n215 = call "DPT Panel Dryer PreCondition.vi"("Equipment"=w462, "CDAQ Tasks"=w459, "RDB Channel"=w470, "Error In"=w461) -> ("Cold Dryer Weight"=w471:dbl, "Error Out"=w464:errorcluster)  [unwired: 10 in]
            n216 = case shown="\"120\", Default" w469 {
              tunnel: [Chroma_Driver_Select."Output On 120" ("Chroma Power Select") Chroma_Driver_Select."Output On 208" ("Chroma Power Select") Chroma_Driver_Select."Output On 240" ("Chroma Power Select")] -> w467
              frame "120", Default {
              }
              frame "208" {
              }
              frame "240" {
              }
            }
            n217 = local read "L1 Adjusted"() -> (w458:string)
            n218 = local read "L2 Adjusted"() -> (w457:string)
            n219 = Build Array(Chroma_Driver_Select."Output Off" ("Chroma Power Select"), Chroma_Driver_Select."Initialize" ("Chroma Power Select"), w467) -> (w466:T22[])
            n220 = case shown="True" w460 {
              tunnel: w466 -> [_ w478]
              tunnel: w465 -> [_ w477]
              tunnel: w464 -> [w472 w476]
              tunnel: [w472 w475] -> w463
              tunnel: w458 -> [_ w474]
              tunnel: w457 -> [_ w473]
              frame False {
              }
              frame True {
                n221 = for {
                  tunnel: w477 -> [w488]
                  tunnel: w478 -> [w485] mode=indexing
                  shift-right: [w484] -> w475
                  shift-left: w476 -> [w487]
                  tunnel: w474 -> [w480]
                  tunnel: w473 -> [w479]
                  i -> [w483]
                  n222 = Equal To 0?(x=w483) -> (x = 0?=w482:bool)
                  n223 = call "Chroma 617xx Driver GPIB-VISA-RW.vi"("VISA resource name"=w488, "L1 Adjusted"=w480, "L2 Adjusted"=w479, "Chroma Power Select"=w485, "Use Adjusted Voltage"=TRUE, "error in (no error)"=w487) -> ("error out"=w486:errorcluster)  [unwired: 8 in, 1 out]
                  n224 = case shown="True" w482 {
                    tunnel: w486 -> [w489 w492]
                    tunnel: [w489 w491] -> w484
                    frame False {
                    }
                    frame True {
                      n225 = call "UTILITY Delay mS.vi"("Error In"=w492, "milliseconds to wait"=u32 7000) -> ("Error Out"=w491:errorcluster)  [unwired: 13 in]
                    }
                  }
                }
              }
            }
          }
          frame True {
          }
        }
        "Empty Dryer Cold Weight (lbs)" <- w439
        n226 = Bundle By Name(cluster=w443, "Test Information.Empty Dryer Cold Weight:"=w439) -> (w446:T17)
        n227 = global write "DPT Global Test Variables.vi" "Globals for Dryer Performance Test"(w446) -> ()
        n228 = Bundle By Name(cluster=w448, "Empty Dryer Cold Weight"=w439) -> (w447:T24)
        n229 = case shown="No Error" w449 {
          tunnel: ["" ("State(s) in Front (\"\")") "Macro: Exit" ("State(s) in Front (\"\")")] -> w453
          tunnel: w452 -> [_ w500]
          frame No Error {
          }
          frame Error {
            n230 = Concatenate Strings("Error:", w500) -> (w502:string)
            n231 = One Button Dialog(message=w502) -> ()  [unwired: 1 in, 1 out]
          }
        }
        n232 = call <vilib>:"Add State(s) to Queue__jki_lib_state_machine.vi"("State(s) in Front (\"\")"=w453, "State(s) in (\"\")"=w455) -> ("States Out"=w454:string)  [unwired: 13 in]
      }
      frame "Start: Gas Reading" {
        n233 = local read "Simulate"() -> (w511:bool)
        n234 = global read "DPT Global Test Variables.vi" "Globals for Dryer Performance Test"() -> (w506:T17)
        n235 = Unbundle By Name(w506) -> ("Test Information.Dryer Type"=w507:string)
        n236 = Not Equal?(x="Gas", y=w507) -> (x != y?=w503:bool)
        n237 = Or(x=w503, y=w511) -> (x .or. y?=w504:bool)
        n238 = case shown="False" w504 {
          tunnel: w512 -> [w528 w541]
          tunnel: [w528 w541] -> w508
          tunnel: w510 -> [w539 _]
          tunnel: w510 -> [w534 w540]
          tunnel: [w533 w540] -> w509
          frame False {
            n239 = Unbundle By Name(w539) -> ("Start Header Data"=w532:string[][], "CDAQ Tasks"=w521:refnum<k21>[])
            n240 = call "DPT GET NI Data.vi"("Tasks In"=w521) -> ("cDAQ Data"=w520:string[][])  [unwired: 9 in, 1 out]
            n241 = Index Array(array=w520, index (row)=2 ("disabled index (row)"), index (col)=1 ("disabled index (col)")) -> (element=w517:string)
            n242 = Fract/Exp String To Number(string=w517) -> (number=w523:dbl)  [unwired: 3 in, 1 out]
            n243 = local read "2015?"() -> (w522:bool)
            n244 = call "DPT Worksheet DOE Audit.vi"() -> ("DOE Data Out"=w526:T25)  [unwired: 13 in, 2 out]
            n245 = Bundle By Name(cluster=w526, "Gas Vol Init"=w523) -> (w525:T25)
            n246 = call "DPT Worksheet DOE Audit.vi"("2015?"=w522, "Add?"=TRUE, "DOE Data"=w525) -> ()  [unwired: 10 in, 3 out]
            n247 = Build Array(w517) -> (w538:string[])
            n248 = Build Array("Dry Meter Initial Reading") -> (w537:string[])
            n249 = Build Array (concatenate)(w538) -> (w535:string[])
            n250 = Build Array (concatenate)(w537) -> (w536:string[])
            n251 = Build Array(w536, w535) -> (w530:string[][])
            n252 = Transpose 2D Array(2D array=w530) -> (transposed array=w529:string[][])
            n253 = Build Array (concatenate)(w532, w529) -> (w531:string[][])
            n254 = Bundle By Name(cluster=w534, "Start Header Data"=w531) -> (w533:T24)
          }
          frame True {
          }
        }
        n255 = case shown="No Error" w508 {
          tunnel: ["" ("State(s) in Front (\"\")") "Macro: Exit" ("State(s) in Front (\"\")")] -> w514
          tunnel: w513 -> [_ w544]
          frame No Error {
          }
          frame Error {
            n256 = Concatenate Strings("Error:", w544) -> (w546:string)
            n257 = One Button Dialog(message=w546) -> ()  [unwired: 1 in, 1 out]
          }
        }
        n258 = call <vilib>:"Add State(s) to Queue__jki_lib_state_machine.vi"("State(s) in Front (\"\")"=w514, "State(s) in (\"\")"=w516) -> ("States Out"=w515:string)  [unwired: 13 in]
      }
      frame "Start: Ambient" {
        n259 = local read "Simulate"() -> (w550:bool)
        n260 = case shown="False" w550 {
          tunnel: w551 -> [w572 w599]
          tunnel: [w571 w599] -> w547
          tunnel: w549 -> [w580 _]
          tunnel: w549 -> [w579 w598]
          tunnel: [w578 w598] -> w548
          frame False {
            n261 = local read "ITHX RH Sensor"() -> (w558:bool)
            n262 = Unbundle By Name(w580) -> ("Start Header Data"=w577:string[][], "CDAQ Tasks"=w556:refnum<k21>[])
            n263 = case shown="False" w558 {
              tunnel: w572 -> [w587 w597]
              tunnel: [w583 w596] -> w571
              tunnel: [w581 w590] -> w563
              tunnel: [w582 w591] -> w560
              tunnel: w556 -> [w589 _]
              frame False {
                # "M.S.-Try to do unbundle to get Data Out, \ninstead of the current element index thing"
                n264 = call "cDAQ GET Module Temps.vi"("error in (no error)"=w587, "Module Number"=6, "Tasks (In)"=w589) -> ("error out"=w583:errorcluster, "Raw Data"=w586:dbl[])  [unwired: 5 in, 2 out]
                n265 = Index Array(array=w586, index #1=3 ("index"), index #2=4 ("index")) -> (element #1=w582:dbl, element #2=w581:dbl)
              }
              frame True {
                n266 = global read "DPT Global Test Variables.vi" "Globals for Dryer Performance Test"() -> (w594:T17)
                n267 = Unbundle By Name(w594) -> ("Test Setup.RH-IP"=w595:string)
                n268 = call "Newport ITX-D3N.vi"("error in (no error)"=w597, "Machine"=w595) -> ("error out"=w596:errorcluster, "Temp/Humidity"=w593:dbl[])  [unwired: 6 in, 2 out]
                n269 = Array To Cluster(array=w593) -> (cluster=w592:T27)
                n270 = Unbundle(w592) -> ("Temp/Humidity[0]"=w591:dbl, "Temp/Humidity[1]"=w590:dbl)
              }
            }
            n271 = Number To Fractional String(number=w560, precision (6)=i16 1) -> (F-format string=w559:string)  [unwired: 2 in]
            n272 = Number To Fractional String(number=w563, precision (6)=i16 1) -> (F-format string=w562:string)  [unwired: 2 in]
            n273 = call "DPT Worksheet DOE Audit.vi"() -> ("DOE Data Out"=w565:T25)  [unwired: 13 in, 2 out]
            n274 = Bundle By Name(cluster=w565, "Ambinet Temp"=w559, "Ambinet RH"=w562) -> (w566:T25)
            n275 = Build Array(w559, w562) -> (w568:string[])
            n276 = local read "2015?"() -> (w557:bool)
            n277 = call "DPT Worksheet DOE Audit.vi"("2015?"=w557, "Add?"=TRUE, "DOE Data"=w566) -> ()  [unwired: 10 in, 3 out]
            n278 = Build Array("Ambient Temp", "Ambient RH") -> (w569:string[])
            n279 = Build Array(w569, w568) -> (w575:string[][])
            n280 = Transpose 2D Array(2D array=w575) -> (transposed array=w574:string[][])
            n281 = Build Array (concatenate)(w577, w574) -> (w576:string[][])
            n282 = Bundle By Name(cluster=w579, "Start Header Data"=w576) -> (w578:T24)
          }
          frame True {
          }
        }
        n283 = case shown="Error" w547 {
          tunnel: ["" ("State(s) in Front (\"\")") "Macro: Exit" ("State(s) in Front (\"\")")] -> w553
          tunnel: w552 -> [_ w602]
          frame No Error {
          }
          frame Error {
            n284 = Concatenate Strings("Error:", w602) -> (w604:string)
            n285 = One Button Dialog(message=w604) -> ()  [unwired: 1 in, 1 out]
          }
        }
        n286 = call <vilib>:"Add State(s) to Queue__jki_lib_state_machine.vi"("State(s) in Front (\"\")"=w553, "State(s) in (\"\")"=w555) -> ("States Out"=w554:string)  [unwired: 13 in]
      }
      frame "Start: Files" {
        # "Preceeded by:\n Dryer Weight setting in Global."
        # "Alter File Init subvi per application to get a dialog box that gives you \nyour data filename."
        n287 = Unbundle By Name(w625) -> ("Equipment.Scale Com Port"=w609:refnum<visa-resource-name>, "Start Header Data"=w623:string[][])
        n288 = global read "DPT Global Test Variables.vi" "Globals for Dryer Performance Test"() -> (w613:T17)
        n289 = Unbundle By Name(w613) -> ("Directories.Work File Directory"=w612:path)
        "Work File Directory" <- w612
        n290 = local read "FileVersionInfo Out"() -> (w621:T15)
        n291 = Unbundle By Name(w621) -> ("ProductName"=w631:string, "FileVersion"=w630:string)
        n292 = call "DPT File Setup.vi"("Data File Directory"=w612, "Test_Type:"=w631, "Version In:"=w630, "Supply Voltage:"="Supply Voltage:", "error in (no error)"=w622, "File Extension:"="xlsx", "Scale Com Port"=w609, "Flow Computer Info Baro,BTUF,u,Z"=w623) -> ("FileInit Cluster"=→"FileInit Cluster":T6, "Weights Out"=w624:T28, "FileName"=w615:path, "Nominal Load  Weight"=w610:string, "error out"=w619:errorcluster)  [unwired: 7 in]
        "FileName DataLog" <- w615
        n293 = Bundle By Name(cluster=w625, "Dryer Load Nominal Weight"=w610) -> (w611:T24)
        n294 = Unbundle By Name(w624) -> ("Actual RMC"=w608:dbl, "Bone Dry Wt(lbs)"=w607:dbl, "Measured IMC"=w606:dbl)
        "Bone Dry Weight (lbs)" <- w607
        "Wet Clothing Weight (lbs)" <- w606
        n295 = Strip Path(path=w615) -> (name=→"Data Filename":string)  [unwired: 1 out]
        n296 = local write "Relative Moisture Content (%)"(w608) -> ()
        n297 = Equal?(x=path "", y=w615) -> (x = y?=w614:bool)
        n298 = Unbundle By Name(w619) -> ("status"=w617:bool)
        n299 = flat-sequence {
          tunnel: w607 -> [w637]
          tunnel: w606 -> [w636]
          frame #0 {
            n300 = local read "2015?"() -> (w634:bool)
            n301 = call "DPT Worksheet DOE Audit.vi"() -> ("DOE Data Out"=w639:T25)  [unwired: 13 in, 2 out]
            n302 = Bundle By Name(cluster=w639, "Bone Dry Wt"=w637, "Initial Wt"=w636) -> (w638:T25)
            n303 = call "DPT Worksheet DOE Audit.vi"("2015?"=w634, "Add?"=TRUE, "DOE Data"=w638) -> ()  [unwired: 10 in, 3 out]
          }
        }
        n304 = Or(x=w614, y=w617) -> (x .or. y?=w618:bool)
        n305 = case shown="False" w618 {
          tunnel: ["" ("State(s) in Front (\"\")") "Macro: Exit" ("State(s) in Front (\"\")")] -> w626
          tunnel: w627 -> [_ w643]
          frame False {
            w640 = TRUE
            n306 = property on="Write to File" class="Bool (strict)"("Val(Sgnl)"=w640) -> ()  [unwired: 2 in, 2 out]
            "Write to File" <- w640
          }
          frame True {
            n307 = Concatenate Strings("Error:", w643) -> (w645:string)
            n308 = One Button Dialog(message=w645) -> ()  [unwired: 1 in, 1 out]
          }
        }
        n309 = call <vilib>:"Add State(s) to Queue__jki_lib_state_machine.vi"("State(s) in Front (\"\")"=w626, "State(s) in (\"\")"=w633) -> ("States Out"=w632:string)  [unwired: 13 in]
      }
      frame "Get Offset Coeff" {
        # "w45 is the weight shift 45 seconds into the test.  The dryer scales have up to a 40 second averaging filter.\nAt 45 seconds after the dryer starts, take the weight adjusted for temp, and subtract from initial conditions.\nThis shift is correlated to the error at the end, depending on the load size."
        # "The conversion of weight to real weight:\n\nBase on load weight (first col).\nCoef of initial weight shift (second col.)\nOffset based on average error seen.  3rd col\nVolume used for temp calculations 4th col."
        n310 = global read "DPT Global Test Variables.vi" "Globals for Dryer Performance Test"() -> (w648:T17)
        n311 = Unbundle By Name(w648) -> ("Test Setup.T45_Coeff."=→"Init Offset Coeff":dbl, "Test Setup.Weight Offset"=→"Offset":dbl)
        n312 = call <vilib>:"Add State(s) to Queue__jki_lib_state_machine.vi"("State(s) in (\"\")"=w652) -> ("States Out"=w651:string)  [unwired: 14 in]
      }
      frame "Start: Time" {
        n313 = call "DPT Panel Stop Condition.vi"() -> ("Enable Time Limit Out"=→"Enable Time Limit":bool, "Time Limit(s) Out"=→"Time Limit(s)":dbl, "Enable RMC Limit Out"=→"Enable RMC Limit":bool, "RMC Limit Out"=→"RMC Limit":dbl, "Enable Stop On Power Off Out"=→"Enable Stop On Power Off":bool, "Power Off Time(samples) Out"=→"Power Off Time(samples)":i32, "Power Off Check"=→"Power Off Check":bool[])  [unwired: 9 in]
        n314 = call <vilib>:"Add State(s) to Queue__jki_lib_state_machine.vi"("State(s) in (\"\")"=w663) -> ("States Out"=w662:string)  [unwired: 14 in]
      }
      frame "---------- Data ----------" {
        # "Do not put any code in this frame.\n(It is a separator no-op. You can make a copy of this frame to create a new Data frame)"
        n315 = call <vilib>:"Add State(s) to Queue__jki_lib_state_machine.vi"("State(s) in (\"\")"=w667) -> ("States Out"=w666:string)  [unwired: 14 in]
      }
      frame "Data: Initialize" {
        w673 = ""  # Dryer Load Nominal Weight
        w668 = ""  # Dryer Type
        w674 = string[][] []  # Start Header Data
        w675 = 0.0  # Empty Dryer Cold Weight
        w676 = "240/120"  # Supply Voltage:
        w677 = string[] []  # DAQ Label List
        w678 = ""  # DAQ Chan List
        w679 = T8 {"Scale Com Port"="COM1", "Com Flow Computer"="COM1", "Com Power Meter"="COM1", "Com Power Supply"="", "Power "={"Yokogawa"={"WT210"={"Sample Rate (1: 0.25s)"=0, "A Range (12: 20A)"=0, "V Range (6: 600V)"=0, "Power VISA Yokogawa WT210"=""}, "WT500"={"Power VISA Yokogawa WT500"="", "V Range (8: 1000V)"=0, "I Range (7: 40A)"=0, "Update Rate (3: 500ms)"=0}}, "Aplus"={"Aplus IP Address"="", "Remote Port"=0, "Instrument"="", "Instr Driver Revision"=""}, "Power Limits"={"Crest Factor"={"Upper Limit"=0.0, "Lower Limit"=0.0}, "Harmonic Content"={"Uthd"=0.0}, "Voltage"={"% Error"=0.0}, "Stability"={"<1 Watt "={"Wattage"=0.0, "Slope (mW/H)"=0.0}, ">1 Watt"={"1%Power/Hour"=0.0}}}, "Nominal Voltage"=0, "Time Limit (s)"=0.0, "Power Variation Limit (%)"=0.0, "Power Supply"={"Chroma 61605"="", "Use Chroma?"=FALSE}}}  # Equipment
        w680 = path "C:/work/DryerPerformanceTest.ini"  # Config File Path
        w681 = path "c:/palceholder.csv"  # FileName
        w683 = errorcluster[] []  # Error Log
        w684 = T29 {"Current VI Reference"=refnum, "Close Panel on Exit?"=FALSE}  # Core
        # "Next update make this \nvariable. It is currently the\ndefault value"
        # "Config File Name"
        # "Initialize the shift-register data, here.\n(data names are defined by what you wire into the bundle function)"
        n316 = local write "Tab Control"(T10."                           Data  " ("Tab Control")) -> ()
        n317 = call <vilib>:"Add State(s) to Queue__jki_lib_state_machine.vi"("State(s) in (\"\")"=w687) -> ("States Out"=w686:string)  [unwired: 14 in]
        n318 = Bundle("Core"=w684, "Error Log"=w683, "FileName"=w681, "Config File Path"=w680, "Standby Power Settings"="Standby Power Settings", "Equipment"=w679, "DAQ Chan List"=w678, "DAQ Label List"=w677, "Supply Voltage:"=w676, "Empty Dryer Cold Weight"=w675, "Start Header Data"=w674, "Dryer Type"=w668, "Dryer Load Nominal Weight"=w673, "Power Analyzer"="Power Analyzer", "CDAQ Tasks"="CDAQ Tasks") -> (w685:T24)  [unwired: 1 in]
      }
      frame "Data: Cleanup" {
        # "Cleanup any data and references, here.\n(this is called automatically, by the Macro: Exit)"
        n319 = Unbundle By Name(w696) -> ("Core.Current VI Reference"=w695:refnum<vi>, "Equipment.Com Flow Computer"=w692:refnum<visa-resource-name>, "Equipment.Power.Yokogawa.WT500.Power VISA Yokogawa WT500"=w690:refnum<visa-resource-name>, "Equipment.Power.Power Supply.Chroma 61605"=w689:refnum<visa-resource-name>)
        n320 = flat-sequence {
          tunnel: w695 -> [w712]
          tunnel: w694 -> [w711]
          tunnel: [w705] -> w693
          tunnel: w692 -> [w710]
          tunnel: w688 -> [w708]
          tunnel: [w706] -> w691
          frame #0 {
            w699 = TRUE ("Finish")
            n321 = Not(x=w699) -> (.not. x?=w700:bool)
            n322 = property on="End1_Main" class="Bool (strict)"("Val(Sgnl)"=w699) -> ()  [unwired: 2 in, 2 out]
            n323 = local write "Start Test"(w700) -> ()
            "End1_Main" <- w699
          }
          frame #1 {
            n324 = disable-structure shown="Disabled" {
              frame Disabled {
                n325 = while {
                  stop <- w704 stop-if-true
                  n326 = local read "End2_DAQ"() -> (w703:bool)
                  n327 = local read "Eng3_Log"() -> (w702:bool)
                  n328 = Compound Arithmetic op=AND(w703, w702) -> (w704:bool)
                  n329 = Wait (ms)(milliseconds to wait=u32 150) -> ()  [unwired: 1 out]
                }
              }
              frame Enabled {
              }
            }
          }
          frame #2 {
            n330 = for {
              tunnel: w708 -> [w716] mode=indexing
              n331 = VISA Close(VISA resource name=w716) -> ()  [unwired: 1 in, 1 out]
            }
            n332 = local read "Use SL9200 Gas Readings?"() -> (w709:bool)
            n333 = case shown="True" w709 {
              tunnel: w710 -> [_ w718]
              frame False {
              }
              frame True {
                n334 = call "SL9200 Driver SM.vi"("ComPort"=w718, "Close Com"=TRUE) -> ()  [unwired: 11 in, 3 out]
              }
            }
            n335 = Close Reference(reference=w712, error in (no error)=w711) -> (error out=w707:errorcluster)
            n336 = case shown="No Error" w707 {
              selector: w707 -> [w713 w714]
              tunnel: [_ "Exit" ("State(s) in Front (\"\")")] -> w706
              tunnel: [w713 _] -> w705
              frame No Error {
              }
              frame Error {
                n337 = call <vilib>:"Simple Error Handler.vi"("error in (no error)"=w714) -> ()  [unwired: 4 in, 5 out]
              }
            }
          }
        }
        n338 = Build Array(w690, w689) -> (w688:refnum<visa-resource-name>[])
        n339 = call <vilib>:"Add State(s) to Queue__jki_lib_state_machine.vi"("State(s) in Front (\"\")"=w691, "State(s) in (\"\")"=w698) -> ("States Out"=w697:string)  [unwired: 13 in]
      }
      frame "---------- UI ----------" {
        # "Do not put any code in this frame.\n(It is a separator no-op. You can make a copy of this frame to create a new UI frame)"
        n340 = call <vilib>:"Add State(s) to Queue__jki_lib_state_machine.vi"("State(s) in (\"\")"=w722) -> ("States Out"=w721:string)  [unwired: 14 in]
      }
      frame "UI: Front Panel State" {
        # "Argument"
        # "Set Front Panel Open or Closed\n(Usage: \"UI: Front Panel State >> Open|Close|Minimize\")"
        n341 = Unbundle By Name(w726) -> ("Core.Current VI Reference"=w725:refnum<vi>)
        n342 = case shown="True" "Close when complete" {
          tunnel: w728 -> [w731 w735]
          tunnel: [w731 w734] -> w727
          tunnel: w725 -> [_ w733]
          tunnel: w724 -> [_ w732]
          frame False {
          }
          frame True {
            n343 = case shown="\"Open\", Default" w732 {
              tunnel: w735 -> [w738 w742 w750]
              tunnel: [w740 w745 w751] -> w734
              tunnel: w733 -> [w739 w741 w748]
              frame "Open", Default {
                n344 = invoke class="VI" method="FP.Open"(reference=w739, error in=w738, "Activate"=TRUE, "State"=T23."Maximized") -> (error out=w740:errorcluster)  [unwired: 1 in, 4 out]
              }
              frame "Minimize" {
                n345 = invoke class="VI" method="FP.Open"(reference=w741, error in=w742, "Activate"=TRUE, "State"=T23."Minimized") -> (error out=w745:errorcluster)  [unwired: 1 in, 4 out]
              }
              frame "Close" {
                n346 = property class="VI"(reference=w748, error in=w750) -> (reference out=w747:refnum<vi>, error out=w749:errorcluster, "Front Panel.Open"=w746:bool)
                n347 = case shown="True" w746 {
                  tunnel: [w752 w755] -> w751
                  tunnel: w749 -> [w752 w754]
                  tunnel: w747 -> [_ w753]
                  frame False {
                  }
                  frame True {
                    n348 = invoke class="VI" method="FP.Close"(reference=w753, error in=w754) -> (error out=w755:errorcluster)  [unwired: 1 in, 2 out]
                  }
                }
              }
            }
          }
        }
        n349 = call <vilib>:"Add State(s) to Queue__jki_lib_state_machine.vi"("State(s) in (\"\")"=w730) -> ("States Out"=w729:string)  [unwired: 14 in]
      }
      frame "-------Config File------" {
        # "Do not put any code in this frame.\n(It is a separator no-op. You can make a copy of this frame to create a new Data frame)"
        n350 = call <vilib>:"Add State(s) to Queue__jki_lib_state_machine.vi"("State(s) in (\"\")"=w759) -> ("States Out"=w758:string)  [unwired: 14 in]
      }
      frame "Config: Read" {
        w769 = FALSE  # Write?
        # "Read Globals from Config File.\n(This file will be customized per application)"
        n351 = Unbundle By Name(w762) -> ("Config File Path"=w768:path)
        n352 = call "DPT Global Cluster Read Write.vi"("Write?"=w769, "error in (no error)"=w771, "configuration file path"=w768) -> ("error out"=w770:errorcluster, "Test Config Out"=w764:T17)  [unwired: 7 in]
        n353 = global write "DPT Global Test Variables.vi" "Globals for Dryer Performance Test"(w764) -> ()
        n354 = local write "Globals for Dryer Performance Test"(w764) -> ()
        n355 = Unbundle By Name(w764) -> ("Test Setup.Scale Com"=w767:dbl, "Test Setup.Smoothing"=→"Use Smoothing":bool, "Test Setup.CDAQ"=→"cDAQ":bool)  [unwired: 1 out]
        n356 = To Unsigned Byte Integer(number=w767) -> (unsigned 8bit integer=w766:u8)
        n357 = call "UTILITY Com Chan Type Conversion.vi"("Com Chan"=w766) -> ("VISA resource name"=w760:refnum<visa-resource-name>)  [unwired: 11 in, 3 out]
        "Scale Com Port" <- w760
        n358 = Bundle By Name(cluster=w762, "Equipment.Scale Com Port"=w760) -> (w761:T24)
        n359 = disable-structure shown="Disabled" {
          frame Disabled {
            n360 = local read item#-1() -> ()  [unwired: 1 in]
          }
          frame Enabled {
          }
        }
        n361 = call <vilib>:"Add State(s) to Queue__jki_lib_state_machine.vi"("State(s) in (\"\")"=w773) -> ("States Out"=w772:string)  [unwired: 14 in]
      }
      frame "Config: Write" {
        # "Write Globals to Config File.\n(This file will be customized per application)"
        n362 = Unbundle By Name(w779) -> ("Config File Path"=w778:path)
        n363 = global read "DPT Global Test Variables.vi" "Globals for Dryer Performance Test"() -> (w774:T17)
        "Globals for Dryer Performance Test" <- w774
        n364 = call "DPT Global Cluster Read Write.vi"("Write?"=TRUE, "error in (no error)"=w777, "configuration file path"=w778, "Test Config In"=w774) -> ("error out"=w776:errorcluster)  [unwired: 6 in, 1 out]
        n365 = call <vilib>:"Add State(s) to Queue__jki_lib_state_machine.vi"("State(s) in (\"\")"=w781) -> ("States Out"=w780:string)  [unwired: 14 in]
      }
      frame "---------- Macro ----------" {
        # "Do not put any code in this frame.\n(It is a separator no-op. You can make a copy of this frame to create a new Macro frame)"
        n366 = call <vilib>:"Add State(s) to Queue__jki_lib_state_machine.vi"("State(s) in (\"\")"=w785) -> ("States Out"=w784:string)  [unwired: 14 in]
      }
      frame "Macro: Initialize" {
        # "Initialization Macro\n(This is called once, when the VI starts)"
        n367 = call <vilib>:"Add State(s) to Queue__jki_lib_state_machine.vi"("State(s) in Front (\"\")"="Data: Initialize\nInitialize Core Data\nUI: Front Panel State >> Minimize", "State(s) in (\"\")"=w790) -> ("States Out"=w789:string)  [unwired: 13 in]
      }
      frame "Macro: Exit" {
        w800 = "\n"
        w802 = "Stopping Test" ("String")
        # "Exit Macro\n(This is called once, when the VI exits)"
        n368 = Unbundle By Name(w804) -> ("Core.Close Panel on Exit?"=w796:bool)
        n369 = local read "exe?"() -> (w795:bool)
        n370 = call "String_in_Reference.vi"("String"=w802) -> ()  [unwired: 18 in, 1 out]
        n371 = local write "Status Message"(w802) -> ()
        n372 = Compound Arithmetic op=AND(w796, w795) -> ()  [unwired: 1 out]
        n373 = Select(t="UI: Front Panel State >> Close", s=FALSE, f="") -> (s? t:f=w799:string)
        n374 = property on="Quit" class="Bool (strict)"("Val(Sgnl)"=TRUE ("Value (Signaling)")) -> ()  [unwired: 2 in, 2 out]
        n375 = Concatenate Strings("Data: Cleanup", w800, w799, w800, "Exit") -> (w797:string)
        n376 = local write "End Test"(FALSE ("End Test")) -> ()
        n377 = call <vilib>:"Add State(s) to Queue__jki_lib_state_machine.vi"("State(s) in Front (\"\")"=w797, "State(s) in (\"\")"=w807) -> ("States Out"=w806:string)  [unwired: 13 in]
      }
      frame "---------- Test ----------" {
        n378 = call <vilib>:"Add State(s) to Queue__jki_lib_state_machine.vi"("State(s) in (\"\")"=w811) -> ("States Out"=w810:string)  [unwired: 14 in]
      }
      frame "Test: Main" {
        # "Wait for the test to complete.  Either the button is pressed, or RMC limit is reached, or the time is reached, or the power is off."
        # "Use this as a test to see if the test is complete.  If not, continue to wait."
        n379 = local read "Data Process RMC Counter"() -> (w812:dbl)
        n380 = local read "Enable RMC Limit"() -> (w816:bool)
        n381 = local read "Enable Stop On Power Off"() -> (w814:bool)
        n382 = local read "Power On One Shot"() -> (w817:bool)
        n383 = local write "Loggin Data"(TRUE ("Init Complete")) -> ()
        n384 = local read "Enable Time Limit"() -> (w815:bool)
        n385 = Compound Arithmetic op=AND(w816, w817) -> (w818:bool)
        n386 = And(x=w814, y=w817) -> (x .and. y?=w821:bool)
        n387 = case shown="True" w818 {
          tunnel: [FALSE w841] -> w813
          tunnel: w812 -> [_ w838]
          frame False {
          }
          frame True {
            # "Let the scale stablize for 20 seconds"
            n388 = Greater?(x=w838, y=20.0) -> (0:w836:bool)
            n389 = case shown="True" w836 {
              tunnel: [T12 100.0 ("Relative Moisture Content (%)") w843] -> w839
              frame False {
              }
              frame True {
                n390 = local read "Relative Moisture Content (%)"() -> (w843:T12)
              }
            }
            n391 = local read "RMC Limit"() -> (w840:dbl)
            n392 = Greater?(x=w840, y=w839) -> (0:w841:bool)
          }
        }
        n393 = case shown="True" w821 {
          selector: w821 -> [w833 _]
          tunnel: [w833 w834] -> w820
          frame False {
          }
          frame True {
            n394 = local read "Power Off One Shot"() -> (w834:bool)
          }
        }
        n395 = case shown="True" w815 {
          tunnel: [FALSE w849] -> w826
          frame False {
          }
          frame True {
            n396 = local read "Start Time (sec)"() -> (w848:T13)
            n397 = local read "Time Limit(s)"() -> (w845:dbl)
            n398 = call "UTILITY E-Time.vi"() -> ("Elapsed Time (sec)"=w847:dbl)  [unwired: 9 in, 2 out]
            n399 = Subtract(x=w847, y=w848) -> (x-y=w846:T13)
            n400 = Greater?(x=w846, y=w845) -> (0:w849:bool)
          }
        }
        n401 = local read "End Test"() -> (w819:T5)
        n402 = Compound Arithmetic op=OR(w826, w813, w819, w820) -> (w825:T5)
        "Test Complete?" <- w825
        n403 = case shown="True" w825 {
          tunnel: ["Test: Control Sequence" ("State(s) at Back (\"\")") "Power Off\nMacro: Exit" ("State(s) in Front (\"\")")] -> w829
          tunnel: w813 -> [_ w854]
          tunnel: w820 -> [_ w853]
          tunnel: w819 -> [_ w852]
          frame False {
          }
          frame True {
            n404 = case shown="False" w854 {
              tunnel: w853 -> [_ w865]
              tunnel: [w856 w864] -> w851
              tunnel: w852 -> [_ w863]
              frame True {
                n405 = local read "Start Time (sec)"() -> (w861:T13)
                n406 = call "UTILITY E-Time.vi"() -> ("Elapsed Time (sec)"=w862:dbl)  [unwired: 9 in, 2 out]
                n407 = Subtract(x=w862, y=w861) -> (x-y=w860:T13)
                n408 = Number To Fractional String(number=w860) -> (F-format string=w859:string)  [unwired: 3 in]
                n409 = Concatenate Strings("RMC Limit Reached: Cycle Time, ", w859, ", seconds.") -> (w856:string)
              }
              frame False {
                n410 = case shown="True" w865 {
                  tunnel: [w866 w875] -> w864
                  tunnel: w863 -> [w867 _]
                  frame False {
                    n411 = Select(t="End Button Depressed", s=w867, f="Over Time Limit") -> (s? t:f=w866:string)
                  }
                  frame True {
                    n412 = local read "Tend?"() -> (w871:dbl)
                    n413 = local read "2015?"() -> (w870:bool)
                    n414 = local read "Start Time (sec)"() -> (w880:T13)
                    n415 = Subtract(x=w871, y=w880) -> (x-y=w879:T13)
                    n416 = Number To Fractional String(number=w879) -> (F-format string=w878:string)  [unwired: 3 in]
                    n417 = call "DPT Worksheet DOE Audit.vi"() -> ("DOE Data Out"=w873:T25)  [unwired: 13 in, 2 out]
                    n418 = Bundle By Name(cluster=w873, "End Time(s)"=w871) -> (w872:T25)
                    n419 = Concatenate Strings("Power Off: Cycle Time, ", w878, ", seconds.") -> (w875:string)
                    n420 = call "DPT Worksheet DOE Audit.vi"("2015?"=w870, "Add?"=TRUE, "DOE Data"=w872) -> ()  [unwired: 10 in, 3 out]
                  }
                }
              }
            }
            "End Msg" <- w851
          }
        }
        n421 = call "String_in_Reference.vi"("String"="Running, Logging Data...") -> ()  [unwired: 18 in, 1 out]
        n422 = local read "UI Timer"() -> (w824:i32)
        n423 = To Unsigned Long Integer(number=w824) -> (unsigned 32bit integer=w823:u32)
        n424 = Wait (ms)(milliseconds to wait=w823) -> ()  [unwired: 1 out]
        n425 = call <vilib>:"Add State(s) to Queue__jki_lib_state_machine.vi"("State(s) in Front (\"\")"=w829, "State(s) in (\"\")"=w832) -> ("States Out"=w831:string)  [unwired: 13 in]
      }
      frame "Test: Control Sequence" {
        # "Main control sequence defined here."
        n426 = call <vilib>:"Add State(s) to Queue__jki_lib_state_machine.vi"("State(s) in Front (\"\")"="Test: Step 1" ("State(s) in Front (\"\")"), "State(s) in (\"\")"=w885) -> ("States Out"=w884:string)  [unwired: 13 in]
      }
      frame "Test: Step 1" {
        # "Description of Test Step.\nCheck Every Minute if you are done."
        n427 = call <vilib>:"Add State(s) to Queue__jki_lib_state_machine.vi"("State(s) in Front (\"\")"="Test: Main" ("State(s) in Front (\"\")"), "State(s) in (\"\")"=w890) -> ("States Out"=w889:string)  [unwired: 13 in]
      }
      frame "-----Functions------" {
        n428 = call <vilib>:"Add State(s) to Queue__jki_lib_state_machine.vi"("State(s) in (\"\")"=w894) -> ("States Out"=w893:string)  [unwired: 14 in]
      }
      frame "Power Off" {
        n429 = Unbundle By Name(w902) -> ("Equipment.Power.Power Supply.Chroma 61605"=w901:refnum<visa-resource-name>, "Equipment.Power.Power Supply.Use Chroma?"=w895:bool)
        n430 = local read "Simulate"() -> (w900:bool)
        n431 = case shown="False" w900 {
          tunnel: w901 -> [w913 _]
          tunnel: [w911 w919] -> w898
          tunnel: w899 -> [w912 w919]
          tunnel: w895 -> [w910 _]
          frame False {
            n432 = case shown="True" w910 {
              tunnel: w913 -> [_ w918]
              tunnel: w912 -> [w914 w917]
              tunnel: [w914 w916] -> w911
              frame False {
              }
              frame True {
                n433 = call "Chroma 617xx Driver GPIB-VISA-RW.vi"("VISA resource name"=w918, "Chroma Power Select"=Chroma_Driver_Select."Output Off", "error in (no error)"=w917) -> ("error out"=w916:errorcluster)  [unwired: 11 in, 1 out]
              }
            }
          }
          frame True {
          }
        }
        n434 = case shown="Error" w898 {
          tunnel: ["" ("State(s) in Front (\"\")") "Macro: Exit" ("State(s) in Front (\"\")")] -> w897
          tunnel: w896 -> [_ w907]
          frame No Error {
          }
          frame Error {
            n435 = Concatenate Strings("Error:", w907) -> (w909:string)
            n436 = One Button Dialog(message=w909) -> ()  [unwired: 1 in, 1 out]
          }
        }
        n437 = call <vilib>:"Add State(s) to Queue__jki_lib_state_machine.vi"("State(s) in Front (\"\")"=w897, "State(s) in (\"\")"=w904) -> ("States Out"=w903:string)  [unwired: 13 in]
      }
    }
    n438 = local read "Debug Mode"() -> (w47:bool)
    n439 = case shown="True" w47 {
      tunnel: [w61 w64] -> w51
      tunnel: w50 -> [w61 w63]
      tunnel: w48 -> [_ w62]
      frame False {
      }
      frame True {
        n440 = Build Array (concatenate)(w63, w62) -> (w64:string[])
        "Debug List Test States" <- w64
      }
    }
  }
  "error out" <- w8
  n441 = call <vilib>:"Add State(s) to Queue__jki_lib_state_machine.vi"("State(s) in (\"\")"="Data: Initialize") -> ("States Out"=w4:string)  [unwired: 14 in]
  n442 = call <vilib>:"Add State(s) to Queue__jki_lib_state_machine.vi"("State(s) in (\"\")"="Data: Initialize") -> ("States Out"=w12:string)  [unwired: 14 in]
  n443 = while "Data Acquisition Steps" {
    shift-right: [w931] -> _
    shift-left: _ -> [w930]
    shift-right: [w933] -> _
    shift-left: _ -> [w929]
    shift-right: [w932] -> _
    shift-left: w12 -> [w934]
    shift-right: [w928] -> w7
    shift-left: 0.0 ("Elapsed Time (sec)") -> [w927]
    tunnel: w19 -> [w920]
    shift-right: [w926] -> _
    shift-left: string[] [] -> [w925]
    tunnel: [w921] -> w6
    tunnel: [w920] -> w9
    stop <- w921 stop-if-true
    # "Data Log Time"
    n444 = call <vilib>:"Parse State Queue__jki_lib_state_machine.vi"("State Queue"=w934, "Error In (no error)"=w929) -> ("Remaining States"=w936:string, "Current State"=w924:string, "Arguments"=w935:string)  [unwired: 11 in]
    n445 = case shown="\"Data Acquire: Weight\"" w924 {
      selector: w924 -> [_ w970 _ _ _ _ _ _ _ _ _ _ _ _]
      tunnel: w936 -> [w950 w974 w991 w997 w1002 w1009 w1044 w1058 w1083 w1101 w1118 w1171 w1187 w1205]
      tunnel: w935 -> [_ _ _ _ _ _ _ _ _ _ _ _ _ _]
      tunnel: w930 -> [w948 w972 w984 w995 w999 _ w1042 w1059 w1079 w1097 w1114 w1175 w1191 w1199]
      tunnel: [w947 w976 errorcluster {"status"=FALSE, "code"=0, "source"=""} ("error out") w992 w1000 w1007 w1043 w1048 w1077 w1094 w1112 w1177 w1194 w1203] -> w933
      tunnel: w929 -> [w946 w975 w982 w992 w1000 w1007 w1043 w1048 w1077 w1095 w1113 w1178 w1195 w1203]
      tunnel: [w949 w973 w990 w996 w1001 w1008 w1047 w1062 w1082 w1100 w1117 w1172 w1188 w1204] -> w932
      tunnel: [_ _ _ TRUE _ w1003 _ _ _ _ _ _ _ _] -> w921
      tunnel: [w945 w972 w984 w995 w999 w1005 w1045 w1060 w1080 w1098 w1115 w1176 w1189 w1199] -> w931
      tunnel: "DAQ Timer" -> [w944 _ _ _ _ _ _ _ _ _ _ _ _ _]
      tunnel: [w942 w969 w987 w994 w998 w1006 w1046 w1061 w1081 w1099 w1116 w1179 w1196 w1200] -> w928
      tunnel: w927 -> [_ w969 w987 w994 w998 w1006 w1046 w1061 w1081 w1099 w1116 w1179 w1196 w1200]
      tunnel: w920 -> [_ _ _ _ _ w1004 _ _ _ _ _ _ _ w1198]
      frame "", "Idle" {
        n446 = call "UTILITY E-Time.vi"() -> ("Elapsed Time (sec)"=w941:dbl)  [unwired: 9 in, 2 out]
        n447 = call "UTILITY Timeout Calc.vi"("Timer"=w941, "Gather Data Period"=w944) -> ("coerced(x)"=w943:i32)  [unwired: 8 in, 1 out]
        "DAQ Delay Time" <- w943
        n448 = event shown="[0] Timeout;  \"Get Data Interrupt\": Value Change" {
          selector: _ -> [_]
          dyn-events: _ -> [_]
          timeout: w943 -> [_]
          tunnel: w950 -> [w959]
          tunnel: [w958] -> w949
          tunnel: w948 -> [w956]
          tunnel: [w957] -> w947
          tunnel: w946 -> [w957]
          tunnel: [w956] -> w945
          tunnel: [w953] -> w942
          event Timeout; "Get Data Interrupt": Value Change {
            w952 = "Data Acquire: Init\nData Acquire: CDAQ\nData Acquire: Power\nData Acquire: Gas\nData Acquire: RH\nData Acquire: Weight\nData Acquire: Door Switch\nData: Queue"  # Data Acquisition Steps
            # "Edit Data Acquisition Steps.\n(These are the steps used to gather the data.)"
            n449 = event-data() -> ()  [unwired: 1 in, 1 out]
            n450 = local read "Loggin Data"() -> (w955:bool)
            n451 = call "UTILITY E-Time.vi"() -> ("Elapsed Time (sec)"=w953:dbl)  [unwired: 9 in, 2 out]
            n452 = case shown="True" w955 {
              tunnel: [w961 w966] -> w954
              tunnel: w953 -> [_ _]
              tunnel: w952 -> [_ w964]
              frame False {
                n453 = local read "End1_Main"() -> (w960:bool)
                n454 = case shown="False" w960 {
                  tunnel: ["" " Exit"] -> w961
                  frame False {
                  }
                  frame True {
                  }
                }
              }
              frame True {
                n455 = local read "End1_Main"() -> (w965:bool)
                n456 = case shown="True" w965 {
                  tunnel: [w967 "Exit"] -> w966
                  tunnel: w964 -> [w967 _]
                  frame False {
                  }
                  frame True {
                  }
                }
              }
            }
            n457 = local write "Get Data Interrupt"(FALSE ("Get Data Interrupt")) -> ()
            n458 = call <vilib>:"Add State(s) to Queue__jki_lib_state_machine.vi"("State(s) in Front (\"\")"=w954, "State(s) in (\"\")"=w959) -> ("States Out"=w958:string)  [unwired: 13 in]
          }
        }
      }
      frame Default {
        w979 = 42 items=["No error", "Argument error", "Memory is full", "Out of zone", "End of file", "File already open", "Generic file I/O error", "File not found", "File permission error", "Disk is full", "Duplicate path", "Too many files open", "System feature not enabled", "Resource file not found", "Cannot add resource", "Resource not found", "Image not found", "Image memory error", "Pen does not exist", "Config type invalid", "Config token not found", "Config parse error", "Config memory error", "Bad external code format", "Bad external code offset", "External code not present", "Null window", "Destroy window error", "Null menu", "Print aborted", "Bad print record", "Print driver error", "Windows error during printing", "Memory error during printing", "Print dialog error", "Generic print error", "Invalid device refnum", "Device not found", "Device parameter error", "Device unit error", "Cannot open device", "Device call aborted", "Generic error", "Cancelled by user", "Object ID too low", "Object ID too high", "Object not in heap", "Unknown heap", "Unknown object (invalid DefProc)", "Unknown object (DefProc not in table)", "Message out of range", "Invalid (null) method", "Unknown message", "Manager call not supported", "Bad address", "Network operation in progress", "Network operation timed out", "Connection is busy", "Network attribute not supported", "Network error", "Address in use", "System out of memory", "Connection aborted", "Connection refused", "Not connected", "Already connected", "Connection closed", "Initialization error (interapplication manager)", "Bad occurrence", "Wait on unbound occurrence handler", "Occurrence queue overflow", "Datalog type conflict", "Unused", "Unrecognized type (interapplication manager)", "Memory corrupt", "Failed to make temporary DLL", "Old CIN version", "Drag socket not found", "Failed to load drop-object", "Failed to register OLE object", "Failed to release OLE object", "Format specifier type mismatch", "Unknown format specifier", "Too few format specifiers", "Too many format specifiers", "Scan failed", "Newer CIN version", "Error converting to variant", "Runtime menu error", "Password tampered", "Variant attribute not found", "Incompatible variant data type", "Event data is not available", "Event Store is not present", "Occurrence is not found", "Event Queue is not created", "Event info is not available", "Refnum passed is NULL", "Error retrieving Class GUID", "Error retrieving CoClass GUID", "Error retrieving TypeLib GUID.", "Bad built application magic bytes.", "Specific driver is different from the specific driver associated with the Logical Name.", "There is no session opened to the class driver.", "Max Error", "MAX - Error with config objects", "MAX - Error loading configuration", "MAX - Group not supported"]
        # "Current State"
        # "Do not delete, rename, or modify this frame.\n(this is used to capture unhandled states and typos)"
        # "Handle mistyped state name (developer tool)"
        n459 = Format Into String(format string="Software Exception: Unhandled State \"%s\"." ("message"), error in=w975, w970) -> (resulting string=w978:string, error out=w977:errorcluster)  [unwired: 1 in]
        n460 = call <vilib>:"Error Cluster From Error Code.vi"("show call chain? (False)"=TRUE, "error in (no error)"=w977, "error message (\"\")"=w978, "error code (0)"=w979) -> ("error out"=w976:errorcluster)  [unwired: 5 in]
        n461 = call <vilib>:"Add State(s) to Queue__jki_lib_state_machine.vi"("State(s) in (\"\")"=w974) -> ("States Out"=w973:string)  [unwired: 14 in]
      }
      frame "Error Handler" {
        # "Unhandled Error -- Display it"
        # "Handle any errors here.\nYou can also output any states to clean-up after errors occur"
        # "Clear error"
        n462 = Unbundle By Name(w984) -> ("Error Log 2"=w983:errorcluster[])
        n463 = call <vilib>:"General Error Handler.vi"("error in (no error)"=w982) -> ()  [unwired: 10 in, 5 out]
        n464 = Build Array (concatenate)(w983, w982) -> (w981:errorcluster[])
        n465 = Bundle By Name(cluster=w984, "Error Log 2"=w981) -> ()  [unwired: 1 out]
        n466 = control-ref of="This VI"() -> (w986:refnum<vi>)
        n467 = local write "Error Log 2"(w981) -> ()
        n468 = property class="VI"(reference=w986, "TB.ShowAbortBut"=TRUE ("Tool Bar:Show Abort Button")) -> ()  [unwired: 1 in, 2 out]
        n469 = call <vilib>:"Add State(s) to Queue__jki_lib_state_machine.vi"("State(s) in Front (\"\")"="/* Post Error States", "State(s) in (\"\")"=w991) -> ("States Out"=w990:string)  [unwired: 13 in]
      }
      frame "Exit" {
        n470 = call <vilib>:"Add State(s) to Queue__jki_lib_state_machine.vi"("State(s) in (\"\")"=w997) -> ("States Out"=w996:string)  [unwired: 14 in]
      }
      frame "---------- Data ----------" {
        # "Do not put any code in this frame.\n(It is a separator no-op. You can make a copy of this frame to create a new Data frame)"
        n471 = call <vilib>:"Add State(s) to Queue__jki_lib_state_machine.vi"("State(s) in (\"\")"=w1002) -> ("States Out"=w1001:string)  [unwired: 14 in]
      }
      frame "Data: Initialize" {
        # "Initialize Data.\n(This is the initialization of all of the data to be Logged.)"
        n472 = while {
          tunnel: [w1023] -> w1005
          tunnel: w1004 -> [w1022]
          tunnel: [w1015] -> w1003
          stop <- w1016 continue-if-true
          w1019 = T19 {"Data Array"=[], "Data"=[], "Date"=""}  # Q Element
          w1020 = dbl[] []  # Data Array
          # "\"Data Array\" is used for data processing in the code. \"Data\" (2D string) is for user viewing."
          # "Wait till init complete, or finish."
          n473 = Wait (ms)(milliseconds to wait=u32 150) -> ()  [unwired: 1 out]
          n474 = local read "DAQ Channel List"() -> (w1013:string)
          n475 = local read "Equipment"() -> (w1021:T8)
          n476 = Bundle(cluster=w1019, "Data Array"=w1020) -> (w1018:T19)  [unwired: 2 in]
          n477 = local read "End1_Main"() -> (w1015:bool)
          n478 = local read "Loggin Data"() -> (w1017:bool)
          n479 = Bundle("queue out"=w1022, "Q Element"=w1018, "Equipment"=w1021, "DAQ Channel List"=w1013, "Error Log 2"="Error Log 2", "Stream Data"="Stream Data", "Voltage Stream Header Output"="Voltage Stream Header Output") -> (w1023:T31)  [unwired: 1 in]
          n480 = Compound Arithmetic op=AND(invert w1015, invert w1017) -> (w1016:bool)
        }
        n481 = call <vilib>:"Add State(s) to Queue__jki_lib_state_machine.vi"("State(s) in (\"\")"=w1009) -> ("States Out"=w1008:string)  [unwired: 14 in]
      }
      frame "Data Acquire: Init" {
        # "On all of the data, we have a label in the label array, and the data in the Data array."
        # "Acquire Data Step.\n(This is an example that simulates the gathering of data.)"
        n482 = Unbundle By Name(w1042) -> ("Q Element.Data Array"=w1030:dbl[], "Q Element.Data"=w1028:string[][])
        n483 = call "UTILITY E-Time.vi"() -> ("Elapsed Time (sec)"=w1025:dbl)  [unwired: 9 in, 2 out]
        "Test Time" <- w1025
        n484 = Index Array(array=w1030, index=0) -> (element=w1040:dbl)
        n485 = Subtract(x=w1025, y=w1040) -> (x-y=→"Tsamp(s)":dbl)
        n486 = local read "DAQ Channel List"() -> (w1038:string)
        n487 = Get Date/Time In Seconds() -> (seconds since 1Jan1904=w1024:timestamp)
        n488 = Build Array("Time") -> (w1027:string[])
        n489 = Build Array(w1025) -> (w1031:dbl[])
        n490 = Get Date/Time String(seconds (now)=w1024, want seconds? (F)=TRUE) -> (date string=w1034:string, time string=w1035:string)  [unwired: 1 in]
        n491 = call "DPT Sort Data in Columns.vi"("Q Element.Data"=w1028, "DAQ Label List 2"=w1027, "Old Data Array"=w1030, "cDAQ Data Out"=w1031) -> ("Output Data"=w1026:string[][], "New Data Array"=w1032:dbl[])  [unwired: 4 in, 1 out]
        n492 = Concatenate Strings(w1034, ", " ("string"), w1035) -> (w1033:string)
        n493 = Bundle By Name(cluster=w1042, "DAQ Channel List"=w1038, "Q Element.Data"=w1026, "Q Element.Data Array"=w1032, "Q Element.Date"=w1033) -> (w1045:T31)
        n494 = call <vilib>:"Add State(s) to Queue__jki_lib_state_machine.vi"("State(s) in (\"\")"=w1044) -> ("States Out"=w1047:string)  [unwired: 14 in]
      }
      frame "Data Acquire: CDAQ" {
        # "label + data"
        # "First one begins array."
        n495 = Unbundle By Name(w1059) -> ("Q Element.Data"=w1057:string[][], "Q Element.Data Array"=w1051:dbl[])  [unwired: 1 out]
        n496 = call "cDAQ GET Module Temps.vi"("Module Number"=6) -> ()  [unwired: 7 in, 4 out]
        n497 = local read "CDAQ Tasks"() -> ()  [unwired: 1 out]
        n498 = local read "DAQ Label List"() -> (w1054:string[])
        n499 = Build Array (concatenate)(w1054, string[] ["Gas Pressure", "RH Channel", "Temp Channel", "Barometric Pressure", "Gas Feedback Chan", "Gas Temperature"]) -> (w1052:string[])
        n500 = call "DPT Sort Data in Columns.vi"("Q Element.Data"=w1057, "DAQ Label List 2"=w1052, "Old Data Array"=w1051) -> ("Output Data"=w1056:string[][], "Array"=→"cDAQ Data Out":string[], "New Data Array"=w1050:dbl[])  [unwired: 5 in]
        n501 = Bundle By Name(cluster=w1059, "Q Element.Data"=w1056, "Q Element.Data Array"=w1050) -> (w1060:T31)
        n502 = call <vilib>:"Add State(s) to Queue__jki_lib_state_machine.vi"("State(s) in (\"\")"=w1058) -> ("States Out"=w1062:string)  [unwired: 14 in]
      }
      frame "Data Acquire: Power" {
        (unwired) string[] ["VL1", "VL2", "IL1", "IL2", "P", "WH", "Ipeak", "Phi(1,2)"]
        # "Update with drivers \nrather than custom\ncommands"
        # "Acquire Data Step.\n(This is an example that simulates the gathering of data.)"
        n503 = Unbundle By Name(w1079) -> ("Q Element.Data"=w1066:string[][], "Q Element.Data Array"=w1064:dbl[], "Equipment.Power.Yokogawa.WT500.Power VISA Yokogawa WT500"=w1078:refnum<visa-resource-name>)
        n504 = call "WT500 Read Power.vi"("VISA resource name"=w1078, "WT500 CMDS"=WT500_Sequences."GetReadings") -> ("VISA resource name out"=w1069:refnum<visa-resource-name>, "PowerData"=w1076:T32, "Measurement Values"=w1068:dbl[], "Label"=w1067:string[], "error out"=w1070:errorcluster)  [unwired: 8 in, 1 out]
        n505 = call "YKWT500 Error Query.vi"("error in (no error)"=w1070, "VISA resource name"=w1069) -> ()  [unwired: 6 in, 4 out]
        n506 = Unbundle By Name(w1076) -> ("Current L1"=→"Current L1 (A)":dbl, "Current L2"=→"Current L2 (A)":dbl, "Power"=→"Power (Watts)" →"Watt Chart":dbl, "WattHours"=→"Watt Hours (Wh)":dbl)
        n507 = call "DPT Sort Data in Columns.vi"("Q Element.Data"=w1066, "DAQ Label List 2"=w1067, "Old Data Array"=w1064, "cDAQ Data Out"=w1068) -> ("Output Data"=w1065:string[][], "New Data Array"=w1063:dbl[])  [unwired: 4 in, 1 out]
        n508 = Bundle By Name(cluster=w1079, "Q Element.Data"=w1065, "Q Element.Data Array"=w1063) -> (w1080:T31)
        n509 = call <vilib>:"Add State(s) to Queue__jki_lib_state_machine.vi"("State(s) in (\"\")"=w1083) -> ("States Out"=w1082:string)  [unwired: 14 in]
      }
      frame "Data Acquire: Gas" {
        # "FIXME: VERIFY CORRECT READINGS."
        # "Acquire Data Step.\n(This is an example that simulates the gathering of data.)"
        n510 = Unbundle By Name(w1097) -> ("Q Element.Data"=w1089:string[][], "Q Element.Data Array"=w1085:dbl[], "Equipment.Com Flow Computer"=w1096:refnum<visa-resource-name>)
        n511 = local read "Use SL9200 Gas Readings?"() -> (w1092:bool)
        n512 = local read "Use Dry Gas Meter?"() -> (w1091:bool)
        n513 = call "DPT Gas Flow Readings.vi"("Com Flow Computer"=w1096, "Use SL9200 Gas Readings?"=w1092, "Use Dry Gas Meter?"=w1091, "Initialize?"=FALSE, "Error In"=w1095) -> ("Labels"=w1088:string[], "Values"=w1093:string[], "error out"=w1094:errorcluster)  [unwired: 8 in]
        n514 = Fract/Exp String To Number(string=w1093) -> (number=w1087:dbl[])  [unwired: 3 in, 1 out]
        n515 = call "DPT Sort Data in Columns.vi"("Q Element.Data"=w1089, "DAQ Label List 2"=w1088, "Old Data Array"=w1085, "cDAQ Data Out"=w1087) -> ("Output Data"=w1086:string[][], "New Data Array"=w1084:dbl[])  [unwired: 4 in, 1 out]
        n516 = Bundle By Name(cluster=w1097, "Q Element.Data"=w1086, "Q Element.Data Array"=w1084) -> (w1098:T31)
        n517 = call <vilib>:"Add State(s) to Queue__jki_lib_state_machine.vi"("State(s) in (\"\")"=w1101) -> ("States Out"=w1100:string)  [unwired: 14 in]
      }
      frame "Data Acquire: RH" {
        # "Acquire Data Step.\nAcquire data from ITHX logger if values of IP are not 0.  This should be set in the global config.\nGet RH vals.  First time thru loop, look for headers and replace values.  Otherwise, concatonate values."
        n518 = global read "DPT Global Test Variables.vi" "Globals for Dryer Performance Test"() -> (w1111:T17)
        n519 = Unbundle By Name(w1111) -> ("Test Setup.RH-IP"=w1110:string, "Test Setup.RH-IP2"=w1109:string, "Test Setup.RH-IP3"=w1108:string)
        n520 = Unbundle By Name(w1114) -> ("Q Element.Data"=w1106:string[][], "Q Element.Data Array"=w1105:dbl[])
        n521 = Build Array(w1110, w1109, w1108) -> (w1107:string[])
        n522 = for {
          tunnel: w1113 -> [w1129]
          tunnel: [w1119] -> w1112
          tunnel: w1107 -> [w1121] mode=indexing
          shift-right: [w1126] -> w1102
          shift-left: w1106 -> [w1125]
          shift-right: [w1124] -> w1104
          shift-left: w1105 -> [w1123]
          tunnel: string[][] [["Chamber Temp", "Chamber RH"], ["Probe1 Temp", "Probe1 RH"], ["Probe2 Temp", "Probe2 RH"]] ("array") -> [w1120] mode=indexing
          i -> [w1122]
          # "FIXME: VERIFY CORRECT READINGS."
          n523 = Equal?(x=w1121, y="0") -> (x = y?=w1128:bool)
          n524 = case shown="False" w1128 {
            tunnel: w1129 -> [w1136 w1164]
            tunnel: [w1137 w1164] -> w1119
            tunnel: [w1130 w1163] -> w1126
            tunnel: w1125 -> [w1134 w1163]
            tunnel: [w1131 w1162] -> w1124
            tunnel: w1123 -> [w1132 w1162]
            tunnel: w1122 -> [w1140 _]
            tunnel: w1121 -> [w1138 _]
            tunnel: w1120 -> [w1133 _]
            frame False {
              n525 = Equal To 0?(x=w1140) -> (x = 0?=w1139:bool)
              n526 = call "Newport ITX-D3N.vi"("error in (no error)"=w1136, "Machine"=w1138) -> ("error out"=w1137:errorcluster, "Temp/Humidity"=w1135:dbl[])  [unwired: 6 in, 2 out]
              "[Temp (F), RH]" <- w1135
              n527 = case shown="True" w1139 {
                tunnel: w1135 -> [w1145 w1152]
                tunnel: w1134 -> [w1144 w1151]
                tunnel: w1133 -> [w1146 w1150]
                tunnel: w1132 -> [w1142 w1149]
                tunnel: [w1141 w1148] -> w1131
                tunnel: [w1143 w1147] -> w1130
                frame False {
                  n528 = call "DPT Sort Data in Columns.vi"("Q Element.Data"=w1144, "DAQ Label List 2"=w1146, "Old Data Array"=w1142, "cDAQ Data Out"=w1145) -> ("Output Data"=w1143:string[][], "New Data Array"=w1141:dbl[])  [unwired: 4 in, 1 out]
                }
                frame True {
                  n529 = for {
                    tunnel: w1152 -> [w1161] mode=indexing
                    tunnel: w1151 -> [w1154]
                    tunnel: w1150 -> [w1160] mode=indexing
                    shift-right: [w1156] -> w1148
                    shift-left: w1149 -> [w1159]
                    tunnel: [w1153] -> w1147
                    n530 = Index Array(array=w1154, index (col)=0 ("disabled index (col)")) -> (element=w1155:string[])  [unwired: 1 in]
                    n531 = Search 1D Array(1D array=w1155, element=w1160) -> (index of element=w1158:i32)  [unwired: 1 in]
                    n532 = Replace Array Subset(array=w1159, new element=w1161, index=w1158) -> (w1156:dbl[])
                    n533 = call "DPT Sort Data in Columns.vi"("Q Element.Data"=w1154, "DAQ Label List 2"=w1155, "cDAQ Data Out"=w1156) -> ("Output Data"=w1153:string[][])  [unwired: 5 in, 2 out]
                  }
                }
              }
            }
            frame True {
              # "If the IP is configured, replace the Chamber RH\nand Temp with Ithx values.\nIf second and 3rd configured, add them."
            }
          }
        }
        n534 = Bundle By Name(cluster=w1114, "Q Element.Data"=w1102, "Q Element.Data Array"=w1104) -> (w1115:T31)
        n535 = call <vilib>:"Add State(s) to Queue__jki_lib_state_machine.vi"("State(s) in (\"\")"=w1118) -> ("States Out"=w1117:string)  [unwired: 14 in]
      }
      frame "Data Acquire: Weight" {
        n536 = Unbundle By Name(w1175) -> ("Q Element.Data Array"=w1174:dbl[], "Q Element.Data"=w1169:string[][])
        n537 = for {
          N: "W.Samps 2" -> [_]
          tunnel: "Weight Offset 2" -> [w1184]
          tunnel: [w1183] -> w1182 mode=indexing
          shift-right: [w1185] -> w1177
          shift-left: w1178 -> [w1186]
          n538 = call "Weight Input.vi"("Offset"=w1184, "Error In"=w1186) -> ("Weight"=w1183:dbl, "error out"=w1185:errorcluster)  [unwired: 9 in, 3 out]
        }
        n539 = call-poly <vilib>:"Mean.vi"("X"=w1182) -> ("mean"=w1168:dbl)  [unwired: 1 out]
        n540 = Build Array(w1168) -> (w1167:dbl[])
        n541 = Build Array("Weight") -> (w1165:string[])
        n542 = Build Array (concatenate)(w1174, w1168) -> (w1173:dbl[])
        n543 = call "DPT Sort Data in Columns.vi"("Q Element.Data"=w1169, "DAQ Label List 2"=w1165, "cDAQ Data Out"=w1167) -> ("Output Data"=w1170:string[][])  [unwired: 5 in, 2 out]
        n544 = Bundle By Name(cluster=w1175, "Q Element.Data Array"=w1173, "Q Element.Data"=w1170) -> (w1176:T31)
        n545 = call <vilib>:"Add State(s) to Queue__jki_lib_state_machine.vi"("State(s) in (\"\")"=w1171) -> ("States Out"=w1172:string)  [unwired: 14 in]
      }
      frame "Data Acquire: Door Switch" {
        n546 = Unbundle By Name(w1191) -> ("Q Element.Data Array"=w1193:dbl[])
        n547 = call "DPT Door Switch.vi"("error in (no error)"=w1195) -> ("error out"=w1194:errorcluster, "Door Switch Activation"=w1190:i16)  [unwired: 9 in]
        n548 = Build Array (concatenate)(w1193, w1190) -> (w1192:dbl[])
        n549 = Bundle By Name(cluster=w1191, "Q Element.Data Array"=w1192) -> (w1189:T31)
        n550 = call <vilib>:"Add State(s) to Queue__jki_lib_state_machine.vi"("State(s) in (\"\")"=w1187) -> ("States Out"=w1188:string)  [unwired: 14 in]
      }
      frame "Data: Queue" {
        # "Put Data in Queue to be used by parsing/saving code ->"
        n551 = Unbundle By Name(w1199) -> ("Q Element"=w1197:T19)
        n552 = Enqueue Element(queue=w1198, element=w1197) -> (queue out=w1202:refnum<queue>)  [unwired: 2 in, 2 out]
        n553 = Get Queue Status(queue=w1202) -> (# elements in queue=w1201:i32)  [unwired: 2 in, 7 out]
        "# elements in queue" <- w1201
        n554 = property on="# elements in queue" class="DigNum (strict)"("Val(Sgnl)"=w1201) -> ()  [unwired: 2 in, 2 out]
        n555 = call <vilib>:"Add State(s) to Queue__jki_lib_state_machine.vi"("State(s) in (\"\")"=w1205) -> ("States Out"=w1204:string)  [unwired: 14 in]
      }
    }
    n556 = local read "Debug Mode"() -> (w923:bool)
    n557 = case shown="True" w923 {
      tunnel: [w937 w940] -> w926
      tunnel: w925 -> [w937 w939]
      tunnel: w924 -> [_ w938]
      frame False {
      }
      frame True {
        n558 = Build Array (concatenate)(w939, w938) -> (w940:string[])
        "daq debug array" <- w940
      }
    }
  }
  n559 = while "Data Procressing, UI Update, Data Storage" {
    shift-right: [w1215] -> _
    shift-left: _ -> [w1214]
    shift-right: [w1217] -> _
    shift-left: _ -> [w1213]
    shift-right: [w1216] -> _
    shift-left: w4 -> [w1218]
    tunnel: w19 -> [w1212]
    shift-right: [w1210] -> _
    shift-left: string[] [] -> [w1211]
    tunnel: [w1206] -> w21
    stop <- w1206 stop-if-true
    n560 = call <vilib>:"Parse State Queue__jki_lib_state_machine.vi"("State Queue"=w1218, "Error In (no error)"=w1213) -> ("Remaining States"=w1220:string, "Current State"=w1209:string, "Arguments"=w1219:string)  [unwired: 11 in]
    n561 = case shown="\"Data: Process RMC\"" w1209 {
      selector: w1209 -> [_ w1282 _ _ _ _ _ _ _ _ _ _ _ _ _ _ _ _ _ _ _ _ _]
      tunnel: w1220 -> [w1231 w1286 w1298 w1302 w1310 w1316 w1324 w1341 w1358 w1383 w1425 w1496 w1531 w1558 w1572 w1663 w1690 w1720 w1762 w1768 w1828 w1870 w1890]
      tunnel: w1219 -> [_ _ _ _ _ w1312 _ _ _ _ _ _ _ _ _ _ _ _ _ _ _ _ _]
      tunnel: w1214 -> [w1229 w1284 w1295 w1299 w1307 w1311 w1321 w1338 w1355 w1378 w1419 w1494 w1525 w1555 w1566 w1658 w1687 w1717 w1759 w1765 w1786 w1849 w1886]
      tunnel: [w1228 w1288 errorcluster {"status"=FALSE, "code"=0, "source"=""} ("error out") w1300 w1308 w1314 w1322 w1339 w1356 w1381 w1423 w1463 w1521 w1556 w1570 w1661 w1688 w1718 w1760 w1766 w1826 w1859 w1888] -> w1217
      tunnel: w1213 -> [w1227 w1287 w1294 w1300 w1308 w1313 w1322 w1339 w1356 w1381 w1423 w1463 w1521 w1556 w1570 w1661 w1688 w1718 w1760 w1766 w1826 w1846 w1888]
      tunnel: [w1230 w1285 w1297 w1301 w1309 w1315 w1323 w1340 w1357 w1382 w1424 w1495 w1530 w1557 w1571 w1662 w1689 w1719 w1761 w1767 w1827 w1869 w1889] -> w1216
      tunnel: [_ _ _ _ _ _ _ _ _ _ _ _ _ _ _ _ _ _ _ _ _ _ TRUE] -> w1206
      tunnel: [w1226 w1284 w1295 w1299 w1307 w1311 w1321 w1337 w1354 w1377 w1419 w1493 w1524 w1555 w1569 w1659 w1687 w1717 w1759 w1765 w1785 w1849 w1886] -> w1215
      tunnel: "UI Timer" -> [w1225 _ _ _ _ _ _ _ _ _ _ _ _ _ _ _ _ _ _ _ _ _ _]
      tunnel: w1212 -> [_ _ _ _ _ _ _ w1336 w1353 _ _ _ _ _ _ _ _ _ _ _ _ _ _]
      frame "", "Idle" {
        # "executes when the state queue is empty"
        n562 = event shown="[2] \"End1_Main\": Value Change" {
          selector: _ -> [_ _ _ _ _]
          dyn-events: _ -> [_ _ _ _ _]
          timeout: w1225 -> [_ _ _ _ _]
          tunnel: w1231 -> [w1236 _ _ w1274 w1279]
          tunnel: [w1235 w1239 w1256 w1274 w1279] -> w1230
          tunnel: w1229 -> [w1233 w1240 w1245 w1275 w1280]
          tunnel: [w1234 w1237 w1254 w1276 w1281] -> w1228
          tunnel: w1227 -> [w1234 w1237 w1254 w1276 w1281]
          tunnel: [w1233 w1240 w1246 w1275 w1280] -> w1226
          event Timeout {
            n563 = event-data() -> ()  [unwired: 1 in, 1 out]
            n564 = call <vilib>:"Add State(s) to Queue__jki_lib_state_machine.vi"("State(s) in Front (\"\")"="UI: Update", "State(s) in (\"\")"=w1236) -> ("States Out"=w1235:string)  [unwired: 13 in]
          }
          event "# elements in queue": Value Change {
            n565 = event-data() -> ()  [unwired: 1 in, 6 out]
            n566 = call <vilib>:"Add State(s) to Queue__jki_lib_state_machine.vi"("State(s) in Front (\"\")"="Data: DeQueue\nData: Process\nData: Save\nUI: Update" ("State(s) in Front (\"\")")) -> ("States Out"=w1239:string)  [unwired: 14 in]
          }
          event "End1_Main": Value Change {
            n567 = event-data() -> ()  [unwired: 1 in, 6 out]
            n568 = Unbundle By Name(w1245) -> ("Q Element.Data"=w1243:string[][], "Q Element.Data Array"=w1251:dbl[], "Data Save Array"=w1244:string[][])
            n569 = local read "Write to File"() -> (w1247:bool)
            n570 = local read "Use Dry Gas Meter?"() -> (w1249:bool)
            n571 = Index Array(array=w1243, index (col)=0 ("disabled index (col)")) -> (element=w1241:string[])  [unwired: 1 in]
            n572 = Search 1D Array(1D array=w1241, element="Gas Feedback") -> (index of element=w1253:i32)  [unwired: 1 in]
            n573 = And(x=w1249, y=w1247) -> (x .and. y?=w1248:bool)
            n574 = Index Array(array=w1251, index=w1253) -> (element=w1250:dbl)
            n575 = case shown="True" w1248 {
              tunnel: w1250 -> [_ w1268]
              tunnel: [w1257 w1264] -> w1246
              tunnel: w1245 -> [w1257 w1263]
              tunnel: w1244 -> [_ w1261]
              frame False {
              }
              frame True {
                n576 = Number To Fractional String(number=w1268, precision (6)=i16 3) -> (F-format string=w1267:string)  [unwired: 2 in]
                n577 = Fract/Exp String To Number(string=w1267) -> (number=w1269:dbl)  [unwired: 3 in, 1 out]
                n578 = call "DPT Worksheet DOE Audit.vi"() -> ("DOE Data Out"=w1270:T25)  [unwired: 13 in, 2 out]
                n579 = Bundle By Name(cluster=w1270, "Gas Vol Fin"=w1269) -> (w1271:T25)
                n580 = Concatenate Strings("Dry Meter Final Reading", "," ("string"), w1267) -> (w1262:string)
                n581 = local read "2015?"() -> (w1265:bool)
                n582 = Build Array(w1262) -> (w1260:string[])
                n583 = call "DPT Worksheet DOE Audit.vi"("2015?"=w1265, "Add?"=TRUE, "DOE Data"=w1271) -> ()  [unwired: 10 in, 3 out]
                n584 = Build Array (concatenate)(w1261, w1260) -> (w1259:string[][])
                n585 = Bundle By Name(cluster=w1263, "Data Save Array"=w1259) -> (w1264:T33)
              }
            }
            n586 = call <vilib>:"Add State(s) to Queue__jki_lib_state_machine.vi"("State(s) in Front (\"\")"="Finalize Sequence\nExit" ("State(s) in Front (\"\")")) -> ("States Out"=w1256:string)  [unwired: 14 in]
          }
          event Value Change {
            n587 = event-data() -> ()  [unwired: 1 in, 6 out]
            n588 = local write "Tab Control"(T10."                                  Debug Info" ("Tab Control")) -> ()
          }
          event Value Change {
            n589 = event-data() -> ()  [unwired: 1 in, 6 out]
            n590 = local write "Tab Control"(T10."                           Data  " ("Tab Control")) -> ()
          }
        }
      }
      frame Default {
        w1291 = 42 items=["No error", "Argument error", "Memory is full", "Out of zone", "End of file", "File already open", "Generic file I/O error", "File not found", "File permission error", "Disk is full", "Duplicate path", "Too many files open", "System feature not enabled", "Resource file not found", "Cannot add resource", "Resource not found", "Image not found", "Image memory error", "Pen does not exist", "Config type invalid", "Config token not found", "Config parse error", "Config memory error", "Bad external code format", "Bad external code offset", "External code not present", "Null window", "Destroy window error", "Null menu", "Print aborted", "Bad print record", "Print driver error", "Windows error during printing", "Memory error during printing", "Print dialog error", "Generic print error", "Invalid device refnum", "Device not found", "Device parameter error", "Device unit error", "Cannot open device", "Device call aborted", "Generic error", "Cancelled by user", "Object ID too low", "Object ID too high", "Object not in heap", "Unknown heap", "Unknown object (invalid DefProc)", "Unknown object (DefProc not in table)", "Message out of range", "Invalid (null) method", "Unknown message", "Manager call not supported", "Bad address", "Network operation in progress", "Network operation timed out", "Connection is busy", "Network attribute not supported", "Network error", "Address in use", "System out of memory", "Connection aborted", "Connection refused", "Not connected", "Already connected", "Connection closed", "Initialization error (interapplication manager)", "Bad occurrence", "Wait on unbound occurrence handler", "Occurrence queue overflow", "Datalog type conflict", "Unused", "Unrecognized type (interapplication manager)", "Memory corrupt", "Failed to make temporary DLL", "Old CIN version", "Drag socket not found", "Failed to load drop-object", "Failed to register OLE object", "Failed to release OLE object", "Format specifier type mismatch", "Unknown format specifier", "Too few format specifiers", "Too many format specifiers", "Scan failed", "Newer CIN version", "Error converting to variant", "Runtime menu error", "Password tampered", "Variant attribute not found", "Incompatible variant data type", "Event data is not available", "Event Store is not present", "Occurrence is not found", "Event Queue is not created", "Event info is not available", "Refnum passed is NULL", "Error retrieving Class GUID", "Error retrieving CoClass GUID", "Error retrieving TypeLib GUID.", "Bad built application magic bytes.", "Specific driver is different from the specific driver associated with the Logical Name.", "There is no session opened to the class driver.", "Max Error", "MAX - Error with config objects", "MAX - Error loading configuration", "MAX - Group not supported"]
        # "Current State"
        # "Do not delete, rename, or modify this frame.\n(this is used to capture unhandled states and typos)"
        # "Handle mistyped state name (developer tool)"
        n591 = Format Into String(format string="Software Exception: Unhandled State \"%s\"." ("message"), error in=w1287, w1282) -> (resulting string=w1290:string, error out=w1289:errorcluster)  [unwired: 1 in]
        n592 = call <vilib>:"Error Cluster From Error Code.vi"("show call chain? (False)"=TRUE, "error in (no error)"=w1289, "error message (\"\")"=w1290, "error code (0)"=w1291) -> ("error out"=w1288:errorcluster)  [unwired: 5 in]
        n593 = call <vilib>:"Add State(s) to Queue__jki_lib_state_machine.vi"("State(s) in (\"\")"=w1286) -> ("States Out"=w1285:string)  [unwired: 14 in]
      }
      frame "Error Handler" {
        # "Unhandled Error -- Display it"
        # "Handle any errors here.\nYou can also output any states to clean-up after errors occur"
        # "Clear error"
        n594 = call <vilib>:"General Error Handler.vi"("error in (no error)"=w1294) -> ()  [unwired: 10 in, 5 out]
        n595 = call <vilib>:"Add State(s) to Queue__jki_lib_state_machine.vi"("State(s) in Front (\"\")"="/* Post Error States", "State(s) in (\"\")"=w1298) -> ("States Out"=w1297:string)  [unwired: 13 in]
      }
      frame "---------- UI ----------" {
        # "Do not put any code in this frame.\n(It is a separator no-op. You can make a copy of this frame to create a new Data frame)"
        n596 = call <vilib>:"Add State(s) to Queue__jki_lib_state_machine.vi"("State(s) in (\"\")"=w1302) -> ("States Out"=w1301:string)  [unwired: 14 in]
      }
      frame "UI: Update" {
        # "Update User Interface with processed Data"
        n597 = local read "Start Time (sec)"() -> (w1305:T13)
        n598 = call "String_in_Reference.vi"() -> ("String Out"=→"Status Message":string)  [unwired: 19 in]
        n599 = call "UTILITY E-Time.vi"() -> ("Elapsed Time (sec)"=w1304:dbl)  [unwired: 9 in, 2 out]
        n600 = Subtract(x=w1304, y=w1305) -> (x-y=→"Elapsed Time":T13)
        n601 = call <vilib>:"Add State(s) to Queue__jki_lib_state_machine.vi"("State(s) in (\"\")"=w1310) -> ("States Out"=w1309:string)  [unwired: 14 in]
      }
      frame "UI: Cursor Set" {
        # "Argument"
        # "Set and Unset Cursor Busy.\n(Usage: \"UI: Cursor Set >> Busy|Idle\")"
        n602 = case shown="\"Idle\", Default" w1312 {
          tunnel: w1313 -> [w1318 w1320]
          tunnel: [w1317 w1319] -> w1314
          frame "Idle", Default {
            n603 = call <vilib>:"Unset Busy.vi"("error in (no error)"=w1318) -> ("error out"=w1317:errorcluster)  [unwired: 10 in]
          }
          frame "Busy" {
            n604 = call <vilib>:"Set Busy.vi"("error in (no error)"=w1320) -> ("error out"=w1319:errorcluster)  [unwired: 9 in, 1 out]
          }
        }
        n605 = call <vilib>:"Add State(s) to Queue__jki_lib_state_machine.vi"("State(s) in (\"\")"=w1316) -> ("States Out"=w1315:string)  [unwired: 14 in]
      }
      frame "------ DATA ------" {
        # "Do not put any code in this frame.\n(It is a separator no-op. You can make a copy of this frame to create a new Data frame)"
        n606 = call <vilib>:"Add State(s) to Queue__jki_lib_state_machine.vi"("State(s) in (\"\")"=w1324) -> ("States Out"=w1323:string)  [unwired: 14 in]
      }
      frame "Data: Initialize" {
        w1329 = FALSE  # Power Previous
        w1330 = FALSE  # Enable RMC
        w1333 = dbl[] []  # Time Array
        w1332 = dbl[][] []  # Data Array
        w1331 = TRUE  # Init Save File
        w1334 = TRUE  # Graph Reset
        # "Next update\nmake this variable. It is currently\nthe default value"
        # "Offset value init."
        n607 = call "UTILITY FGV Double.vi"("Value In"=0.0, "Set?"=TRUE) -> ()  [unwired: 9 in, 1 out]
        n608 = local read "Q Element"() -> (w1335:T19)
        n609 = call <vilib>:"Add State(s) to Queue__jki_lib_state_machine.vi"("State(s) in (\"\")"=w1341) -> ("States Out"=w1340:string)  [unwired: 14 in]
        n610 = Bundle(cluster=w1338, "queue out"=w1336, "Q Element"=w1335, "Graph Reset"=w1334, "Init Save File"=w1331, "Time Array"=w1333, "Data Array"=w1332, "Enable RMC"=w1330, "Power Previous"=w1329, "Data Save Array"="Data Save Array", "Excel Template Path"="Excel Template Path") -> (w1337:T33)
      }
      frame "Data: DeQueue" {
        # "Remove Time"
        n611 = Dequeue Element(queue=w1353) -> (element=w1352:T19)  [unwired: 2 in, 3 out]
        n612 = Unbundle By Name(w1352) -> ("Data"=w1350:string[][], "Data Array"=w1345:dbl[])
        n613 = Number To Fractional String(number=w1345) -> (F-format string=w1351:string[])  [unwired: 3 in]
        n614 = local read "Plot Legend"() -> (w1347:T18)
        n615 = Build Array (concatenate)(w1350, w1351) -> (w1349:string[][])
        n616 = Delete From Array(array=w1345, length=1, index=0) -> (array with subset deleted=w1344:dbl[])  [unwired: 1 out]
        n617 = Transpose 2D Array(2D array=w1349) -> (transposed array=→"Data":string[][])
        n618 = for {
          tunnel: w1344 -> [w1360] mode=indexing
          tunnel: w1347 -> [w1361] mode=indexing
          tunnel: [w1359] -> w1346 mode=indexing
          n619 = Bundle By Name(cluster=w1361, "Value"=w1360) -> (w1359:T34)
        }
        n620 = local write "Plot Legend"(w1346) -> ()
        n621 = Bundle By Name(cluster=w1355, "Q Element"=w1352) -> (w1354:T33)
        n622 = call <vilib>:"Add State(s) to Queue__jki_lib_state_machine.vi"("State(s) in (\"\")"=w1358) -> ("States Out"=w1357:string)  [unwired: 14 in]
      }
      frame "Data: Process" {
        # "Disable RMC during power off."
        # "If the current indicates the the dryer is on, go to the Data: Process RMC"
        n623 = Unbundle By Name(w1378) -> ("Q Element.Data"=w1372:string[][], "Q Element.Data Array"=w1371:dbl[], "Enable RMC"=w1376:bool)
        n624 = local read "Power (Watts)"() -> (w1363:T12)
        n625 = local read "Write to File"() -> (w1366:bool)
        n626 = Greater?(x=w1363, y="Power On Threshold") -> (0:w1362:bool)
        "Power >Threshold" <- w1362
        n627 = And(x=w1362, y=w1366) -> (x .and. y?=w1367:bool)
        "Power ON" <- w1367
        n628 = call "DPT Dryer Power Latches.vi"("Time Limit in Seconds"="Power off Check RMC sec", "Power On"=w1367, "Init?"=FALSE) -> ("Time of Last Power On"=w1369:dbl, "Power Off One Shot"=w1365:bool, "Power On One Shot"=w1370:bool)  [unwired: 6 in]
        "Power On One Shot" <- w1370
        "Power Off One Shot" <- w1365
        n629 = Compound Arithmetic op=AND(w1370, invert w1365, w1366) -> (w1374:bool)
        n630 = Compound Arithmetic op=AND(w1374, invert w1376) -> (w1375:bool)
        n631 = case shown="True" w1375 {
          tunnel: w1372 -> [_ w1400]
          tunnel: w1371 -> [_ w1399]
          tunnel: string[] ["Wp:Sigma", "Tscale", "Gas Pressure", "Gas Temperature", "Barometric Pressure", "Gas Feedback"] ("Label List 2") -> [_ w1401]
          frame False {
          }
          frame True {
            # "First time through, init. start time."
            n632 = for {
              tunnel: w1399 -> [w1416]
              tunnel: w1400 -> [w1413]
              tunnel: w1401 -> [w1415] mode=indexing
              tunnel: [w1414] -> w1398 mode=indexing
              n633 = Index Array(array=w1413, index (col)=0 ("disabled index (col)")) -> (element=w1411:string[])  [unwired: 1 in]
              n634 = Search 1D Array(1D array=w1411, element=w1415) -> (index of element=w1417:i32)  [unwired: 1 in]
              n635 = Index Array(array=w1416, index=w1417) -> (element=w1414:dbl)
            }
            n636 = call "UTILITY E-Time.vi"() -> ("Elapsed Time (sec)"=w1402:dbl)  [unwired: 9 in, 2 out]
            "Start Time (sec)" <- w1402
            n637 = local read "Use Dry Gas Meter?"() -> (w1394:bool)
            n638 = Array To Cluster(array=w1398) -> (cluster=w1397:T35)
            n639 = Unbundle(w1397) -> ("[0]"=w1396:dbl, "[1]"=→"Init Scale Temp":dbl, "[2]"=w1387:dbl, "[3]"=w1389:dbl, "[4]"=w1391:dbl, "[5]"=w1392:dbl)
            n640 = case shown="False" w1394 {
              tunnel: [w1406 w1410] -> w1393
              tunnel: w1392 -> [_ w1410]
              tunnel: w1391 -> [_ w1409]
              tunnel: [w1406 w1409] -> w1390
              tunnel: w1389 -> [_ w1408]
              tunnel: [w1406 w1408] -> w1388
              tunnel: w1387 -> [_ w1407]
              tunnel: [w1406 w1407] -> w1386
              frame False {
                w1406 = 0.0 ("[2]")
              }
              frame True {
              }
            }
            n641 = local read "2015?"() -> (w1385:bool)
            n642 = call "DPT Worksheet DOE Audit.vi"() -> ("DOE Data Out"=w1404:T25)  [unwired: 13 in, 2 out]
            n643 = Bundle By Name(cluster=w1404, "Start Time(s)"=w1402, "Elect Energy Start"=w1396, "Gas Meter Pres"=w1386, "Gas Meter Temp"=w1388, "Barometer Pres"=w1390, "Gas Vol Init"=w1393) -> (w1403:T25)
            n644 = call "DPT Worksheet DOE Audit.vi"("2015?"=w1385, "Add?"=TRUE, "DOE Data"=w1403) -> ()  [unwired: 10 in, 3 out]
          }
        }
        n645 = case shown="True" w1365 {
          tunnel: w1369 -> [_ w1384]
          frame False {
          }
          frame True {
            "Tend?" <- w1384
          }
        }
        n646 = Bundle By Name(cluster=w1378, "Enable RMC"=w1374) -> (w1377:T33)
        n647 = call <vilib>:"Add State(s) to Queue__jki_lib_state_machine.vi"("State(s) in Front (\"\")"="Data: Process Gas\nData: Process RMC", "State(s) in (\"\")"=w1383) -> ("States Out"=w1382:string)  [unwired: 13 in]
      }
      frame "Data: Process Gas" {
        # "If the current indicates the the dryer is on, go to the Data: Process RMC"
        n648 = Unbundle By Name(w1419) -> ("Q Element.Data"=w1421:string[][], "Q Element.Data Array"=w1420:dbl[], "Power Previous"=w1418:bool)
        n649 = case shown="True" w1418 {
          tunnel: "Gas Pressure" ("Label") -> [_ w1437]
          tunnel: w1421 -> [_ w1428]
          tunnel: w1420 -> [_ w1435]
          frame False {
          }
          frame True {
            n650 = Index Array(array=w1428, index (col)=0 ("disabled index (col)")) -> (element=w1426:string[])  [unwired: 1 in]
            n651 = Search 1D Array(1D array=w1426, element=w1437) -> (index of element=w1436:i32)  [unwired: 1 in]
            n652 = Index Array(array=w1435, index=w1436) -> (element=w1434:dbl)
            n653 = call "DPT Worksheet DOE Audit.vi"() -> ("DOE Data Out"=w1432:T25)  [unwired: 13 in, 2 out]
            n654 = while {
              tunnel: w1434 -> [w1441]
              shift-right: [w1439] -> _
              shift-left: _ -> [w1440]
              tunnel: [w1438] -> w1430
              stop <- TRUE stop-if-true
              n655 = Build Array (concatenate)(w1440, w1441) -> (w1439:dbl[])
              n656 = call-poly <vilib>:"Mean.vi"("X"=w1439) -> ("mean"=w1438:dbl)  [unwired: 1 out]
            }
            n657 = Bundle By Name(cluster=w1432, "Gas Meter Pres"=w1430) -> (w1431:T25)
            n658 = local read "2015?"() -> (w1429:bool)
            n659 = call "DPT Worksheet DOE Audit.vi"("2015?"=w1429, "Add?"=TRUE, "DOE Data"=w1431) -> ()  [unwired: 10 in, 3 out]
          }
        }
        n660 = call <vilib>:"Add State(s) to Queue__jki_lib_state_machine.vi"("State(s) in (\"\")"=w1425) -> ("States Out"=w1424:string)  [unwired: 14 in]
      }
      frame "Data: Process RMC" {
        # "FIXME: RMC calculated after power on.  Is this OK?"
        # "Process Data Steps.\nPuts the gathered data into arrays to be saved."
        n661 = call "UTILITY Counter.vi"() -> ("Count"=→"Data Process RMC Counter":dbl)  [unwired: 11 in]
        n662 = Unbundle By Name(w1494) -> ("Graph Reset"=w1491:bool, "Q Element"=w1489:T19, "Enable RMC"=w1454:bool)
        n663 = call "UTILITY FGV Double.vi"() -> ("Value"=w1471:dbl)  [unwired: 11 in]
        n664 = local read "Offset"() -> (w1465:dbl)
        n665 = local read "Init Offset Coeff"() -> (w1464:dbl)
        n666 = Multiply(x=w1464, y=w1471) -> (x*y=w1470:dbl)
        n667 = Unbundle By Name(w1489) -> ("Data"=w1448:string[][], "Data Array"=w1446:dbl[])
        n668 = Add(x=w1465, y=w1470) -> (x+y=w1469:dbl)
        "Load Offset" <- w1469
        n669 = Or(x=w1491, y="Clear Graph") -> (x .or. y?=w1488:bool)
        n670 = case shown="True" w1488 {
          tunnel: [w1516 w1518] -> w1487
          tunnel: "Plot: Add Data All\nPlot: Add Data Power\nPlot: Add Data RMC" ("State(s) in Front (\"\")") -> [w1517 w1518]
          frame True {
            n671 = Concatenate Strings("Plot: Init", "\r", w1517) -> (w1516:string)
          }
          frame False {
          }
        }
        n672 = Select(t=w1469, s="Apply Load Offset", f=0.0) -> (s? t:f=w1468:dbl)
        n673 = for {
          tunnel: w1448 -> [w1509]
          tunnel: string[] ["Scale Weight", "Room Ambient(F)", "RDB F", "Tscale"] -> [w1513] mode=indexing
          tunnel: w1446 -> [w1512]
          tunnel: [w1510] -> w1484 mode=indexing
          n674 = Index Array(array=w1509, index (col)=0 ("disabled index (col)")) -> (element=w1508:string[])  [unwired: 1 in]
          n675 = Search 1D Array(1D array=w1508, element=w1513) -> (index of element=w1511:i32)  [unwired: 1 in]
          n676 = Index Array(array=w1512, index=w1511) -> (element=w1510:dbl)
        }
        n677 = local read "Init Scale Temp"() -> (w1474:dbl)
        n678 = local read "Bone Dry Weight (lbs)"() -> (w1451:T12)
        n679 = local read "Wet Clothing Weight (lbs)"() -> (w1457:T12)
        n680 = local read "Empty Dryer Cold Weight (lbs)"() -> (w1458:T12)
        n681 = Array To Cluster(array=w1484) -> (cluster=w1483:T36)
        n682 = Unbundle(w1483) -> ("[0]"=w1449:dbl, "[1]"=w1461:dbl, "[2]"=w1460:dbl, "[3]"=w1477:dbl)
        "Scale Weight (lbs)" <- w1449
        "Room Ambient (Degrees F)" <- w1461
        "RDB Temperature (Degrees F)" <- w1460
        n683 = Bundle(cluster=T16 {"Measeured Weight"=0.0, "BDW - Bone Dry Wt(lbs)"=0.0, "Empty Dryer Cold Weight"=0.0, "Measured IMC"=0.0, "Tamb"=0.0, "T-RDB"=0.0, "Drum Volume"=0.0, "Load Offset"=0.0, "Temp Coeff"=0.0, "Temp Cal"=0.0, "Tscale"=0.0} ("RMC Calc Inputs 2"), "Measeured Weight"=w1449, "BDW - Bone Dry Wt(lbs)"=w1451, "Empty Dryer Cold Weight"=w1458, "Measured IMC"=w1457, "Tamb"=w1461, "T-RDB"=w1460, "Drum Volume"="Drum Volume", "Load Offset"=w1468, "Temp Coeff"="Scale Temp Coeff", "Temp Cal"=w1474, "Tscale"=w1477) -> (w1481:T16)
        "RMC Calc Inputs" <- w1481
        n684 = local read "Power On One Shot"() -> (w1476:bool)
        n685 = case shown="True" w1476 {
          tunnel: w1481 -> [_ w1506]
          tunnel: [w1497 w1505] -> w1453
          tunnel: "MA Filter Size" -> [_ w1504]
          tunnel: [_ w1503] -> w1478
          tunnel: [w1497 w1502] -> w1450
          tunnel: [_ w1501] -> w1456
          tunnel: [_ w1500] -> w1475
          tunnel: w1454 -> [_ w1499]
          tunnel: [w1497 w1498] -> w1473
          frame False {
            w1497 = 0.0 ("RMC")
          }
          frame True {
            n686 = call "DPT MA Scale Corrections.vi"("RMC Calc Inputs"=w1506, "Enable"=w1499, "MA Filter Size"=w1504) -> ("RMC_Sm"=w1498:dbl, "RMC"=w1505:dbl, "Raw Weight"=w1503:dbl, "Corrected Weight"=w1501:dbl, "Wcomp"=w1502:dbl, "Wbouy"=w1500:dbl)  [unwired: 11 in]
          }
        }
        "Wbouy" <- w1475
        "Cloth Weight Estimate (lbs)" <- w1456
        n687 = local read "Use Smoothing"() -> (w1472:bool)
        n688 = call <vilib>:"Add State(s) to Queue__jki_lib_state_machine.vi"("State(s) in Front (\"\")"=w1487, "State(s) in (\"\")"=w1496) -> ("States Out"=w1495:string)  [unwired: 13 in]
        n689 = Select(t=w1473, s=w1472, f=w1453) -> (s? t:f=w1462:dbl)
        n690 = Build Array(w1473, w1453, w1478, w1456, w1450, w1475) -> (w1445:dbl[])
        n691 = call "DPT Sort Data in Columns.vi"("Q Element.Data"=w1448, "DAQ Label List 2"=string[] ["Smooth Rmc", "RMC", "Raw Weight", "Corrected Weight", "Wcomp", "Wbuoy"], "Old Data Array"=w1446, "cDAQ Data Out"=w1445) -> ("Output Data"=w1443:string[][], "New Data Array"=w1444:dbl[])  [unwired: 4 in, 1 out]
        n692 = Absolute Value(x=w1462) -> (abs(x)=→"Relative Moisture Content (%)" →"RMC Chart":dbl)
        n693 = Bundle By Name(cluster=w1494, "Graph Reset"=FALSE, "Q Element.Data"=w1443, "Q Element.Data Array"=w1444) -> (w1493:T33)
      }
      frame "Data: Save" {
        n694 = Unbundle By Name(w1525) -> ("Data Save Array"=w1520:string[][], "Q Element.Date"=w1522:string, "Init Save File"=w1528:bool, "Q Element.Data"=w1526:string[][], "Q Element.Data Array"=w1527:dbl[])  [unwired: 1 out]
        n695 = local read "Write to File"() -> (w1529:bool)
        n696 = case shown="True" w1529 {
          tunnel: w1528 -> [w1533 w1542]
          tunnel: w1527 -> [_ w1541]
          tunnel: w1526 -> [_ w1540]
          tunnel: [w1533 FALSE ("Init Save File")] -> w1523
          tunnel: w1522 -> [_ w1537]
          tunnel: w1520 -> [_ w1535]
          tunnel: [string[][] [] w1534] -> w1519
          frame False {
            # "Don't write to file. Therefore just put a constant\nas a place holder"
          }
          frame True {
            n697 = Build Array("Date" ("delimiter (\\t)"), w1537) -> (w1536:string[])
            n698 = case shown="False" w1542 {
              tunnel: w1541 -> [w1550 w1554]
              tunnel: w1540 -> [w1548 _]
              tunnel: w1536 -> [w1546 _]
              tunnel: [w1543 w1551] -> w1534
              tunnel: w1535 -> [w1545 w1553]
              frame True {
                # "Add a header"
                n699 = Number To Fractional String(number=w1550) -> (F-format string=w1549:string[])  [unwired: 3 in]
                n700 = Build Array (concatenate)(w1548, w1549) -> (w1547:string[][])
                n701 = Build Array (concatenate)(w1546, w1547) -> (w1544:string[][])
                n702 = Build Array (concatenate)(w1545, w1544) -> (w1543:string[][])
              }
              frame False {
                # "Save data to array"
                n703 = Number To Fractional String(number=w1554) -> (F-format string=w1552:string[])  [unwired: 3 in]
                n704 = Build Array (concatenate)(w1553, w1552) -> (w1551:string[][])
              }
            }
          }
        }
        n705 = call <vilib>:"Add State(s) to Queue__jki_lib_state_machine.vi"("State(s) in (\"\")"=w1531) -> ("States Out"=w1530:string)  [unwired: 14 in]
        n706 = Bundle By Name(cluster=w1525, "Init Save File"=w1523, "Data Save Array"=w1519) -> (w1524:T33)
      }
      frame "------PLOT-------" {
        # "Do not put any code in this frame.\n(It is a separator no-op. You can make a copy of this frame to create a new Data frame)"
        n707 = call <vilib>:"Add State(s) to Queue__jki_lib_state_machine.vi"("State(s) in (\"\")"=w1558) -> ("States Out"=w1557:string)  [unwired: 14 in]
      }
      frame "Plot: Init" {
        w1562 = cluster{dbl[], dbl[]}[] [] ("RHS Tank TCs")
        w1567 = TRUE  # Init Save File
        w1568 = FALSE  # Graph Reset
        # "Remove Time"
        n708 = Unbundle By Name(w1566) -> ("Q Element.Data"=w1561:string[][])
        n709 = Index Array(array=w1561, index (col)=0 ("disabled index (col)")) -> (element=w1559:string[])  [unwired: 1 in]
        n710 = Delete From Array(array=w1559, length=1, index=0) -> (array with subset deleted=w1565:string[])  [unwired: 1 out]
        n711 = stacked-sequence {
          tunnel: w1565 -> [w1586 _ _]
          frame #0 {
            n712 = local read "Plot Legend"() -> (w1575:T18)
            n713 = Array Size(array=w1586) -> (size(s)=w1585:i32)
            n714 = local read "Number of TCs"() -> (w1584:i32)
            n715 = Index Array(array=w1575, index=0) -> (element=w1574:T34)
            n716 = To Unsigned Long Integer(number=w1585) -> (unsigned 32bit integer=w1587:u32)
            n717 = for {
              tunnel: w1586 -> [w1591] mode=indexing
              tunnel: w1584 -> [w1597]
              tunnel: w1574 -> [w1593]
              tunnel: [w1592] -> w1573 mode=indexing
              i -> [w1598]
              n718 = To Unsigned Long Integer(number=w1598) -> (unsigned 32bit integer=w1599:u32)
              n719 = Less?(x=w1598, y=w1597) -> (x < y?=w1595:bool)
              n720 = Boolean To (0,1)(Boolean=w1595) -> (0, 1=w1596:i16)
              n721 = property on="Plot All" class="XYGraph (strict)"("Active Plot"=w1599, "Plot.Plot Name"=w1591, "Plot.YScaleIdx"=w1596) -> ("Plot.Plot Color"=w1590:u32)  [unwired: 2 in, 2 out]
              n722 = Bundle By Name(cluster=w1593, "OnOff"=TRUE ("Boolean"), "Color Box"=w1590, "Title"=w1591) -> (w1592:T34)
            }
            n723 = property on="Plot All" class="XYGraph (strict)"("XScale.NameLbl.Text"="Time" ("X Scale.Name Label.Text"), "ActYScl"=1 ("Active Y Scale"), "YScale.NameLbl.Text"="Temperature °F" ("X Scale Label"), "YScale.Minimum"=50.0 ("Y Scale.Range:Minimum"), "YScale.Maximum"=200.0 ("Y Scale.Range:Maximum"), "ActYScl"=0 ("Active Y Scale"), "YScale.NameLbl.Text"="kWatts, lbs.,V,A" ("Y Scale Label Right"), "YScale.Minimum"=0.0 ("Ymin Right"), "YScale.Maximum"=250.0 ("Y Scale.Range:Maximum"), "LegNumRows"=w1587) -> ()  [unwired: 2 in, 2 out]
            n724 = local write "Plot Legend"(w1573) -> ()
          }
          frame #1 {
            w1611 = string[] ["Irms:Element 1", "Irms:Element 2", "P:Sigma"]
            n725 = control-ref of="Plot Power"() -> (w1603:refnum<vi>)
            n726 = for {
              tunnel: w1611 -> [w1620] mode=indexing
              tunnel: 2 ("y") -> [w1614]
              tunnel: w1603 -> [w1615]
              i -> [w1618]
              n727 = Greater Or Equal?(x=w1618, y=w1614) -> (x >= y?=w1616:bool)
              n728 = To Unsigned Long Integer(number=w1618) -> (unsigned 32bit integer=w1619:u32)
              n729 = Boolean To (0,1)(Boolean=w1616) -> (0, 1=w1617:i16)
              n730 = property on="Property Node" class="XYGraph (strict)"(reference=w1615, "Active Plot"=w1619, "Plot.Plot Name"=w1620, "Plot.YScaleIdx"=w1617) -> ()  [unwired: 1 in, 2 out]
            }
            n731 = Array Size(array=w1611) -> (size(s)=w1613:i32)
            n732 = To Unsigned Long Integer(number=w1613) -> (unsigned 32bit integer=w1602:u32)
            n733 = property on="Property Node" class="XYGraph (strict)"(reference=w1603, "XScale.NameLbl.Text"="Time" ("X Scale.Name Label.Text"), "ActYScl"=1 ("Active Y Scale"), "YScale.NameLbl.Text"="Watts" ("Y Scale.Name Label.Text"), "YScale.Minimum"=0.0 ("Y Scale.Range:Minimum"), "YScale.Maximum"=5000.0 ("Y Scale.Range:Maximum"), "ActYScl"=0 ("Active Y Scale"), "YScale.NameLbl.Text"="Current(Amps)" ("Y Scale.Name Label.Text"), "YScale.Minimum"=0.0 ("Y Scale.Range:Minimum"), "YScale.Maximum"=32.0 ("Y Scale.Range:Maximum"), "LegNumRows"=w1602) -> ()  [unwired: 1 in, 2 out]
          }
          frame #2 {
            w1628 = string[] ["RAW Weight", "RMC"]
            n734 = control-ref of="Plot RMC"() -> (w1621:refnum<vi>)
            n735 = Array Size(array=w1628) -> (size(s)=w1631:i32)
            n736 = To Unsigned Long Integer(number=w1631) -> (unsigned 32bit integer=w1629:u32)
            n737 = for {
              tunnel: w1628 -> [w1638] mode=indexing
              tunnel: w1621 -> [w1634]
              i -> [w1633]
              n738 = Equal To 0?(x=w1633) -> (x = 0?=w1635:bool)
              n739 = To Unsigned Long Integer(number=w1633) -> (unsigned 32bit integer=w1637:u32)
              n740 = Boolean To (0,1)(Boolean=w1635) -> (0, 1=w1636:i16)
              n741 = property on="Property Node" class="XYGraph (strict)"(reference=w1634, "Active Plot"=w1637, "Plot.Plot Name"=w1638, "Plot.YScaleIdx"=w1636) -> ()  [unwired: 1 in, 2 out]
            }
            n742 = property on="Property Node" class="XYGraph (strict)"(reference=w1621, "XScale.NameLbl.Text"="Time" ("X Scale.Name Label.Text"), "ActYScl"=1 ("Active Y Scale"), "YScale.NameLbl.Text"="LBS" ("Y Scale.Name Label.Text"), "AutoscaleDelay"=sgl 0.0 ("Autoscale Delay"), "ActYScl"=0 ("Active Y Scale"), "YScale.NameLbl.Text"="RMC" ("Y Scale.Name Label.Text"), "YScale.Minimum"=0.0 ("Y Scale.Range:Minimum"), "YScale.Maximum"=100.0 ("Y Scale.Range:Maximum"), "LegNumRows"=w1629) -> ()  [unwired: 1 in, 2 out]
          }
        }
        n743 = Bundle By Name(cluster=w1566, "Graph Reset"=w1568, "Init Save File"=w1567) -> (w1569:T33)
        n744 = local write "Plot All"(w1562) -> ()
        n745 = local write "Plot Power"(w1562) -> ()
        n746 = local write "Plot RMC"(w1562) -> ()
        n747 = call <vilib>:"Add State(s) to Queue__jki_lib_state_machine.vi"("State(s) in (\"\")"=w1572) -> ("States Out"=w1571:string)  [unwired: 14 in]
      }
      frame "Plot: Add Data All" {
        # "Add Current Sample to Data Array"
        # "First Element Assumed to be Time."
        n748 = Unbundle By Name(w1658) -> ("Time Array"=w1657:dbl[], "Q Element.Data Array"=w1652:dbl[], "Data Array"=w1660:dbl[][])
        n749 = case shown="True" "None" {
          selector: "None" -> [w1672 _]
          tunnel: "Plot Legend" -> [w1673 w1676]
          tunnel: [w1673 w1675] -> w1643
          tunnel: [w1672 w1674] -> w1640
          frame False {
          }
          frame True {
            n750 = for {
              tunnel: w1676 -> [w1679] mode=indexing
              tunnel: [w1678] -> w1675 mode=indexing
              tunnel: [w1677] -> w1674
              w1677 = FALSE ("OnOff")
              n751 = Bundle By Name(cluster=w1679, "OnOff"=w1677) -> (w1678:T34)
            }
          }
        }
        n752 = local write "None"(w1640) -> ()
        n753 = case shown="True" "All" {
          tunnel: w1643 -> [w1665 w1668]
          tunnel: [w1665 w1667] -> w1641
          tunnel: [FALSE ("OnOff") FALSE ("OnOff")] -> w1639
          frame False {
          }
          frame True {
            n754 = for {
              tunnel: w1668 -> [w1671] mode=indexing
              tunnel: [w1670] -> w1667 mode=indexing
              n755 = Bundle By Name(cluster=w1671, "OnOff"=TRUE) -> (w1670:T34)
            }
          }
        }
        n756 = Delete From Array(array=w1652, length=1, index=0) -> (deleted portion=w1650:dbl[], array with subset deleted=w1651:dbl[])
        n757 = Transpose 2D Array(2D array=w1660) -> (transposed array=w1655:dbl[][])
        n758 = Build Array (concatenate)(w1657, w1650) -> (w1653:dbl[])
        n759 = Build Array (concatenate)(w1655, w1651) -> (w1656:dbl[][])
        n760 = Transpose 2D Array(2D array=w1656) -> (transposed array=w1654:dbl[][])
        n761 = control-ref of="Plot All"() -> (w1646:refnum<vi>)
        n762 = local write "Plot Legend"(w1641) -> ()
        n763 = local write "All"(w1639) -> ()
        n764 = for {
          tunnel: w1653 -> [w1686]
          tunnel: [w1685] -> w1647 mode=indexing
          tunnel: w1654 -> [w1684] mode=indexing
          tunnel: w1646 -> [w1683]
          tunnel: w1641 -> [w1681] mode=indexing
          i -> [w1682]
          n765 = Unbundle By Name(w1681) -> ("OnOff"=w1680:bool)
          n766 = Bundle(w1686, w1684) -> (w1685:cluster{dbl[], dbl[]})  [unwired: 1 out]
          n767 = property on="Property Node" class="XYGraph (strict)"(reference=w1683, "Active Plot"=w1682, "Plot.Visible?"=w1680) -> ()  [unwired: 1 in, 2 out]
        }
        "Plot All" <- w1647
        n768 = call <vilib>:"Add State(s) to Queue__jki_lib_state_machine.vi"("State(s) in (\"\")"=w1663) -> ("States Out"=w1662:string)  [unwired: 14 in]
        n769 = Bundle By Name(cluster=w1658, "Time Array"=w1653, "Data Array"=w1654) -> (w1659:T33)
      }
      frame "Plot: Add Data Power" {
        n770 = disable-structure shown="Disabled" {
          disable-tunnel: w1687 -> [w1708 _]
          frame Disabled {
            n771 = Unbundle By Name(w1708) -> ("Q Element.Data"=w1707:string[][], "Time Array"=w1709:dbl[], "Data Array"=w1699:dbl[][])
            n772 = for {
              tunnel: w1707 -> [w1713]
              tunnel: string[] ["Irms:Element 1", "Irms:Element 2", "P:Sigma"] -> [w1712] mode=indexing
              tunnel: [w1711] -> w1706 mode=indexing
              n773 = Search 1D Array(1D array=w1713, element=w1712) -> (index of element=w1711:i32)  [unwired: 1 in]
            }
            n774 = Index Array(array=w1706, index #1=0 ("index"), index #2=1 ("index"), index #3=2 ("index")) -> (element #1=w1702:i32, element #2=w1701:i32, element #3=w1700:i32)
            n775 = Decrement(x=w1701) -> (x-1=w1692:i32)
            n776 = Decrement(x=w1702) -> (x-1=w1693:i32)
            n777 = Decrement(x=w1700) -> (x-1=w1691:i32)
            n778 = Index Array(array=w1699, index (row)=w1693) -> (element=w1698:dbl[])  [unwired: 1 in]
            n779 = Index Array(array=w1699, index (row)=w1692) -> (element=w1697:dbl[])  [unwired: 1 in]
            n780 = Index Array(array=w1699, index (row)=w1691) -> (element=w1696:dbl[])  [unwired: 1 in]
            n781 = Build Array(w1698, w1697, w1696) -> (w1695:dbl[][])
            n782 = for {
              tunnel: w1709 -> [w1716]
              tunnel: [w1715] -> w1710 mode=indexing
              tunnel: w1695 -> [w1714] mode=indexing
              n783 = Bundle("Time Array"=w1716, w1714) -> (w1715:cluster{"Time Array":dbl[], dbl[]})  [unwired: 1 out]
            }
            "Plot Power" <- w1710
          }
          frame Enabled {
          }
        }
        n784 = call <vilib>:"Add State(s) to Queue__jki_lib_state_machine.vi"("State(s) in (\"\")"=w1690) -> ("States Out"=w1689:string)  [unwired: 14 in]
      }
      frame "Plot: Add Data RMC" {
        # "I have disabled this case . I am doing a easier plot"
        n785 = disable-structure shown="Disabled" {
          disable-tunnel: w1717 -> [w1751 _]
          frame Disabled {
            # "Is the dry time and exponential?"
            n786 = local read "Debug Mode"() -> (w1731:bool)
            n787 = Unbundle By Name(w1751) -> ("Q Element.Data"=w1750:string[][], "Time Array"=w1740:dbl[], "Data Array"=w1723:dbl[][])
            n788 = Select(t="RMC", s=w1731, f="Smooth_Rmc") -> (s? t:f=w1728:string)
            n789 = Build Array("Weight", w1728) -> (w1727:string[])
            n790 = local read "Wet Clothing Weight (lbs)"() -> (w1721:T12)
            n791 = for {
              tunnel: w1750 -> [w1755]
              tunnel: w1727 -> [w1754] mode=indexing
              tunnel: [w1753] -> w1749 mode=indexing
              n792 = Search 1D Array(1D array=w1755, element=w1754) -> (index of element=w1753:i32)  [unwired: 1 in]
            }
            n793 = local read "Bone Dry Weight (lbs)"() -> (w1722:T12)
            n794 = local read "RMC Limit"() -> (w1739:dbl)
            n795 = Index Array(array=w1749, index #1=0 ("index"), index #2=1 ("index"), index #3=2 ("index")) -> (element #1=w1746:i32, element #2=w1745:i32, element #3=w1725:i32)
            n796 = Decrement(x=w1745) -> (x-1=w1741:i32)
            n797 = Decrement(x=w1746) -> (x-1=w1742:i32)
            n798 = Decrement(x=w1725) -> (x-1=w1724:i32)
            n799 = Index Array(array=w1723, index (row)=w1742) -> (element=w1734:dbl[])  [unwired: 1 in]
            n800 = Index Array(array=w1723, index (row)=w1741) -> (element=w1744:dbl[])  [unwired: 1 in]
            n801 = Divide(x=w1739, y=100.0) -> (x/y=w1737:dbl)
            n802 = Index Array(array=w1723, index (row)=w1724) -> ()  [unwired: 1 in, 1 out]
            n803 = Multiply(x=w1722, y=w1737) -> (x*y=w1736:T12)
            n804 = Build Array(w1734, w1744) -> (w1743:dbl[][])
            n805 = Add(x=w1722, y=w1736) -> (x+y=w1735:T12)
            n806 = for {
              tunnel: w1740 -> [w1758]
              tunnel: [w1757] -> w1752 mode=indexing
              tunnel: w1743 -> [w1756] mode=indexing
              n807 = Bundle("Time Array"=w1758, w1756) -> (w1757:cluster{"Time Array":dbl[], dbl[]})  [unwired: 1 out]
            }
            "Plot RMC" <- w1752
            n808 = call "DPT Estimate Completion Time.vi"("IMC Weight"=w1721, "Completion Weight"=w1735, "Time Values"=w1740, "Weight Values"=w1734) -> ("Completion Time Estimate"=→"Experimental Completion Time Estimate":dbl)  [unwired: 9 in, 2 out]
          }
          frame Enabled {
          }
        }
        n809 = call <vilib>:"Add State(s) to Queue__jki_lib_state_machine.vi"("State(s) in (\"\")"=w1720) -> ("States Out"=w1719:string)  [unwired: 14 in]
      }
      frame "-------FINALIZE------ " {
        n810 = call <vilib>:"Add State(s) to Queue__jki_lib_state_machine.vi"("State(s) in (\"\")"=w1762) -> ("States Out"=w1761:string)  [unwired: 14 in]
      }
      frame "Finalize Sequence" {
        n811 = local read "Write to File"() -> (w1763:bool)
        n812 = case shown="True" w1763 {
          tunnel: ["" "Finalize DataLog\nFinalize Write DOE Data" ("State(s) in Front (\"\")")] -> w1764
          frame False {
          }
          frame True {
          }
        }
        n813 = call <vilib>:"Add State(s) to Queue__jki_lib_state_machine.vi"("State(s) in Front (\"\")"=w1764, "State(s) in (\"\")"=w1768) -> ("States Out"=w1767:string)  [unwired: 13 in]
      }
      frame "Finalize DataLog" {
        w1790 = 60.0  # s/min
        # "RMC OK?"
        n814 = Unbundle By Name(w1786) -> ("Q Element.Data"=w1803:string[][], "Q Element.Data Array"=w1804:dbl[], "Data Save Array"=w1784:string[][])  [unwired: 1 out]
        n815 = flat-sequence {
          tunnel: [w1830] -> w1771
          tunnel: [w1832] -> w1824
          tunnel: w1771 -> [w1832]
          tunnel: [w1831] -> w1793
          frame #0 {
            n816 = local read "Scale Com Port"() -> (w1829:refnum<visa-resource-name>)
            n817 = call "DPT Panel Scale Reading Percision.vi"("VISA resource name"=w1829) -> ("read buffer"=w1830:T2)  [unwired: 13 in, 1 out]
          }
          frame #1 {
            n818 = call "UTILITY E-Time.vi"() -> ("Elapsed Time (sec)"=w1831:dbl)  [unwired: 9 in, 2 out]
          }
        }
        n819 = Build Array("Stopped" ("String")) -> (w1782:string[])
        n820 = for {
          tunnel: w1803 -> [w1835]
          tunnel: string[] ["Time", "Gas Feedback", "Wp:Sigma"] -> [w1839] mode=indexing
          tunnel: w1804 -> [w1838]
          tunnel: [w1836] -> w1805 mode=indexing
          n821 = Index Array(array=w1835, index (col)=0 ("disabled index (col)")) -> (element=w1833:string[])  [unwired: 1 in]
          n822 = Search 1D Array(1D array=w1833, element=w1839) -> (index of element=w1837:i32)  [unwired: 1 in]
          n823 = Index Array(array=w1838, index=w1837) -> (element=w1836:dbl)
        }
        n824 = local read "Enable RMC Limit"() -> (w1794:bool)
        n825 = local read "Power On One Shot"() -> (w1814:bool)
        n826 = Concatenate Strings("Final Weight:, " ("String"), w1824) -> (w1781:string)
        n827 = Build Array(w1781) -> (w1780:string[])
        n828 = Fract/Exp String To Number(string=w1824) -> (number=w1807:dbl)  [unwired: 3 in, 1 out]
        n829 = local read "Use Dry Gas Meter?"() -> (w1800:bool)
        n830 = Array To Cluster(array=w1805) -> (cluster=w1806:cluster{"[0]":dbl, "[1]":dbl, "[2]":dbl})
        n831 = Unbundle(w1806) -> ("[0]"=w1792:dbl, "[1]"=w1797:dbl, "[2]"=w1796:dbl)
        n832 = Subtract(x=w1793, y=w1792) -> (x-y=w1791:dbl)
        n833 = Divide(x=w1791, y=w1790) -> (x/y=w1789:dbl)
        n834 = Number To Fractional String(number=w1789) -> (F-format string=w1788:string)  [unwired: 3 in]
        n835 = And(x=w1794, y=w1814) -> (x .and. y?=w1815:bool)
        n836 = case shown="True" w1815 {
          tunnel: [TRUE w1842] -> w1813
          frame False {
          }
          frame True {
            n837 = local read "RMC Limit"() -> (w1843:dbl)
            n838 = local read "Relative Moisture Content (%)"() -> (w1841:T12)
            n839 = Greater?(x=w1843, y=w1841) -> (0:w1842:bool)
          }
        }
        n840 = Concatenate Strings("FMC DELAY (min):," ("String"), w1788) -> (w1778:string)
        n841 = Build Array(w1778) -> (w1779:string[])
        n842 = Select(t=w1797, s=w1800, f=0.0) -> (s? t:f=w1799:dbl)
        n843 = local read "Bone Dry Weight (lbs)"() -> (w1772:T12)
        n844 = local read "End Msg"() -> (w1777:string)
        n845 = Build Array(w1777) -> (w1776:string[])
        n846 = call "DPT Worksheet DOE Audit.vi"() -> ("DOE Data Out"=w1809:T25)  [unwired: 13 in, 2 out]
        n847 = Bundle By Name(cluster=w1809, "End Time(s)"=w1792, "Final Wt"=w1807, "Gas Vol Fin"=w1799, "Elect Energy End"=w1796) -> (w1808:T25)
        n848 = Divide(x=w1807, y=w1772) -> (x/y=w1823:T12)
        n849 = local read "2015?"() -> (w1787:bool)
        n850 = Decrement(x=w1823) -> (x-1=w1820:T12)
        n851 = Search and Replace String(replace all?=TRUE ("replace all? (F)"), input string=w1777, search string=",") -> (result string=w1816:string)  [unwired: 5 in, 3 out]
        n852 = Number To Fractional String(number=w1820) -> (F-format string=w1822:string)  [unwired: 3 in]
        n853 = call "DPT Worksheet DOE Audit.vi"("2015?"=w1787, "Add?"=TRUE, "DOE Data"=w1808) -> ()  [unwired: 10 in, 3 out]
        n854 = Concatenate Strings(w1816, "\r", "Final RMC:" ("String"), w1822) -> (w1812:string)
        n855 = call <vilib>:"Add State(s) to Queue__jki_lib_state_machine.vi"("State(s) in (\"\")"=w1828) -> ("States Out"=w1827:string)  [unwired: 14 in]
        n856 = Append True/False String(1:w1813, 2:". RMC Limit Not Reached." ("false string"), 3:"" ("true string"), 4:w1812) -> (0:w1775:string)
        "Final User Message" <- w1775
        n857 = Build Array(w1775) -> (w1774:string[])
        n858 = Build Array (concatenate)(w1784, w1782, w1780, w1779, w1776, w1774) -> (w1773:string[][])
        n859 = Bundle By Name(cluster=w1786, "Data Save Array"=w1773) -> (w1785:T33)
      }
      frame "Finalize Write DOE Data" {
        # "Create the directorys"
        # "This is the final parser"
        # "This is the Off Mode Data"
        # "This is the Raw Output Voltage data from the CDAQ"
        # "This is the full Dryer Test Data"
        n860 = disable-structure shown="Disabled" {
          frame Disabled {
            # "Analog voltage data in cluster"
            n861 = local read item#-1() -> (w1872)
            n862 = local read item#-1() -> (w1871)
            n863 = Build Array (concatenate)(w1872, w1871) -> ()  [unwired: 1 out]
          }
          frame Enabled {
          }
        }
        n864 = Unbundle By Name(w1849) -> ("Data Save Array"=w1854:string[][])
        n865 = local read "FileInit Cluster"() -> (w1856:T6)
        n866 = call <vilib>:"Three Button Dialog.vi"("Allow user to close window? (TRUE)"=FALSE, "Right Button Text (\"Cancel\")"="Lab Eval" ("Right Button Text (\"Cancel\")"), "Center Button Text (\"No\")"="Fail" ("F button name (\"Cancel\")"), "Left Button Text (\"Yes\")"="Pass" ("T button name (\"OK\")"), "message"="The final results are all placed under the same\n TR directory. The below buttons specifiy the directory") -> ("Which Button?"=w1861:T37)  [unwired: 6 in]
        n867 = local read "Off Mode Power Output"() -> (w1855:string[][])
        n868 = case shown="\"Center Button\"" w1861 {
          tunnel: ["Result: Pass" ("T button name (\"OK\")") w1878 w1883] -> _
          tunnel: [TRUE FALSE FALSE] -> _
          tunnel: ["Pass" ("T button name (\"OK\")") "Fail" "Lab Eval"] -> w1847
          frame "Left Button", Default {
          }
          frame "Center Button" {
            n869 = call "Prompt User for Input"() -> ("Reason for Failure"=w1879:string)  [unwired: 17 in, 2 out]
            n870 = Concatenate Strings("Result: Fail - ", w1879) -> (w1878:string)
          }
          frame "Right Button" {
            n871 = call "Prompt User for Input2"() -> ("Eval Description"=w1884:string)  [unwired: 17 in, 2 out]
            n872 = Concatenate Strings("Result:  Eval -", w1884) -> (w1883:string)
          }
        }
        n873 = disable-structure shown="Disabled" {
          frame Disabled {
            n874 = call "DPT Parser Dryer Performance.vi"() -> ()  [unwired: 10 in, 2 out]
          }
          frame Enabled {
          }
        }
        n875 = Unbundle By Name(w1856) -> ("TR Number"=w1858:string, "Lab ID"=w1857:string)
        n876 = Bundle By Name(cluster=w1856, "Dryer Test Data"=w1854, "Off Mode Array"=w1855) -> (w1852:T6)
        n877 = Unbundle By Name(w1849) -> ("Excel Template Path"=w1848:path)
        n878 = local read "FileName DataLog"() -> (w1866:path)
        n879 = call "DPT Create Save Directory.vi"("Pass Fail Lab Eval"=w1847, "error in (no error)"=w1846, "Lab ID"=w1857, "TR Number"=w1858, "FileName DataLog"=w1866) -> ("error out"=w1845:errorcluster, "File Path"=w1853:path)  [unwired: 5 in]
        "Created File Path" <- w1853
        "Error after create directory" <- w1845
        n880 = local read "2015?"() -> (w1868:bool)
        n881 = call "DPT Worksheet DOE Audit.vi"("2015?"=w1868, "Write Form"=TRUE ("Add?")) -> ("2015 array"=w1850:string[][], "String"=w1851:string)  [unwired: 11 in, 1 out]
        "2015 array" <- w1850
        n882 = One Button Dialog(message=w1851) -> ()  [unwired: 1 in, 1 out]
        n883 = call "DPT Save to Excel.vi"("2015 Raw Data"=w1850, "Summary"=w1851, "Pass Fail Lab Eval"=w1847, "error in (no error)"=w1845, "FileInit Cluster"=w1852, "report file path"=w1853, "template (empty)"=w1848) -> ("error out"=w1859:errorcluster, "Error"=→"Error":errorcluster[])  [unwired: 3 in]
        "Error after save to excel" <- w1859
        n884 = call <vilib>:"Add State(s) to Queue__jki_lib_state_machine.vi"("State(s) in (\"\")"=w1870) -> ("States Out"=w1869:string)  [unwired: 14 in]
        "Error before create directory" <- w1846
      }
      frame "Exit" {
        n885 = call <vilib>:"Add State(s) to Queue__jki_lib_state_machine.vi"("State(s) in (\"\")"=w1890) -> ("States Out"=w1889:string)  [unwired: 14 in]
      }
    }
    n886 = local read "Debug Mode"() -> (w1208:bool)
    n887 = case shown="True" w1208 {
      tunnel: w1211 -> [w1221 w1224]
      tunnel: [w1221 w1223] -> w1210
      tunnel: w1209 -> [_ w1222]
      frame False {
      }
      frame True {
        n888 = Build Array (concatenate)(w1224, w1222) -> (w1223:string[])
        "UI States" <- w1223
      }
    }
  }
  n889 = disable-structure shown="Disabled" {
    frame Disabled {
      n890 = event shown="[0] \"Quit\": Value Change" {
        selector: _ -> [_]
        dyn-events: _ -> [_]
        timeout: _ -> [_]
        tunnel: [FALSE ("stop")] -> w1891
        event Value Change {
          w1892 = TRUE ("Exit Nufi")
          n891 = event-data() -> ()  [unwired: 1 in, 5 out]
          n892 = while {
            stop <- w1898 stop-if-true
            n893 = local read "End_End"() -> (w1894:bool)
            n894 = local read "End2_DAQ"() -> (w1897:bool)
            n895 = local read "Eng3_Log"() -> (w1896:bool)
            n896 = Compound Arithmetic op=AND(w1894, w1897, w1896) -> (w1898:bool)
            n897 = Wait (ms)(milliseconds to wait=u32 150) -> ()  [unwired: 1 out]
          }
          n898 = global write "Nufi Global_ReceivedDataCluster.vi" "Exit Nufi"(w1892) -> ()
          n899 = property on="End1_Main" class="Bool (strict)"("Val(Sgnl)"=w1892) -> ()  [unwired: 2 in, 2 out]
        }
      }
      n900 = local write "Quit"(w1891) -> ()
    }
    frame Enabled {
    }
  }
  n901 = disable-structure shown="Disabled" {
    disable-tunnel: w21 -> [w1900 _]
    frame Disabled {
      n902 = flat-sequence {
        tunnel: w1900 -> [w1901]
        tunnel: [w1901] -> w1899
        frame #0 {
          n903 = local read "Final User Message"() -> (w1902:string)
          n904 = One Button Dialog(message=w1902) -> ()  [unwired: 1 in, 1 out]
        }
      }
      "Eng3_Log" <- w1899
    }
    frame Enabled {
    }
  }
  n905 = disable-structure shown="Disabled" {
    frame Disabled {
      # "Sets the Chroma power supply output, and reads the voltages with the WT500 to make sure that the \nPower is in range.\n\nOutputs dryer type to globals.  Tests the voltage settings.  Sets the Supply Voltage output variable."
      n906 = call "UTILITY Delay mS.vi"("milliseconds to wait"=u32 2000) -> ("Error In"=w1910:errorcluster, "Error Out"=w1912:errorcluster)  [unwired: 13 in]
      n907 = call "WT500 Read Power.vi"("WT500 CMDS"=WT500_Sequences."GetReadings", "error in (no error)"=w1912) -> ("VISA resource name"=w1903:refnum<visa-resource-name>, "Measurement Values"=w1904:dbl[], "error out"=w1906:errorcluster)  [unwired: 7 in, 4 out]
      n908 = case shown="\"120\", Default" w1909 {
        tunnel: w1904 -> [w1922 w1931 w1940]
        tunnel: [w1916 w1925 w1934] -> w1907
        frame "240" {
          n909 = Delete From Array(array=w1922, length=2, index=0) -> (deleted portion=w1919:dbl[])  [unwired: 1 out]
          n910 = In Range and Coerce(upper limit=121.2, x=w1919, lower limit=118.8) -> (In Range?=w1915:bool[])  [unwired: 1 out]
          n911 = And Array Elements(Boolean array=w1915) -> (logical AND=w1914:bool)
          n912 = Not(x=w1914) -> (.not. x?=w1916:bool)
        }
        frame "208" {
          n913 = Delete From Array(array=w1931, length=2, index=0) -> (deleted portion=w1928:dbl[])  [unwired: 1 out]
          n914 = In Range and Coerce(upper limit=105.2, x=w1928, lower limit=102.8) -> (In Range?=w1924:bool[])  [unwired: 1 out]
          n915 = And Array Elements(Boolean array=w1924) -> (logical AND=w1923:bool)
          n916 = Not(x=w1923) -> (.not. x?=w1925:bool)
        }
        frame "120", Default {
          n917 = Delete From Array(array=w1940, length=1, index=0) -> (deleted portion=w1937:dbl[])  [unwired: 1 out]
          n918 = In Range and Coerce(upper limit=121.0, x=w1937, lower limit=119.0) -> (In Range?=w1933:bool[])  [unwired: 1 out]
          n919 = And Array Elements(Boolean array=w1933) -> (logical AND=w1932:bool)
          n920 = Not(x=w1932) -> (.not. x?=w1934:bool)
        }
      }
      n921 = call "UTILITY Error Bool Add Message.vi"("Error?"=w1907, "Message"="Power Out of Range", "Error In"=w1906) -> ("Error Out"=w1905:errorcluster)  [unwired: 12 in]
    }
    frame Enabled {
    }
  }
  n922 = flat-sequence {
    tunnel: w8 -> [_]
    tunnel: w7 -> [_]
    tunnel: [w1942] -> w1
    tunnel: w5 -> [w1942]
    frame #0 {
      n923 = call <vilib>:"DAQmx Clear Task.vi"("task in"=refnum<k21> "Weight" ("task/channels in")) -> ("error out"=w1941:errorcluster)  [unwired: 14 in]
      n924 = call <vilib>:"Simple Error Handler.vi"("error in (no error)"=w1941) -> ()  [unwired: 4 in, 5 out]
    }
  }
  n925 = flat-sequence {
    tunnel: w9 -> [w1946]
    tunnel: [w1944] -> w3
    tunnel: w6 -> [w1944]
    frame #0 {
      n926 = Release Queue(queue=w1946, force destroy? (F)=TRUE) -> ()  [unwired: 1 in, 3 out]
    }
  }
  n927 = disable-structure shown="Disabled" {
    disable-tunnel: w3 -> [w1947 _]
    frame Disabled {
      "End2_DAQ" <- w1947
    }
    frame Enabled {
    }
  }
  n928 = disable-structure shown="Disabled" {
    disable-tunnel: w1 -> [w1948 _]
    frame Disabled {
      n929 = property on="Quit" class="Bool (strict)"("Val(Sgnl)"=w1948) -> ()  [unwired: 2 in, 2 out]
      "End_End" <- w1948
    }
    frame Enabled {
    }
  }
